vi "OP_Print_TPS_cluster_20171030.vi"() -> ()   [LabVIEW 2013]
uses:
  <vilib>/addons/database/Connection.llb/DB Tools Open Connec (Path).vi
  <vilib>/addons/database/Connection.llb/Conn Execute.vi
  <vilib>/addons/database/Recordset.llb/Rec Fetch Recordset Data (R).vi
  <vilib>/addons/database/Recordset.llb/Rec Destroy - Connection.vi
  <userlib>/caLab/Private/Get_PV-1D.vi
  <userlib>/caLab/Private/Get_PV.vi
  <vilib>/addons/database/_DB Variant To Data/Database Variant To Data.xnode
  <vilib>/addons/database/NI_Database_API.lvlib
panel:
  out "EVENTs":i32
  out "check loop":i32
  in  "Check period":i32=10 min=0 max=10
  out "Diff list":string[][](array[string])
  out "Program Start Time":dbl=3592021508.642459
  out "dT":u32=325
  out "x > y?":bool
  out "PV list":string[](array[string])=["LI-ES-CPS-01:SETMODE", "LI-ES-CPS-01:PULSEMODE", "LI-ES-BPS-01:SETU:GRID", "LI-ES-BPS-01:SETU:SBM", "LI-ES-BPS-01:SETU:MBM", "LI-RF-CAB-07:SET:MODE", "LI-RF-HVP-11:SET:U", "LI-RF-CAB-09:SET:MODE", "LI-RF-HVP-21:SET:U", "LI-RF-CAB-11:SET:MODE", "LI-RF-HVP-31:SET:U", "LI-RF-WGA-01:SET:POS", "LI-RF-WGA-02:SET:POS", "LI-RF-WGA-03:SET:POS", "LI-RF-SFT-01:SET:POS", "LI-RF-SFT-02:SET:POS", "LI-RF-SFT-03:SET:POS", "LI-RF-CTR-01:ES:SET:DEG", "LI-RF-CTR-01:SP:SET:DEG", "LI-RF-CTR-01:K123:SET:DEG", "LI-RF-CTR-01:K1:SET:DEG", "LI-RF-CTR-01:K3:SET:DEG", "LI-RF-AMP-01:SET:PWR", "LI-RF-AMP-02:SET:PWR", "LI-MA-SPS-01:SET:I", "LI-MA-SPS-02:SET:I", "LI-MA-SPS-03:SET:I", "LI-MA-SPS-04:SET:I", "LI-MA-SPS-05:SET:I", "LI-MA-SPS-06:SET:I", "LI-MA-SPS-07:SET:I", "LI-MA-SPS-08:SET:I", "LI-MA-SPS-09:SET:I", "LI-MA-SPS-10:SET:I", "LI-MA-SPS-11:SET:I", "LI-MA-SPS-12:SET:I", "LI-MA-SPS-13:SET:I", "LI-MA-SPS-14:SET:I", "LI-MA-SPS-15:SET:I", "LI-MA-SPS-16:SET:I", "LI-MA-STP-01:SET:I", "LI-MA-STP-02:SET:I", "LI-MA-STP-03:SET:I", "LI-MA-STP-04:SET:I", "LI-MA-STP-05:SET:I", "LI-MA-STP-06:SET:I", "LI-MA-STP-07:SET:I", "LI-MA-STP-08:SET:I", "LI-MA-STP-09:SET:I", "LI-MA-STP-10:SET:I", "LI-MA-STP-11:SET:I", "LI-MA-STP-12:SET:I", "LI-MA-STP-13:SET:I", "LI-MA-STP-14:SET:I", "LI-MA-STP-15:SET:I", "LI-MA-STP-16:SET:I", "LI-MA-QPS-01:SET:I", "LI-MA-QPS-02:SET:I", "LI-MA-QPS-03:SET:I", "LI-MA-QPS-04:SET:I", "LI-MA-QPS-05:SET:I", "LI-MA-QPS-06:SET:I", "CPCITM-TI-EVRTG:Pulse7DelaySet", "CPCITM-TI-EVRTG:Pulse7WidthSet", "CPCITM-TI-EVRTG:GTX7CtrlGTXPHSet", "CPCITM-TI-EVRTG:GTX7DlySet", "CPCITM-TI-EVRTG:Pulse6DelaySet", "CPCITM-TI-EVRTG:Pulse6WidthSet", "CPCITM-TI-EVRTG:GTX6CtrlGTXPHSet", "CPCITM-TI-EVRTG:GTX6DlySet", "CPCILI-TI-EVR:Pulse2DelaySet", "CPCILI-TI-EVR:Pulse2WidthSet", "CPCILI-TI-EVR:Pulse3DelaySet", "CPCILI-TI-EVR:Pulse3WidthSet", "CPCILI-TI-EVR:Pulse4DelaySet", "CPCILI-TI-EVR:Pulse4WidthSet", "CPCILI-TI-EVR:Pulse5DelaySet", "CPCILI-TI-EVR:Pulse5WidthSet", "CPCILI-TI-EVR:Pulse6DelaySet", "CPCILI-TI-EVR:Pulse6WidthSet", "CPCILI-TI-EVR:Pulse7DelaySet", "CPCILI-TI-EVR:Pulse7WidthSet", "CPCILI-TI-EVR:Pulse8DelaySet", "CPCILI-TI-EVR:Pulse8WidthSet", "CPCILI-TI-EVR:Pulse9DelaySet", "CPCILI-TI-EVR:Pulse9WidthSet", "CPCITM-TI-EVRTG:GTX6DlySet", "CPCITM-TI-EVRTG:GTX7DlySet", "LTB-PS-HC-1:setI", "LTB-PS-HC-2:setI", "LTB-PS-HC-3:setI", "LTB-PS-HC-4:setI", "LTB-PS-HC-5:setI", "LTB-PS-VC-1:setI", "LTB-PS-VC-2:setI", "LTB-PS-VC-3:setI", "LTB-PS-VC-4:setI", "LTB-PS-VC-5:setI", "LTB-PS-VC-6:setI", "LTB-PS-VC-7:setI", "LTB-PS-Q1A:setI", "LTB-PS-Q1B:setI", "LTB-PS-Q1C:setI", "LTB-PS-Q2A:setI", "LTB-PS-Q2B:setI", "LTB-PS-Q2C:setI", "LTB-PS-Q3A:setI", "LTB-PS-Q3B:setI", "LTB-PS-Q4A:setI", "LTB-PS-Q4B:setI", "LTB-PS-QQ:setI", "LTB-PS-BEND-1:setI", "LTB-PS-VC-2a:setI", "LTB-PS-HC-3a:setI", "LTB-PS-HC-3b:setI", "LTB-PS-HC-4a:setI", "LTB-PS-HC-5a:setI", "LI-DI-SLIT-motor:axis2Position1", "LI-DI-SLIT-motor:axis1Position1", "BR-PS-HC-101:setI", "BR-PS-HC-102:setI", "BR-PS-HC-103:setI", "BR-PS-HC-104:setI", "BR-PS-HC-105:setI", "BR-PS-HC-106:setI", "BR-PS-HC-107:setI", "BR-PS-HC-108:setI", "BR-PS-HC-109:setI", "BR-PS-HC-110:setI", "BR-PS-HC-201:setI", "BR-PS-HC-202:setI", "BR-PS-HC-203:setI", "BR-PS-HC-204:setI", "BR-PS-HC-205:setI", "BR-PS-HC-206:setI", "BR-PS-HC-207:setI", "BR-PS-HC-208:setI", "BR-PS-HC-209:setI", "BR-PS-HC-210:setI", "BR-PS-HC-301:setI", "BR-PS-HC-302:setI", "BR-PS-HC-303:setI", "BR-PS-HC-304:setI", "BR-PS-HC-305:setI", "BR-PS-HC-306:setI", "BR-PS-HC-307:setI", "BR-PS-HC-308:setI", "BR-PS-HC-309:setI", "BR-PS-HC-310:setI", "BR-PS-HC-401:setI", "BR-PS-HC-402:setI", "BR-PS-HC-403:setI", "BR-PS-HC-404:setI", "BR-PS-HC-405:setI", "BR-PS-HC-406:setI", "BR-PS-HC-407:setI", "BR-PS-HC-408:setI", "BR-PS-HC-409:setI", "BR-PS-HC-410:setI", "BR-PS-HC-501:setI", "BR-PS-HC-502:setI", "BR-PS-HC-503:setI", "BR-PS-HC-504:setI", "BR-PS-HC-505:setI", "BR-PS-HC-506:setI", "BR-PS-HC-507:setI", "BR-PS-HC-508:setI", "BR-PS-HC-509:setI", "BR-PS-HC-510:setI", "BR-PS-HC-601:setI", "BR-PS-HC-602:setI", "BR-PS-HC-603:setI", "BR-PS-HC-603a:setI", "BR-PS-HC-604:setI", "BR-PS-HC-605:setI", "BR-PS-HC-606:setI", "BR-PS-HC-606a:setI", "BR-PS-HC-607:setI", "BR-PS-HC-608:setI", "BR-PS-HC-609:setI", "BR-PS-HC-610:setI", "BR-PS-VC-101:setI", "BR-PS-VC-102:setI", "BR-PS-VC-103:setI", "BR-PS-VC-104:setI", "BR-PS-VC-105:setI", "BR-PS-VC-106:setI", "BR-PS-VC-201:setI", "BR-PS-VC-202:setI", "BR-PS-VC-203:setI", "BR-PS-VC-204:setI", "BR-PS-VC-205:setI", "BR-PS-VC-206:setI", "BR-PS-VC-301:setI", "BR-PS-VC-302:setI", "BR-PS-VC-303:setI", "BR-PS-VC-304:setI", "BR-PS-VC-305:setI", "BR-PS-VC-306:setI", "BR-PS-VC-401:setI", "BR-PS-VC-402:setI", "BR-PS-VC-403:setI", "BR-PS-VC-404:setI", "BR-PS-VC-405:setI", "BR-PS-VC-406:setI", "BR-PS-VC-501:setI", "BR-PS-VC-502:setI", "BR-PS-VC-503:setI", "BR-PS-VC-504:setI", "BR-PS-VC-505:setI", "BR-PS-VC-506:setI", "BR-PS-VC-601:setI", "BR-PS-VC-602:setI", "BR-PS-VC-602a:setI", "BR-PS-VC-603:setI", "BR-PS-VC-604:setI", "BR-PS-VC-604a:setI", "BR-PS-VC-605:setI", "BR-PS-VC-606:setI", "BR-PS-VC-100a:setI", "BR-PS-SD:setI", "BR-PS-SF:setI", "cpsc_027:AO:SLOW_SET:CH:1", "cpsc_037:AO:SLOW_SET:CH:3", "BR-RF-LLRF:setStationPhase", "TI-INJ-PROC:setTinj", "BR-PS-INJ-SE:setHV", "CPCIPM-TI-EVR:Pulse1DelaySet", "BR-PS-INJ-KI:setHV", "CPCIPM-TI-EVR:Pulse2DelaySet", "BR-PS-QF:setWfDC", "BR-PS-QM:setWfDC", "BR-PS-Q1:setWfDC", "BR-PS-Q2:setWfDC", "BR-PS-BEND:setWfDC", "BTS-PS-HC-1:setI", "BTS-PS-HC-2:setI", "BTS-PS-HC-3:setI", "BTS-PS-HC-4:setI", "BTS-PS-HC-5:setI", "BTS-PS-VC-2:setI", "BTS-PS-VC-3:setI", "BTS-PS-VC-4:setI", "BTS-PS-VC-5:setI", "BTS-PS-VC-6:setI", "BTS-PS-Q1A:setI", "BTS-PS-Q1B:setI", "BTS-PS-Q1C:setI", "BTS-PS-Q2A:setI", "BTS-PS-Q2B:setI", "BTS-PS-Q2C:setI", "BTS-PS-Q3A:setI", "BTS-PS-BEND-1:setI", "BTS-PS-BEND-2:setI", "BR-PS-EXT-K1:setHV", "BR-PS-EXT-K2:setHV", "SR-PS-INJ-SE1:setHV", "SR-PS-INJ-SE2:setHV", "SR-PS-INJ-K1:setHV", "SR-PS-INJ-K2:setHV", "SR-PS-INJ-K3:setHV", "SR-PS-INJ-K4:setHV", "CPCIPM-TI-EVR:Pulse4DelaySet", "CPCIPM-TI-EVR:Pulse5DelaySet", "CPCIPM-TI-EVR:Pulse3DelaySet", "CPCIPM-TI-EVR:Pulse6DelaySet", "CPCIPM-TI-EVR:Pulse7DelaySet", "T560:setADelay", "T560:setBDelay", "T560:setCDelay", "T560:setDDelay", "CPCIPM-TI-EVR:Pulse4DelaySet", "CPCIPM-TI-EVR:Pulse5DelaySet", "BR-PS-EXT-SE1:setHV", "BR-PS-EXT-SE2:setHV", "CPCIPM-TI-EVR:Pulse3DelaySet", "CPCIPM-TI-EVR:Pulse11DelaySet", "SR-PS-BEND:setI", "SR-PS-HC-011:setI", "SR-PS-HC-012:setI", "SR-PS-HC-013:setI", "SR-PS-HC-014:setI", "SR-PS-HC-015:setI", "SR-PS-HC-016:setI", "SR-PS-HC-017:setI", "SR-PS-HC-021:setI", "SR-PS-HC-022:setI", "SR-PS-HC-023:setI", "SR-PS-HC-024:setI", "SR-PS-HC-025:setI", "SR-PS-HC-026:setI", "SR-PS-HC-027:setI", "SR-PS-HC-031:setI", "SR-PS-HC-032:setI", "SR-PS-HC-033:setI", "SR-PS-HC-034:setI", "SR-PS-HC-035:setI", "SR-PS-HC-036:setI", "SR-PS-HC-037:setI", "SR-PS-HC-041:setI", "SR-PS-HC-042:setI", "SR-PS-HC-043:setI", "SR-PS-HC-044:setI", "SR-PS-HC-045:setI", "SR-PS-HC-046:setI", "SR-PS-HC-047:setI", "SR-PS-HC-051:setI", "SR-PS-HC-052:setI", "SR-PS-HC-053:setI", "SR-PS-HC-054:setI", "SR-PS-HC-055:setI", "SR-PS-HC-056:setI", "SR-PS-HC-057:setI", "SR-PS-HC-061:setI", "SR-PS-HC-062:setI", "SR-PS-HC-063:setI", "SR-PS-HC-064:setI", "SR-PS-HC-065:setI", "SR-PS-HC-066:setI", "SR-PS-HC-067:setI", "SR-PS-HC-071:setI", "SR-PS-HC-072:setI", "SR-PS-HC-073:setI", "SR-PS-HC-074:setI", "SR-PS-HC-075:setI", "SR-PS-HC-076:setI", "SR-PS-HC-077:setI", "SR-PS-HC-081:setI", "SR-PS-HC-082:setI", "SR-PS-HC-083:setI", "SR-PS-HC-084:setI", "SR-PS-HC-085:setI", "SR-PS-HC-086:setI", "SR-PS-HC-087:setI", "SR-PS-HC-091:setI", "SR-PS-HC-092:setI", "SR-PS-HC-093:setI", "SR-PS-HC-094:setI", "SR-PS-HC-095:setI", "SR-PS-HC-096:setI", "SR-PS-HC-097:setI", "SR-PS-HC-101:setI", "SR-PS-HC-102:setI", "SR-PS-HC-103:setI", "SR-PS-HC-104:setI", "SR-PS-HC-105:setI", "SR-PS-HC-106:setI", "SR-PS-HC-107:setI", "SR-PS-HC-111:setI", "SR-PS-HC-112:setI", "SR-PS-HC-113:setI", "SR-PS-HC-114:setI", "SR-PS-HC-115:setI", "SR-PS-HC-116:setI", "SR-PS-HC-117:setI", "SR-PS-HC-121:setI", "SR-PS-HC-122:setI", "SR-PS-HC-123:setI", "SR-PS-HC-124:setI", "SR-PS-HC-125:setI", "SR-PS-HC-126:setI", "SR-PS-HC-127:setI", "SR-PS-HC-131:setI", "SR-PS-HC-132:setI", "SR-PS-HC-133:setI", "SR-PS-HC-134:setI", "SR-PS-HC-135:setI", "SR-PS-HC-136:setI", "SR-PS-HC-137:setI", "SR-PS-HC-141:setI", "SR-PS-HC-142:setI", "SR-PS-HC-143:setI", "SR-PS-HC-144:setI", "SR-PS-HC-145:setI", "SR-PS-HC-146:setI", "SR-PS-HC-147:setI", "SR-PS-HC-151:setI", "SR-PS-HC-152:setI", "SR-PS-HC-153:setI", "SR-PS-HC-154:setI", "SR-PS-HC-155:setI", "SR-PS-HC-156:setI", "SR-PS-HC-157:setI", "SR-PS-HC-161:setI", "SR-PS-HC-162:setI", "SR-PS-HC-163:setI", "SR-PS-HC-164:setI", "SR-PS-HC-165:setI", "SR-PS-HC-166:setI", "SR-PS-HC-167:setI", "SR-PS-HC-171:setI", "SR-PS-HC-172:setI", "SR-PS-HC-173:setI", "SR-PS-HC-174:setI", "SR-PS-HC-175:setI", "SR-PS-HC-176:setI", "SR-PS-HC-177:setI", "SR-PS-HC-181:setI", "SR-PS-HC-182:setI", "SR-PS-HC-183:setI", "SR-PS-HC-184:setI", "SR-PS-HC-185:setI", "SR-PS-HC-186:setI", "SR-PS-HC-187:setI", "SR-PS-HC-191:setI", "SR-PS-HC-192:setI", "SR-PS-HC-193:setI", "SR-PS-HC-194:setI", "SR-PS-HC-195:setI", "SR-PS-HC-196:setI", "SR-PS-HC-197:setI", "SR-PS-HC-201:setI", "SR-PS-HC-202:setI", "SR-PS-HC-203:setI", "SR-PS-HC-204:setI", "SR-PS-HC-205:setI", "SR-PS-HC-206:setI", "SR-PS-HC-207:setI", "SR-PS-HC-211:setI", "SR-PS-HC-212:setI", "SR-PS-HC-213:setI", "SR-PS-HC-214:setI", "SR-PS-HC-215:setI", "SR-PS-HC-216:setI", "SR-PS-HC-217:setI", "SR-PS-HC-221:setI", "SR-PS-HC-222:setI", "SR-PS-HC-223:setI", "SR-PS-HC-224:setI", "SR-PS-HC-225:setI", "SR-PS-HC-226:setI", "SR-PS-HC-227:setI", "SR-PS-HC-231:setI", "SR-PS-HC-232:setI", "SR-PS-HC-233:setI", "SR-PS-HC-234:setI", "SR-PS-HC-235:setI", "SR-PS-HC-236:setI", "SR-PS-HC-237:setI", "SR-PS-HC-241:setI", "SR-PS-HC-242:setI", "SR-PS-HC-243:setI", "SR-PS-HC-244:setI", "SR-PS-HC-245:setI", "SR-PS-HC-246:setI", "SR-PS-HC-247:setI", "SR-PS-VC-011:setI", "SR-PS-VC-012:setI", "SR-PS-VC-013:setI", "SR-PS-VC-014:setI", "SR-PS-VC-015:setI", "SR-PS-VC-016:setI", "SR-PS-VC-017:setI", "SR-PS-VC-021:setI", "SR-PS-VC-022:setI", "SR-PS-VC-023:setI", "SR-PS-VC-024:setI", "SR-PS-VC-025:setI", "SR-PS-VC-026:setI", "SR-PS-VC-027:setI", "SR-PS-VC-031:setI", "SR-PS-VC-032:setI", "SR-PS-VC-033:setI", "SR-PS-VC-034:setI", "SR-PS-VC-035:setI", "SR-PS-VC-036:setI", "SR-PS-VC-037:setI", "SR-PS-VC-041:setI", "SR-PS-VC-042:setI", "SR-PS-VC-043:setI", "SR-PS-VC-044:setI", "SR-PS-VC-045:setI", "SR-PS-VC-046:setI", "SR-PS-VC-047:setI", "SR-PS-VC-051:setI", "SR-PS-VC-052:setI", "SR-PS-VC-053:setI", "SR-PS-VC-054:setI", "SR-PS-VC-055:setI", "SR-PS-VC-056:setI", "SR-PS-VC-057:setI", "SR-PS-VC-061:setI", "SR-PS-VC-062:setI", "SR-PS-VC-063:setI", "SR-PS-VC-064:setI", "SR-PS-VC-065:setI", "SR-PS-VC-066:setI", "SR-PS-VC-067:setI", "SR-PS-VC-071:setI", "SR-PS-VC-072:setI", "SR-PS-VC-073:setI", "SR-PS-VC-074:setI", "SR-PS-VC-075:setI", "SR-PS-VC-076:setI", "SR-PS-VC-077:setI", "SR-PS-VC-081:setI", "SR-PS-VC-082:setI", "SR-PS-VC-083:setI", "SR-PS-VC-084:setI", "SR-PS-VC-085:setI", "SR-PS-VC-086:setI", "SR-PS-VC-087:setI", "SR-PS-VC-091:setI", "SR-PS-VC-092:setI", "SR-PS-VC-093:setI", "SR-PS-VC-094:setI", "SR-PS-VC-095:setI", "SR-PS-VC-096:setI", "SR-PS-VC-097:setI", "SR-PS-VC-101:setI", "SR-PS-VC-102:setI", "SR-PS-VC-103:setI", "SR-PS-VC-104:setI", "SR-PS-VC-105:setI", "SR-PS-VC-106:setI", "SR-PS-VC-107:setI", "SR-PS-VC-111:setI", "SR-PS-VC-112:setI", "SR-PS-VC-113:setI", "SR-PS-VC-114:setI", "SR-PS-VC-115:setI", "SR-PS-VC-116:setI", "SR-PS-VC-117:setI", "SR-PS-VC-121:setI", "SR-PS-VC-122:setI", "SR-PS-VC-123:setI", "SR-PS-VC-124:setI", "SR-PS-VC-125:setI", "SR-PS-VC-126:setI", "SR-PS-VC-127:setI", "SR-PS-VC-131:setI", "SR-PS-VC-132:setI", "SR-PS-VC-133:setI", "SR-PS-VC-134:setI", "SR-PS-VC-135:setI", "SR-PS-VC-136:setI", "SR-PS-VC-137:setI", "SR-PS-VC-141:setI", "SR-PS-VC-142:setI", "SR-PS-VC-143:setI", "SR-PS-VC-144:setI", "SR-PS-VC-145:setI", "SR-PS-VC-146:setI", "SR-PS-VC-147:setI", "SR-PS-VC-151:setI", "SR-PS-VC-152:setI", "SR-PS-VC-153:setI", "SR-PS-VC-154:setI", "SR-PS-VC-155:setI", "SR-PS-VC-156:setI", "SR-PS-VC-157:setI", "SR-PS-VC-161:setI", "SR-PS-VC-162:setI", "SR-PS-VC-163:setI", "SR-PS-VC-164:setI", "SR-PS-VC-165:setI", "SR-PS-VC-166:setI", "SR-PS-VC-167:setI", "SR-PS-VC-171:setI", "SR-PS-VC-172:setI", "SR-PS-VC-173:setI", "SR-PS-VC-174:setI", "SR-PS-VC-175:setI", "SR-PS-VC-176:setI", "SR-PS-VC-177:setI", "SR-PS-VC-181:setI", "SR-PS-VC-182:setI", "SR-PS-VC-183:setI", "SR-PS-VC-184:setI", "SR-PS-VC-185:setI", "SR-PS-VC-186:setI", "SR-PS-VC-187:setI", "SR-PS-VC-191:setI", "SR-PS-VC-192:setI", "SR-PS-VC-193:setI", "SR-PS-VC-194:setI", "SR-PS-VC-195:setI", "SR-PS-VC-196:setI", "SR-PS-VC-197:setI", "SR-PS-VC-201:setI", "SR-PS-VC-202:setI", "SR-PS-VC-203:setI", "SR-PS-VC-204:setI", "SR-PS-VC-205:setI", "SR-PS-VC-206:setI", "SR-PS-VC-207:setI", "SR-PS-VC-211:setI", "SR-PS-VC-212:setI", "SR-PS-VC-213:setI", "SR-PS-VC-214:setI", "SR-PS-VC-215:setI", "SR-PS-VC-216:setI", "SR-PS-VC-217:setI", "SR-PS-VC-221:setI", "SR-PS-VC-222:setI", "SR-PS-VC-223:setI", "SR-PS-VC-224:setI", "SR-PS-VC-225:setI", "SR-PS-VC-226:setI", "SR-PS-VC-227:setI", "SR-PS-VC-231:setI", "SR-PS-VC-232:setI", "SR-PS-VC-233:setI", "SR-PS-VC-234:setI", "SR-PS-VC-235:setI", "SR-PS-VC-236:setI", "SR-PS-VC-237:setI", "SR-PS-VC-241:setI", "SR-PS-VC-242:setI", "SR-PS-VC-243:setI", "SR-PS-VC-244:setI", "SR-PS-VC-245:setI", "SR-PS-VC-246:setI", "SR-PS-VC-247:setI", "SR-PS-QL1-0101:setI", "SR-PS-QL2-0102:setI", "SR-PS-QL3-0103:setI", "SR-PS-QS4-0104:setI", "SR-PS-QS5-0105:setI", "SR-PS-QS5-0106:setI", "SR-PS-QS4-0107:setI", "SR-PS-QS3-0108:setI", "SR-PS-QS2-0109:setI", "SR-PS-QS1-0110:setI", "SR-PS-QS1-0201:setI", "SR-PS-QS2-0202:setI", "SR-PS-QS3-0203:setI", "SR-PS-QS4-0204:setI", "SR-PS-QS5-0205:setI", "SR-PS-QS5-0206:setI", "SR-PS-QS4-0207:setI", "SR-PS-QS3-0208:setI", "SR-PS-QS2-0209:setI", "SR-PS-QS1-0210:setI", "SR-PS-QS1-0301:setI", "SR-PS-QS2-0302:setI", "SR-PS-QS3-0303:setI", "SR-PS-QS4-0304:setI", "SR-PS-QS5-0305:setI", "SR-PS-QS5-0306:setI", "SR-PS-QS4-0307:setI", "SR-PS-QS3-0308:setI", "SR-PS-QS2-0309:setI", "SR-PS-QS1-0310:setI", "SR-PS-QS1-0401:setI", "SR-PS-QS2-0402:setI", "SR-PS-QS3-0403:setI", "SR-PS-QS4-0404:setI", "SR-PS-QS5-0405:setI", "SR-PS-QS5-0406:setI", "SR-PS-QS4-0407:setI", "SR-PS-QL3-0408:setI", "SR-PS-QL2-0409:setI", "SR-PS-QL1-0410:setI", "SR-PS-QL1-0501:setI", "SR-PS-QL2-0502:setI", "SR-PS-QL3-0503:setI", "SR-PS-QS4-0504:setI", "SR-PS-QS5-0505:setI", "SR-PS-QS5-0506:setI", "SR-PS-QS4-0507:setI", "SR-PS-QS3-0508:setI", "SR-PS-QS2-0509:setI", "SR-PS-QS1-0510:setI", "SR-PS-QS1-0601:setI", "SR-PS-QS2-0602:setI", "SR-PS-QS3-0603:setI", "SR-PS-QS4-0604:setI", "SR-PS-QS5-0605:setI", "SR-PS-QS5-0606:setI", "SR-PS-QS4-0607:setI", "SR-PS-QS3-0608:setI", "SR-PS-QS2-0609:setI", "SR-PS-QS1-0610:setI", "SR-PS-QS1-0701:setI", "SR-PS-QS2-0702:setI", "SR-PS-QS3-0703:setI", "SR-PS-QS4-0704:setI", "SR-PS-QS5-0705:setI", "SR-PS-QS5-0706:setI", "SR-PS-QS4-0707:setI", "SR-PS-QS3-0708:setI", "SR-PS-QS2-0709:setI", "SR-PS-QS1-0710:setI", "SR-PS-QS1-0801:setI", "SR-PS-QS2-0802:setI", "SR-PS-QS3-0803:setI", "SR-PS-QS4-0804:setI", "SR-PS-QS5-0805:setI", "SR-PS-QS5-0806:setI", "SR-PS-QS4-0807:setI", "SR-PS-QL3-0808:setI", "SR-PS-QL2-0809:setI", "SR-PS-QL1-0810:setI", "SR-PS-QL1-0901:setI", "SR-PS-QL2-0902:setI", "SR-PS-QL3-0903:setI", "SR-PS-QS4-0904:setI", "SR-PS-QS5-0905:setI", "SR-PS-QS5-0906:setI", "SR-PS-QS4-0907:setI", "SR-PS-QS3-0908:setI", "SR-PS-QS2-0909:setI", "SR-PS-QS1-0910:setI", "SR-PS-QS1-1001:setI", "SR-PS-QS2-1002:setI", "SR-PS-QS3-1003:setI", "SR-PS-QS4-1004:setI", "SR-PS-QS5-1005:setI", "SR-PS-QS5-1006:setI", "SR-PS-QS4-1007:setI", "SR-PS-QS3-1008:setI", "SR-PS-QS2-1009:setI", "SR-PS-QS1-1010:setI", "SR-PS-QS1-1101:setI", "SR-PS-QS2-1102:setI", "SR-PS-QS3-1103:setI", "SR-PS-QS4-1104:setI", "SR-PS-QS5-1105:setI", "SR-PS-QS5-1106:setI", "SR-PS-QS4-1107:setI", "SR-PS-QS3-1108:setI", "SR-PS-QS2-1109:setI", "SR-PS-QS1-1110:setI", "SR-PS-QS1-1201:setI", "SR-PS-QS2-1202:setI", "SR-PS-QS3-1203:setI", "SR-PS-QS4-1204:setI", "SR-PS-QS5-1205:setI", "SR-PS-QS5-1206:setI", "SR-PS-QS4-1207:setI", "SR-PS-QL3-1208:setI", "SR-PS-QL2-1209:setI", "SR-PS-QL1-1210:setI", "SR-PS-QL1-1301:setI", "SR-PS-QL2-1302:setI", "SR-PS-QL3-1303:setI", "SR-PS-QS4-1304:setI", "SR-PS-QS5-1305:setI", "SR-PS-QS5-1306:setI", "SR-PS-QS4-1307:setI", "SR-PS-QS3-1308:setI", "SR-PS-QS2-1309:setI", "SR-PS-QS1-1310:setI", "SR-PS-QS1-1401:setI", "SR-PS-QS2-1402:setI", "SR-PS-QS3-1403:setI", "SR-PS-QS4-1404:setI", "SR-PS-QS5-1405:setI", "SR-PS-QS5-1406:setI", "SR-PS-QS4-1407:setI", "SR-PS-QS3-1408:setI", "SR-PS-QS2-1409:setI", "SR-PS-QS1-1410:setI", "SR-PS-QS1-1501:setI", "SR-PS-QS2-1502:setI", "SR-PS-QS3-1503:setI", "SR-PS-QS4-1504:setI", "SR-PS-QS5-1505:setI", "SR-PS-QS5-1506:setI", "SR-PS-QS4-1507:setI", "SR-PS-QS3-1508:setI", "SR-PS-QS2-1509:setI", "SR-PS-QS1-1510:setI", "SR-PS-QS1-1601:setI", "SR-PS-QS2-1602:setI", "SR-PS-QS3-1603:setI", "SR-PS-QS4-1604:setI", "SR-PS-QS5-1605:setI", "SR-PS-QS5-1606:setI", "SR-PS-QS4-1607:setI", "SR-PS-QL3-1608:setI", "SR-PS-QL2-1609:setI", "SR-PS-QL1-1610:setI", "SR-PS-QL1-1701:setI", "SR-PS-QL2-1702:setI", "SR-PS-QL3-1703:setI", "SR-PS-QS4-1704:setI", "SR-PS-QS5-1705:setI", "SR-PS-QS5-1706:setI", "SR-PS-QS4-1707:setI", "SR-PS-QS3-1708:setI", "SR-PS-QS2-1709:setI", "SR-PS-QS1-1710:setI", "SR-PS-QS1-1801:setI", "SR-PS-QS2-1802:setI", "SR-PS-QS3-1803:setI", "SR-PS-QS4-1804:setI", "SR-PS-QS5-1805:setI", "SR-PS-QS5-1806:setI", "SR-PS-QS4-1807:setI", "SR-PS-QS3-1808:setI", "SR-PS-QS2-1809:setI", "SR-PS-QS1-1810:setI", "SR-PS-QS1-1901:setI", "SR-PS-QS2-1902:setI", "SR-PS-QS3-1903:setI", "SR-PS-QS4-1904:setI", "SR-PS-QS5-1905:setI", "SR-PS-QS5-1906:setI", "SR-PS-QS4-1907:setI", "SR-PS-QS3-1908:setI", "SR-PS-QS2-1909:setI", "SR-PS-QS1-1910:setI", "SR-PS-QS1-2001:setI", "SR-PS-QS2-2002:setI", "SR-PS-QS3-2003:setI", "SR-PS-QS4-2004:setI", "SR-PS-QS5-2005:setI", "SR-PS-QS5-2006:setI", "SR-PS-QS4-2007:setI", "SR-PS-QL3-2008:setI", "SR-PS-QL2-2009:setI", "SR-PS-QL1-2010:setI", "SR-PS-QL1-2101:setI", "SR-PS-QL2-2102:setI", "SR-PS-QL3-2103:setI", "SR-PS-QS4-2104:setI", "SR-PS-QS5-2105:setI", "SR-PS-QS5-2106:setI", "SR-PS-QS4-2107:setI", "SR-PS-QS3-2108:setI", "SR-PS-QS2-2109:setI", "SR-PS-QS1-2110:setI", "SR-PS-QS1-2201:setI", "SR-PS-QS2-2202:setI", "SR-PS-QS3-2203:setI", "SR-PS-QS4-2204:setI", "SR-PS-QS5-2205:setI", "SR-PS-QS5-2206:setI", "SR-PS-QS4-2207:setI", "SR-PS-QS3-2208:setI", "SR-PS-QS2-2209:setI", "SR-PS-QS1-2210:setI", "SR-PS-QS1-2301:setI", "SR-PS-QS2-2302:setI", "SR-PS-QS3-2303:setI", "SR-PS-QS4-2304:setI", "SR-PS-QS5-2305:setI", "SR-PS-QS5-2306:setI", "SR-PS-QS4-2307:setI", "SR-PS-QS3-2308:setI", "SR-PS-QS2-2309:setI", "SR-PS-QS1-2310:setI", "SR-PS-QS1-2401:setI", "SR-PS-QS2-2402:setI", "SR-PS-QS3-2403:setI", "SR-PS-QS4-2404:setI", "SR-PS-QS5-2405:setI", "SR-PS-QS5-2406:setI", "SR-PS-QS4-2407:setI", "SR-PS-QL3-2408:setI", "SR-PS-QL2-2409:setI", "SR-PS-QL1-2410:setI", "SR-PS-S1-011:setI", "SR-PS-S2-012:setI", "SR-PS-SD-013:setI", "SR-PS-SF-014:setI", "SR-PS-SD-015:setI", "SR-PS-S4-016:setI", "SR-PS-S3-017:setI", "SR-PS-S5-021:setI", "SR-PS-S6-022:setI", "SR-PS-SD-023:setI", "SR-PS-SF-024:setI", "SR-PS-SD-025:setI", "SR-PS-S6-026:setI", "SR-PS-S5-027:setI", "SR-PS-S5-031:setI", "SR-PS-S6-032:setI", "SR-PS-SD-033:setI", "SR-PS-SF-034:setI", "SR-PS-SD-035:setI", "SR-PS-S6-036:setI", "SR-PS-S5-037:setI", "SR-PS-S3-041:setI", "SR-PS-S4-042:setI", "SR-PS-SD-043:setI", "SR-PS-SF-044:setI", "SR-PS-SD-045:setI", "SR-PS-S2-046:setI", "SR-PS-S1-047:setI", "SR-PS-S1-051:setI", "SR-PS-S2-052:setI", "SR-PS-SD-053:setI", "SR-PS-SF-054:setI", "SR-PS-SD-055:setI", "SR-PS-S4-056:setI", "SR-PS-S3-057:setI", "SR-PS-S5-061:setI", "SR-PS-S6-062:setI", "SR-PS-SD-063:setI", "SR-PS-SF-064:setI", "SR-PS-SD-065:setI", "SR-PS-S6-066:setI", "SR-PS-S5-067:setI", "SR-PS-S5-071:setI", "SR-PS-S6-072:setI", "SR-PS-SD-073:setI", "SR-PS-SF-074:setI", "SR-PS-SD-075:setI", "SR-PS-S6-076:setI", "SR-PS-S5-077:setI", "SR-PS-S3-081:setI", "SR-PS-S4-082:setI", "SR-PS-SD-083:setI", "SR-PS-SF-084:setI", "SR-PS-SD-085:setI", "SR-PS-S2-086:setI", "SR-PS-S1-087:setI", "SR-PS-S1-091:setI", "SR-PS-S2-092:setI", "SR-PS-SD-093:setI", "SR-PS-SF-094:setI", "SR-PS-SD-095:setI", "SR-PS-S4-096:setI", "SR-PS-S3-097:setI", "SR-PS-S5-101:setI", "SR-PS-S6-102:setI", "SR-PS-SD-103:setI", "SR-PS-SF-104:setI", "SR-PS-SD-105:setI", "SR-PS-S6-106:setI", "SR-PS-S5-107:setI", "SR-PS-S5-111:setI", "SR-PS-S6-112:setI", "SR-PS-SD-113:setI", "SR-PS-SF-114:setI", "SR-PS-SD-115:setI", "SR-PS-S6-116:setI", "SR-PS-S5-117:setI", "SR-PS-S3-121:setI", "SR-PS-S4-122:setI", "SR-PS-SD-123:setI", "SR-PS-SF-124:setI", "SR-PS-SD-125:setI", "SR-PS-S2-126:setI", "SR-PS-S1-127:setI", "SR-PS-S1-131:setI", "SR-PS-S2-132:setI", "SR-PS-SD-133:setI", "SR-PS-SF-134:setI", "SR-PS-SD-135:setI", "SR-PS-S4-136:setI", "SR-PS-S3-137:setI", "SR-PS-S5-141:setI", "SR-PS-S6-142:setI", "SR-PS-SD-143:setI", "SR-PS-SF-144:setI", "SR-PS-SD-145:setI", "SR-PS-S6-146:setI", "SR-PS-S5-147:setI", "SR-PS-S5-151:setI", "SR-PS-S6-152:setI", "SR-PS-SD-153:setI", "SR-PS-SF-154:setI", "SR-PS-SD-155:setI", "SR-PS-S6-156:setI", "SR-PS-S5-157:setI", "SR-PS-S3-161:setI", "SR-PS-S4-162:setI", "SR-PS-SD-163:setI", "SR-PS-SF-164:setI", "SR-PS-SD-165:setI", "SR-PS-S2-166:setI", "SR-PS-S1-167:setI", "SR-PS-S1-171:setI", "SR-PS-S2-172:setI", "SR-PS-SD-173:setI", "SR-PS-SF-174:setI", "SR-PS-SD-175:setI", "SR-PS-S4-176:setI", "SR-PS-S3-177:setI", "SR-PS-S5-181:setI", "SR-PS-S6-182:setI", "SR-PS-SD-183:setI", "SR-PS-SF-184:setI", "SR-PS-SD-185:setI", "SR-PS-S6-186:setI", "SR-PS-S5-187:setI", "SR-PS-S5-191:setI", "SR-PS-S6-192:setI", "SR-PS-SD-193:setI", "SR-PS-SF-194:setI", "SR-PS-SD-195:setI", "SR-PS-S6-196:setI", "SR-PS-S5-197:setI", "SR-PS-S3-201:setI", "SR-PS-S4-202:setI", "SR-PS-SD-203:setI", "SR-PS-SF-204:setI", "SR-PS-SD-205:setI", "SR-PS-S2-206:setI", "SR-PS-S1-207:setI", "SR-PS-S1-211:setI", "SR-PS-S2-212:setI", "SR-PS-SD-213:setI", "SR-PS-SF-214:setI", "SR-PS-SD-215:setI", "SR-PS-S4-216:setI", "SR-PS-S3-217:setI", "SR-PS-S5-221:setI", "SR-PS-S6-222:setI", "SR-PS-SD-223:setI", "SR-PS-SF-224:setI", "SR-PS-SD-225:setI", "SR-PS-S6-226:setI", "SR-PS-S5-227:setI", "SR-PS-S5-231:setI", "SR-PS-S6-232:setI", "SR-PS-SD-233:setI", "SR-PS-SF-234:setI", "SR-PS-SD-235:setI", "SR-PS-S6-236:setI", "SR-PS-S5-237:setI", "SR-PS-S3-241:setI", "SR-PS-S4-242:setI", "SR-PS-SD-243:setI", "SR-PS-SF-244:setI", "SR-PS-SD-245:setI", "SR-PS-S2-246:setI", "SR-PS-S1-247:setI", "SR-PS-SKEW-011:setI", "SR-PS-SKEW-012:setI", "SR-PS-SKEW-013:setI", "SR-PS-SKEW-014:setI", "SR-PS-SKEW-015:setI", "SR-PS-SKEW-016:setI", "SR-PS-SKEW-017:setI", "SR-PS-SKEW-021:setI", "SR-PS-SKEW-022:setI", "SR-PS-SKEW-023:setI", "SR-PS-SKEW-024:setI", "SR-PS-SKEW-025:setI", "SR-PS-SKEW-026:setI", "SR-PS-SKEW-027:setI", "SR-PS-SKEW-031:setI", "SR-PS-SKEW-032:setI", "SR-PS-SKEW-033:setI", "SR-PS-SKEW-034:setI", "SR-PS-SKEW-035:setI", "SR-PS-SKEW-036:setI", "SR-PS-SKEW-037:setI", "SR-PS-SKEW-041:setI", "SR-PS-SKEW-042:setI", "SR-PS-SKEW-043:setI", "SR-PS-SKEW-044:setI", "SR-PS-SKEW-045:setI", "SR-PS-SKEW-046:setI", "SR-PS-SKEW-047:setI", "SR-PS-SKEW-051:setI", "SR-PS-SKEW-052:setI", "SR-PS-SKEW-053:setI", "SR-PS-SKEW-054:setI", "SR-PS-SKEW-055:setI", "SR-PS-SKEW-056:setI", "SR-PS-SKEW-057:setI", "SR-PS-SKEW-061:setI", "SR-PS-SKEW-062:setI", "SR-PS-SKEW-063:setI", "SR-PS-SKEW-064:setI", "SR-PS-SKEW-065:setI", "SR-PS-SKEW-066:setI", "SR-PS-SKEW-067:setI", "SR-PS-SKEW-071:setI", "SR-PS-SKEW-072:setI", "SR-PS-SKEW-073:setI", "SR-PS-SKEW-074:setI", "SR-PS-SKEW-075:setI", "SR-PS-SKEW-076:setI", "SR-PS-SKEW-077:setI", "SR-PS-SKEW-081:setI", "SR-PS-SKEW-082:setI", "SR-PS-SKEW-083:setI", "SR-PS-SKEW-084:setI", "SR-PS-SKEW-085:setI", "SR-PS-SKEW-086:setI", "SR-PS-SKEW-087:setI", "SR-PS-SKEW-091:setI", "SR-PS-SKEW-092:setI", "SR-PS-SKEW-093:setI", "SR-PS-SKEW-094:setI", "SR-PS-SKEW-095:setI", "SR-PS-SKEW-096:setI", "SR-PS-SKEW-097:setI", "SR-PS-SKEW-101:setI", "SR-PS-SKEW-102:setI", "SR-PS-SKEW-103:setI", "SR-PS-SKEW-104:setI", "SR-PS-SKEW-105:setI", "SR-PS-SKEW-106:setI", "SR-PS-SKEW-107:setI", "SR-PS-SKEW-111:setI", "SR-PS-SKEW-112:setI", "SR-PS-SKEW-113:setI", "SR-PS-SKEW-114:setI", "SR-PS-SKEW-115:setI", "SR-PS-SKEW-116:setI", "SR-PS-SKEW-117:setI", "SR-PS-SKEW-121:setI", "SR-PS-SKEW-122:setI", "SR-PS-SKEW-123:setI", "SR-PS-SKEW-124:setI", "SR-PS-SKEW-125:setI", "SR-PS-SKEW-126:setI", "SR-PS-SKEW-127:setI", "SR-PS-SKEW-131:setI", "SR-PS-SKEW-132:setI", "SR-PS-SKEW-133:setI", "SR-PS-SKEW-134:setI", "SR-PS-SKEW-135:setI", "SR-PS-SKEW-136:setI", "SR-PS-SKEW-137:setI", "SR-PS-SKEW-141:setI", "SR-PS-SKEW-142:setI", "SR-PS-SKEW-143:setI", "SR-PS-SKEW-144:setI", "SR-PS-SKEW-145:setI", "SR-PS-SKEW-146:setI", "SR-PS-SKEW-147:setI", "SR-PS-SKEW-151:setI", "SR-PS-SKEW-152:setI", "SR-PS-SKEW-153:setI", "SR-PS-SKEW-154:setI", "SR-PS-SKEW-155:setI", "SR-PS-SKEW-156:setI", "SR-PS-SKEW-157:setI", "SR-PS-SKEW-161:setI", "SR-PS-SKEW-162:setI", "SR-PS-SKEW-163:setI", "SR-PS-SKEW-164:setI", "SR-PS-SKEW-165:setI", "SR-PS-SKEW-166:setI", "SR-PS-SKEW-167:setI", "SR-PS-SKEW-171:setI", "SR-PS-SKEW-172:setI", "SR-PS-SKEW-173:setI", "SR-PS-SKEW-174:setI", "SR-PS-SKEW-175:setI", "SR-PS-SKEW-176:setI", "SR-PS-SKEW-177:setI", "SR-PS-SKEW-181:setI", "SR-PS-SKEW-182:setI", "SR-PS-SKEW-183:setI", "SR-PS-SKEW-184:setI", "SR-PS-SKEW-185:setI", "SR-PS-SKEW-186:setI", "SR-PS-SKEW-187:setI", "SR-PS-SKEW-191:setI", "SR-PS-SKEW-192:setI", "SR-PS-SKEW-193:setI", "SR-PS-SKEW-194:setI", "SR-PS-SKEW-195:setI", "SR-PS-SKEW-196:setI", "SR-PS-SKEW-197:setI", "SR-PS-SKEW-201:setI", "SR-PS-SKEW-202:setI", "SR-PS-SKEW-203:setI", "SR-PS-SKEW-204:setI", "SR-PS-SKEW-205:setI", "SR-PS-SKEW-206:setI", "SR-PS-SKEW-207:setI", "SR-PS-SKEW-211:setI", "SR-PS-SKEW-212:setI", "SR-PS-SKEW-213:setI", "SR-PS-SKEW-214:setI", "SR-PS-SKEW-215:setI", "SR-PS-SKEW-216:setI", "SR-PS-SKEW-217:setI", "SR-PS-SKEW-221:setI", "SR-PS-SKEW-222:setI", "SR-PS-SKEW-223:setI", "SR-PS-SKEW-224:setI", "SR-PS-SKEW-225:setI", "SR-PS-SKEW-226:setI", "SR-PS-SKEW-227:setI", "SR-PS-SKEW-231:setI", "SR-PS-SKEW-232:setI", "SR-PS-SKEW-233:setI", "SR-PS-SKEW-234:setI", "SR-PS-SKEW-235:setI", "SR-PS-SKEW-236:setI", "SR-PS-SKEW-237:setI", "SR-PS-SKEW-241:setI", "SR-PS-SKEW-242:setI", "SR-PS-SKEW-243:setI", "SR-PS-SKEW-244:setI", "SR-PS-SKEW-245:setI", "SR-PS-SKEW-246:setI", "SR-PS-SKEW-247:setI", "SR-RF2-LLRF:setGapVoltage", "SR-RF2-LLRF:setStationPhase", "SR-RF3-LLRF:setGapVoltage", "SR-RF3-LLRF:setStationPhase", "SR-PS-DMB09-Q1:setI", "SR-PS-DMB09-Q2:setI", "SR-PS-DMB09-Q3:setI", "SR-PS-DMB25-Q1:setI", "SR-PS-DMB25-Q2:setI", "SR-PS-DMB25-Q3:setI", "SR-PS-DMB41-Q1:setI", "SR-PS-DMB41-Q2:setI", "SR-PS-DMB41-Q3:setI", "SR-PS-DMB09-HC1:setI", "SR-PS-DMB09-HC2:setI", "SR-PS-DMB09-VC1:setI", "SR-PS-DMB09-VC2:setI", "SR-PS-DMB25-HC1:setI", "SR-PS-DMB25-HC2:setI", "SR-PS-DMB25-VC1:setI", "SR-PS-DMB25-VC2:setI", "SR-PS-DMB41-HC1:setI", "SR-PS-DMB41-HC2:setI", "SR-PS-DMB41-VC1:setI", "SR-PS-DMB41-VC2:setI", "SR-ID-IU22-05:setGap", "SR-ID-IU22A-09:setGap", "SR-ID-IU22B-09:setGap", "SR-ID-IUT22-21:setGap", "SR-ID-IU22-23:setGap", "SR-ID-IU22A-25:setGap", "SR-ID-IU22B-25:setGap", "SR-ID-EPU48A-41:setGap", "SR-ID-EPU48A-41:setPhase", "SR-ID-EPU48B-41:setGap", "SR-ID-EPU48B-41:setPhase", "SR-ID-EPU46-45:setGap", "SR-ID-EPU46-45:setPhase", "SR-ID-IUT22-21:setGapTaper", "SR-ID-EPU48PS-41:setGap", "SR-ID-IU22-05:gapMotorOff", "SR-ID-IU22A-09:gapMotorOff", "SR-ID-IU22B-09:gapMotorOff", "SR-ID-IUT22-21:gapMotorOff", "SR-ID-IU22-23:gapMotorOff", "SR-ID-IU22A-25:gapMotorOff", "SR-ID-IU22B-25:gapMotorOff", "SR-ID-EPU48A-41:gapMotorOff", "SR-ID-EPU48B-41:gapMotorOff", "SR-ID-EPU46-45:gapMotorOff", "SR-ID-EPU48A-41:phaseMotorOff", "SR-ID-EPU48B-41:phaseMotorOff", "SR-ID-EPU46-45:phaseMotorOff", "SR-DI-FOFB-H:setStatus", "SR-DI-FOFB-V:setStatus", "IGPF:TPSX:FBCTRL", "IGPF:TPSY:FBCTRL", "TPS-SR-022:bpm3:ilk:enabled", "SR-DI-ANGLE-ILK:StatusX", "SR-DI-ANGLE-ILK:StatusY", "SR-DI-RF-FB:setStatus", "SR-ID-EPU48-TFF:status", "SR-ID-EPU48-CFF:status", "SR-ID-EPU46-TFF:status", "SR-ID-EPU46-CFF:status", "TI-INJ-PROC:TopupHiLowStart"]
  out "error out 5":errorcluster
  out "error out 4":errorcluster
  out "result":string="Beam Trip Events \nTatal Counts: 0"
  in  "last ? Hrs":dbl=12.0 min=1.0 max=24.0 step=1.0
  in  "Trip Evt B":bool
  in  "Show Check list Button":bool=TRUE
  in  "View Diff Button":bool
  in  "Save Lattice Button":bool
  in  "Refresh B":bool
  out "x = y?":bool
  out "NOW time":string="15:45:10"
  out "NOW date":string="2017/10/28"
  in  "Save Button":bool
  out "error out 3":errorcluster
  in  "stop":bool
  out "time kickeron":string="15:43:52"
  out "date kickeron":string="2017/10/28"
  out "Cluster":T1={"SR Fill Pattern"=array[864 elements], "Beam Current(mA"=320.769453, "Beam Lifetime(min)"=354.3939151043138, "Beamsize X(um)"=63.15189373514937, "Beamsize Y(um)"=38.03691397287648, "Tune X(from BPM)"=0.1487279843444227, "Tune Y(from BPM)"=0.2309197651663405, "Mode"="Top-Up", "NuX(from BBF) "=0.15142063757609414, "NuY(from BBF)"=0.22496346361412184, "IU22-23gap(R)"=7.0, "IU22-05gap(R)"=7.372, "IU22-05M"=TRUE, "IU22A-09gap(R)"=8.05, "IU22A-09M"=TRUE, "IU22B-09gap(R)"=40.001, "IU22B-09M"=FALSE, "IUT22-21gap(R)"=7.0, "IUT22-21M"=TRUE, "IU22-23M"=TRUE, "IU22A-25gap(R)"=7.0, "IU22A-25M"=TRUE, "IU22B-25gap(R)"=40.0, "IU22B-25M"=FALSE, "EPU48A-41gap(R)"=65.00055, "EPU48A-41gM"=FALSE, "EPU48B-41gap(R)"=27.450000000000003, "EPU48B-41gM"=TRUE, "EPU46-45gap(R)"=44.99850000000001, "EPU46-45gM"=FALSE, "EPU48A-41phase(R)"=0.00055, "EPU48B-41phase(R)"=0.0, "EPU46-45phase(R)"=5e-05, "Grid volt.(V)(S)"=33.0, "Gun mode"="MBM", "Mod.3 HV(kV)(S)"=35.37999999999996, "SR"="SR_DMB_2017_1024_0300LOCO.data", "BR"="Booster_2017_1023_0900.data", "Linac"="Linac_2017_0413_1015.data", "LTB"="LTB_JT_2017_0828_1050.data", "BTS"="BTS_2017_1023_0900.data", "RF2 remote"=TRUE, "RF2 OP mode"=TRUE, "RF2 phase.(S)"=-42.0, "RF Freq.(s)"=499655365.67399085, "RF2 gap volt.(S)"=1600.0, "RF3 remote"=TRUE, "RF3 OP mode"=TRUE, "RF3 phase.(S)"=1.1999999999999995, "RF3 gap volt.(S)"=1600.0, "BBF V"=TRUE, "BBF H"=TRUE, "BR ext. kicker1(kV)"=17.666, "BR ext. kicker2(kV)"=17.666, "BR ext. sep.1(V)"=322.14, "BR ext. sep.2(V)"=441.1, "BR inj. sep.(V)"=104.95, "BR inj. kicker(kV)"=13.449999999999969, "SR kicker4(kV)"=7.945, "SR kicker3(kV)"=8.02, "SR kicker2(kV)"=8.142, "SR kicker1(kV)"=8.1, "SR inj. sep.2(V)"=397.2, "SR inj. sep.1(V)"=398.04, "Bucket Start"=100.0, "Bucket Last"=450.0, "Bucket Step"=10.0, "Orbit ILK(P)"=TRUE, "IU22-05 Hutch Enable"=TRUE, "IU22A-09M Hutch Enable"=TRUE, "IUT22-21M Hutch Enable"=TRUE, "IU22-23M Hutch Enable"=TRUE, "IU22A-25M Hutch Enable"=TRUE, "EPU48A-41M Hutch Enable"=TRUE, "EPU46-45M Hutch Enable"=FALSE, "EPU46-45 FE Enable"=TRUE, "EPU48A-41 FE Enable"=TRUE, "IU22A-25 FE Enable"=TRUE, "IU22-23 FE Enable"=TRUE, "IUT22-21 FE Enable"=TRUE, "IU22A-09 FE Enable"=TRUE, "IU22-05 FE Enable"=TRUE, "EPU48A-41pM"=FALSE, "EPU48B-41pM"=TRUE, "EPU46-45pM"=FALSE, "Gun volt.(V)(S)"=23.5, "Width count"=75.0, "2ns step"=2.0, "10ps delay"=150.0, "phase shifter"=130.0015, "Taper"=1.0899999999999999, "05XBPMX 1"=14.279, "09XBPMX 1"=-34.837, "21XBPMX 1"=-36.466, "23XBPMX 1"=-38.547000000000004, "25XBPMX 1"=-40.08, "41XBPMX 1"=-513.551, "45XBPMX 1"=-12.86, "05XBPMY 1"=51.999, "09XBPMY 1"=30.004, "21XBPMY 1"=-4.771, "23XBPMY 1"=19.080000000000002, "25XBPMY 1"=-4.366, "41XBPMY 1"=309.241, "45XBPMY 1"=1.842, "FOFB H"="On", "FOFB V"="On", "time string"="15:45:09", "date"="2017/10/28", "date (last kicker ON)"="2017/10/28", "time string (last kicker ON)"="15:43:52", "Radio Buttons 2"=enum."absolute", "09XBPMX 2"="23.77", "09XBPMY 2"="-18.01", "05XBPMY 2"="-459.85", "05XBPMX 2"="-403.56", "21XBPMY 2"="-134.87", "21XBPMX 2"="-31.92", "23XBPMY 2"="233.82", "23XBPMX 2"="11.09", "25XBPMY 2"="5171.53", "25XBPMX 2"="2152.43", "41XBPMY 2"=" closed", "41XBPMX 2"=" PAB ", "45XBPMX 2"=" Hutch ", "45XBPMY 2"=" closed", "05 mode"="Follow", "09A mode"="Follow", "09B mode"="Follow", "21 mode"="Follow", "23 mode"="Follow", "25A mode"="Follow", "25B mode"="Follow", "41A mode"="Follow", "41B mode"="Follow", "46 mode"="Follow", "BeamCurrent History"={"BPM NO.  1_172"=array[4319 elements], array[4319 elements]}, "SR Beam Current in            hours"=12.0, "RF FB"="On", "BPMX Graph 2"={"Array of X axis  平均分配至各段"=[1.0, 1.1666666666666667, 1.3333333333333333, 1.5, 1.6666666666666665, 1.8333333333333333, 2.0, 2.142857142857143, 2.2857142857142856, 2.4285714285714284, 2.571428571428571, 2.7142857142857144, 2.857142857142857, 3.0, 3.142857142857143, 3.2857142857142856, 3.4285714285714284, 3.571428571428571, 3.7142857142857144, 3.857142857142857, 4.0, 4.125, 4.25, 4.375, 4.5, 4.625, 4.75, 4.875, 5.0, 5.125, 5.25, 5.375, 5.5, 5.625, 5.75, 5.875, 6.0, 6.142857142857143, 6.285714285714286, 6.428571428571429, 6.571428571428571, 6.714285714285714, 6.857142857142857, 7.0, 7.142857142857143, 7.285714285714286, 7.428571428571429, 7.571428571428571, 7.714285714285714, 7.857142857142857, 8.0, 8.142857142857142, 8.285714285714286, 8.428571428571429, 8.571428571428571, 8.714285714285714, 8.857142857142858, 9.0, 9.142857142857142, 9.285714285714286, 9.428571428571429, 9.571428571428571, 9.714285714285714, 9.857142857142858, 10.0, 10.142857142857142, 10.285714285714286, 10.428571428571429, 10.571428571428571, 10.714285714285714, 10.857142857142858, 11.0, 11.142857142857142, 11.285714285714286, 11.428571428571429, 11.571428571428571, 11.714285714285714, 11.857142857142858, 12.0, 12.125, 12.25, 12.375, 12.5, 12.625, 12.75, 12.875, 13.0, 13.125, 13.25, 13.375, 13.5, 13.625, 13.75, 13.875, 14.0, 14.142857142857142, 14.285714285714286, 14.428571428571429, 14.571428571428571, 14.714285714285714, 14.857142857142858, 15.0, 15.142857142857142, 15.285714285714286, 15.428571428571429, 15.571428571428571, 15.714285714285714, 15.857142857142858, 16.0, 16.142857142857142, 16.285714285714285, 16.428571428571427, 16.571428571428573, 16.714285714285715, 16.857142857142858, 17.0, 17.142857142857142, 17.285714285714285, 17.428571428571427, 17.571428571428573, 17.714285714285715, 17.857142857142858, 18.0, 18.142857142857142, 18.285714285714285, 18.428571428571427, 18.571428571428573, 18.714285714285715, 18.857142857142858, 19.0, 19.142857142857142, 19.285714285714285, 19.428571428571427, 19.571428571428573, 19.714285714285715, 19.857142857142858, 20.0, 20.125, 20.25, 20.375, 20.5, 20.625, 20.75, 20.875, 21.0, 21.125, 21.25, 21.375, 21.5, 21.625, 21.75, 21.875, 22.0, 22.142857142857142, 22.285714285714285, 22.428571428571427, 22.571428571428573, 22.714285714285715, 22.857142857142858, 23.0, 23.142857142857142, 23.285714285714285, 23.428571428571427, 23.571428571428573, 23.714285714285715, 23.857142857142858, 24.0, 24.166666666666668, 24.333333333333332, 24.5, 24.666666666666668, 24.833333333333332], [-104.35000000000001, -27.61, -81.269, 31.074, 6.062, -136.0, 99.494, -88.141, -46.889, -165.06900000000002, 6.021, -84.98, 1.75, -8.811, 8.532, -133.949, -96.848, 24.799, 5.059, -100.301, 144.643, -9.353, 21.271, -55.053000000000004, 53.308, 191.175, 158.868, 222.566, -123.501, -26.869, 534.8770000000001, 573.141, -225.076, -6.779, 120.711, -75.419, 85.256, 50.948, -59.4, -203.09900000000002, -20.847, 130.465, -112.508, 76.115, 15.039, -35.207, -105.659, -16.897000000000002, 68.91, -141.159, 107.378, 144.351, -55.053000000000004, -193.076, 129.21, 58.157000000000004, -162.566, 153.643, 28.149, 9.358, -84.211, 85.112, 22.422, -31.252, 89.379, -47.49, 54.793, -68.275, 110.611, -118.584, -371.90500000000003, -20.115000000000002, -329.103, -249.097, -146.817, 118.556, -25.749, -98.32600000000001, 55.269, -122.093, 50.967, -55.89, 88.019, -0.462, -608.1560000000001, -139.752, -304.999, -215.022, 93.23400000000001, 44.699, -65.235, 37.049, -3.491, -169.852, 216.458, 50.398, -92.285, -132.13400000000001, -12.869, 66.74, -188.53300000000002, 148.653, -5.112, -71.334, -177.681, 41.168, -12.532, -184.913, 194.919, 52.414, -75.628, -80.415, -36.814, 105.73100000000001, -104.36800000000001, 110.101, 49.669000000000004, -67.327, -157.372, 29.624000000000002, 22.156, -105.663, 47.799, 11.591000000000001, -75.285, -79.821, 34.331, -24.937, -158.703, 177.15, 200.872, -165.849, -60.67, 20.183, -15.311, -111.206, 107.58800000000001, 26.489, 69.547, -41.230000000000004, 81.986, 54.43, 253.076, 378.43600000000004, -117.003, -304.999, 131.013, 2.21, -158.435, 94.489, 63.017, -82.94500000000001, 99.147, 65.752, -37.261, -102.577, 41.791000000000004, 66.599, -163.73, 160.137, -7.15, -51.275, -140.353, 33.772, 54.203, -147.597, 128.696, 58.22, -47.144, -184.493, 56.980000000000004, 67.437, -54.227000000000004, -0.031]}, "BPMY Graph 2"={"Array of X axis  平均分配至各段"=[1.0, 1.1666666666666667, 1.3333333333333333, 1.5, 1.6666666666666665, 1.8333333333333333, 2.0, 2.142857142857143, 2.2857142857142856, 2.4285714285714284, 2.571428571428571, 2.7142857142857144, 2.857142857142857, 3.0, 3.142857142857143, 3.2857142857142856, 3.4285714285714284, 3.571428571428571, 3.7142857142857144, 3.857142857142857, 4.0, 4.125, 4.25, 4.375, 4.5, 4.625, 4.75, 4.875, 5.0, 5.125, 5.25, 5.375, 5.5, 5.625, 5.75, 5.875, 6.0, 6.142857142857143, 6.285714285714286, 6.428571428571429, 6.571428571428571, 6.714285714285714, 6.857142857142857, 7.0, 7.142857142857143, 7.285714285714286, 7.428571428571429, 7.571428571428571, 7.714285714285714, 7.857142857142857, 8.0, 8.142857142857142, 8.285714285714286, 8.428571428571429, 8.571428571428571, 8.714285714285714, 8.857142857142858, 9.0, 9.142857142857142, 9.285714285714286, 9.428571428571429, 9.571428571428571, 9.714285714285714, 9.857142857142858, 10.0, 10.142857142857142, 10.285714285714286, 10.428571428571429, 10.571428571428571, 10.714285714285714, 10.857142857142858, 11.0, 11.142857142857142, 11.285714285714286, 11.428571428571429, 11.571428571428571, 11.714285714285714, 11.857142857142858, 12.0, 12.125, 12.25, 12.375, 12.5, 12.625, 12.75, 12.875, 13.0, 13.125, 13.25, 13.375, 13.5, 13.625, 13.75, 13.875, 14.0, 14.142857142857142, 14.285714285714286, 14.428571428571429, 14.571428571428571, 14.714285714285714, 14.857142857142858, 15.0, 15.142857142857142, 15.285714285714286, 15.428571428571429, 15.571428571428571, 15.714285714285714, 15.857142857142858, 16.0, 16.142857142857142, 16.285714285714285, 16.428571428571427, 16.571428571428573, 16.714285714285715, 16.857142857142858, 17.0, 17.142857142857142, 17.285714285714285, 17.428571428571427, 17.571428571428573, 17.714285714285715, 17.857142857142858, 18.0, 18.142857142857142, 18.285714285714285, 18.428571428571427, 18.571428571428573, 18.714285714285715, 18.857142857142858, 19.0, 19.142857142857142, 19.285714285714285, 19.428571428571427, 19.571428571428573, 19.714285714285715, 19.857142857142858, 20.0, 20.125, 20.25, 20.375, 20.5, 20.625, 20.75, 20.875, 21.0, 21.125, 21.25, 21.375, 21.5, 21.625, 21.75, 21.875, 22.0, 22.142857142857142, 22.285714285714285, 22.428571428571427, 22.571428571428573, 22.714285714285715, 22.857142857142858, 23.0, 23.142857142857142, 23.285714285714285, 23.428571428571427, 23.571428571428573, 23.714285714285715, 23.857142857142858, 24.0, 24.166666666666668, 24.333333333333332, 24.5, 24.666666666666668, 24.833333333333332], [-143.858, -13.775, -13.785, 122.665, -66.475, 31.541, 2.118, -24.67, 28.275000000000002, 0.139, -36.578, -28.396, 48.925000000000004, 9.287, -3.412, 70.053, -21.479, 14.89, -7.234, 5.521, -3.164, 19.558, -37.538000000000004, 37.11, -77.159, -13.755, 77.63, 28.249000000000002, -209.114, -44.569, 92.851, 173.641, -70.156, -22.722, 17.795, -6.59, 25.654, -41.882, 53.713, 9.237, -26.164, 18.357, 63.695, -8.542, 5.183, -5.99, 9.508000000000001, -5.462, -29.446, 36.574, -52.552, 51.439, -48.502, 0.73, -23.836000000000002, -3.648, -9.628, -5.485, -68.679, 95.486, -62.041000000000004, 54.633, -58.791000000000004, 68.305, -49.682, 29.838, -8.459, 3.213, -5.561, -80.617, 58.144, 15.346, -158.743, -40.726, 5.259, 3.258, 41.128, -54.377, 5.01, 18.84, 11.403, -20.73, 21.792, -17.296, 27.29, 0.783, -6.804, -137.476, 116.70700000000001, -6.929, 17.846, -3.586, 11.754, 6.341, 0.292, -0.911, -8.236, -5.312, 14.939, -29.945, 30.573, -9.991, -49.344, 82.117, -27.45, 22.291, -6.636, -9.389, 10.034, -14.218, 14.215, -7.3, 12.409, -44.302, 50.197, -36.089, -9.120000000000001, 45.881, 14.836, -27.324, 10.765, -10.139, -33.252, 2.737, -9.99, -6.019, -53.329, -28.159, 2.676, -36.9, -2.372, 8.92, 13.599, -25.723, -16.436, 7.722, -0.088, -29.122, 32.814, -20.521, 30.155, -45.734, 36.611000000000004, 74.528, 68.482, -22.548000000000002, -31.398, 134.603, -45.587, -0.981, -40.156, 24.441, 20.477, -31.424, 19.5, -11.789, 16.394000000000002, -38.567, 9.523, 0.09, -0.058, -4.8500000000000005, 11.71, 25.637, -10.51, -18.101, -12.389000000000001, 95.417, -138.726, 30.355, 96.245, -48.666000000000004, 40.851, -0.71]}} {"SR Beam Current in            hours" min=1.0 max=24.0 step=1.0 format="%#_2f"; "45XBPMY 1" format="%#.2f"; "41XBPMY 1" format="%#.2f"; "25XBPMY 1" format="%#.2f"; "23XBPMY 1" format="%#.2f"; "21XBPMY 1" format="%#.2f"; "09XBPMY 1" format="%#.2f"; "05XBPMY 1" format="%#.2f"; "45XBPMX 1" format="%#.2f"; "41XBPMX 1" format="%#.2f"; "25XBPMX 1" format="%#.2f"; "23XBPMX 1" format="%#.2f"; "21XBPMX 1" format="%#.2f"; "09XBPMX 1" format="%#.2f"; "05XBPMX 1" format="%#.2f"; "Taper" format="%#.4f"; "phase shifter" format="%#.3f"; "10ps delay" format="%#.1f"; "2ns step" format="%#.1f"; "Width count" format="%#.1f"; "Gun volt.(V)(S)" format="%#.1f"; "Bucket Step" format="%#.2f"; "Bucket Last" format="%#.2f"; "Bucket Start" format="%#.2f"; "BR ext. kicker1(kV)" format="%#.2f"; "BR ext. kicker2(kV)" format="%#.2f"; "BR ext. sep.1(V)" format="%#.2f"; "BR ext. sep.2(V)" format="%#.2f"; "BR inj. sep.(V)" format="%#.3f"; "BR inj. kicker(kV)" format="%#.3f"; "SR kicker4(kV)" format="%#.2f"; "SR kicker3(kV)" format="%#.2f"; "SR kicker2(kV)" format="%#.2f"; "SR kicker1(kV)" format="%#.2f"; "SR inj. sep.2(V)" format="%#.2f"; "SR inj. sep.1(V)" format="%#.2f"; "RF3 gap volt.(S)" format="%#.0f"; "RF3 phase.(S)" format="%#.1f"; "RF2 gap volt.(S)" format="%#.0f"; "RF Freq.(s)" format="%#.1f"; "RF2 phase.(S)" format="%#.1f"; "Mod.3 HV(kV)(S)" format="%#.3f"; "Grid volt.(V)(S)" format="%#.1f"; "EPU46-45phase(R)" format="%#.4f"; "EPU48B-41phase(R)" format="%#.4f"; "EPU48A-41phase(R)" format="%#.4f"; "EPU46-45gap(R)" format="%#.4f"; "EPU48B-41gap(R)" format="%#.4f"; "EPU48A-41gap(R)" format="%#.4f"; "IU22B-25gap(R)" format="%#.4f"; "IU22A-25gap(R)" format="%#.4f"; "IUT22-21gap(R)" format="%#.4f"; "IU22B-09gap(R)" format="%#.4f"; "IU22A-09gap(R)" format="%#.4f"; "IU22-05gap(R)" format="%#.4f"; "IU22-23gap(R)" format="%#.4f"; "NuY(from BBF)" format="%#.4f"; "NuX(from BBF)" format="%#.4f"; "Tune Y(from BPM)" format="%#.4f"; "Tune X(from BPM)" format="%#.4f"; "Beamsize Y(um)" format="%#.2f"; "Beamsize X(um)" format="%#.2f"; "Beam Lifetime(min)" format="%#.3f"; "Beam Current(mA" format="%#.3f"}
  out "Value Array (number) 7":dbl[](array[numeric])=[12.934000000000001, 52.266, -35.292, 28.567, -37.62, -4.79, -40.34, 19.011, -41.612, -4.549, -513.989, 308.821, -13.981, 1.604, -404.43600000000004, -459.711, 23.794, -18.499, -32.093, -134.864, 10.407, 233.79500000000002, 2139.3830000000003, 5158.407, -27.067, 11.554, 134.031, -84.025]
  out "Value Array (number) 6":dbl[](array[numeric])=[7.372, 8.05, 40.001, 7.0, 7.0, 7.0, 40.0, 65.0006, 0.00065, 27.450000000000003, 0.0, 44.99850000000001, 5e-05, -1.0899999999999999, 130.0015]
  out "Value Array (number) 5":dbl[](array[numeric])=[499654641.19275105, 1.0, 0.0, 1335.005102558433, 1400.0, -56.1, 1.0, 0.0, 1362.1066276040413, 1400.0, 160.0]
  out "Value Array (number) 3":dbl[](array[numeric])=[0.0, 33.0, 23.5, 350.0, 35.37999999999996, 22485.0, 22485.0, 62.0, 75.0, 2.0, 2.0, 200.0, 150.0]
  out "Orbit ILK(A)":bool
  out "Orbit INT. Ang Active":bool
  out "Orbit INT.Ang. On":bool
  out "Orbit INT. Pos Active":bool
  out "Orbit INT.Pos. On":bool
  out "SBM volt.(S)":dbl=350.0 format="%#.1f"
  out "MBM volt.(S)":dbl=23.5 format="%#.1f"
  in  "Copy Button":bool
  in  "Print Button":bool
  in  "Help Button":bool
  in  "Open Button":bool
  out "BR Fill Pattern":dbl[](graph)
  # "TPS OP Handover Information"
  # "Additional Functions"
  # "Others"
  # "Time："
  # "Valve  Status"
  # "follow"
  # "SM Status"
  # "歷史電流圖\ntrip次數?\n輻射劑量?\n平均氣壓\n目前最高累計劑量\n最近一次觸發時BR電流及WCM數值"
  # "TFF"
  # "CFF"
  # "hrs"
  # "TPS Operational Handover Information v1.4.3"
  # "SR Status"
  # "Feedback"
  # "Pulse Mag"
  # "LINAC"
  # "x8(ns)"
  # "x2(ns)"
  # "x0.01(ns)"
  # "RF Status"
  # "Hz"
  # "(kV)"
  # "(kV)"
  # "Changeliang@LOP.NSRRC"
  # "SR Fill Pattern"
  # "Lattice Files in using"
  # "ID &Beamline (R)"
  # "mode"
  # "Gap\nmm"
  # "Motor"
  # "Phase"
  # "FE/Hutch"
  # "phase\nshifter"
  # "XBPM1X\num"
  # "XBPM1Y\num"
  # "XBPM2X\num"
  # "XBPM2Y\num"
  # "Note"
  # "05"
  # "09"
  # "Taper(enc)"
  # "21"
  # "23"
  # "25"
  # "41"
  # "45"
  # "SR Orbit"
  # "BPMX"
  # "BPMY"
  # "SR Beam Current History"
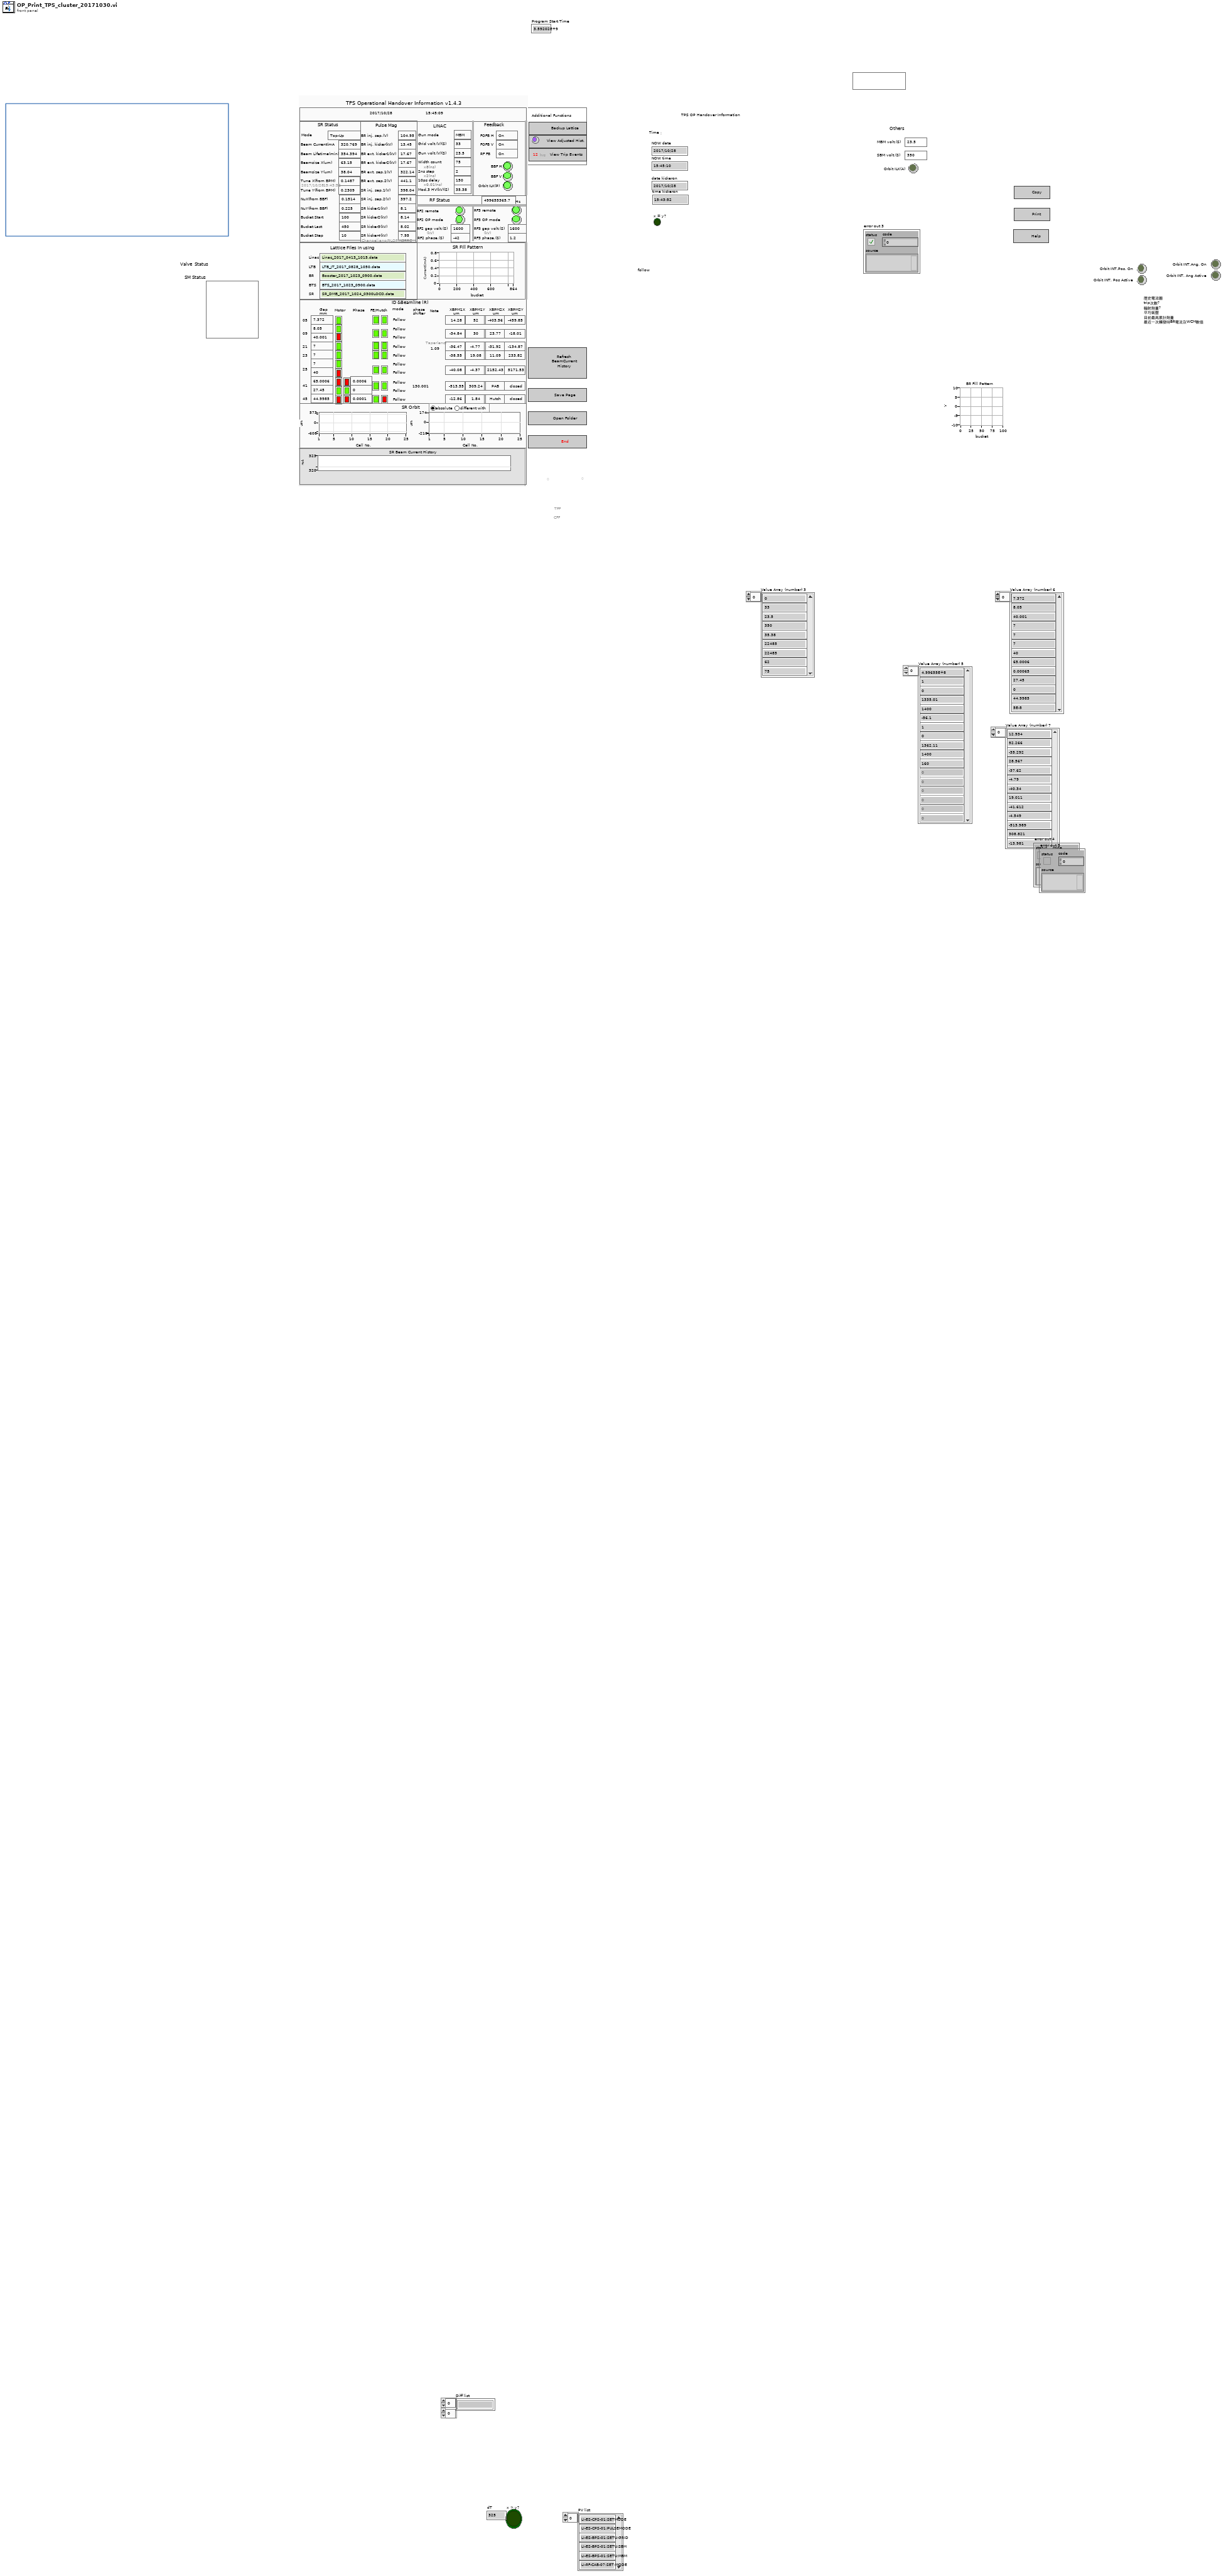
[diagram p1: front panel]
types:
  T1 = cluster{"SR Fill Pattern":dbl[], "Beam Current(mA":dbl, "Beam Lifetime(min)":dbl, "Beamsize X(um)":dbl, "Beamsize Y(um)":dbl, "Tune X(from BPM)":dbl, "Tune Y(from BPM)":dbl, "Mode":string, "NuX(from BBF) ":dbl, "NuY(from BBF)":dbl, "IU22-23gap(R)":dbl, "IU22-05gap(R)":dbl, "IU22-05M":bool, "IU22A-09gap(R)":dbl, "IU22A-09M":bool, "IU22B-09gap(R)":dbl, "IU22B-09M":bool, "IUT22-21gap(R)":dbl, "IUT22-21M":bool, "IU22-23M":bool, "IU22A-25gap(R)":dbl, "IU22A-25M":bool, "IU22B-25gap(R)":dbl, "IU22B-25M":bool, "EPU48A-41gap(R)":dbl, "EPU48A-41gM":bool, "EPU48B-41gap(R)":dbl, "EPU48B-41gM":bool, "EPU46-45gap(R)":dbl, "EPU46-45gM":bool, "EPU48A-41phase(R)":dbl, "EPU48B-41phase(R)":dbl, "EPU46-45phase(R)":dbl, "Grid volt.(V)(S)":dbl, "Gun mode":string, "Mod.3 HV(kV)(S)":dbl, "SR":string, "BR":string, "Linac":string, "LTB":string, "BTS":string, "RF2 remote":bool, "RF2 OP mode":bool, "RF2 phase.(S)":dbl, "RF Freq.(s)":dbl, "RF2 gap volt.(S)":dbl, "RF3 remote":bool, "RF3 OP mode":bool, "RF3 phase.(S)":dbl, "RF3 gap volt.(S)":dbl, "BBF V":bool, "BBF H":bool, "BR ext. kicker1(kV)":dbl, "BR ext. kicker2(kV)":dbl, "BR ext. sep.1(V)":dbl, "BR ext. sep.2(V)":dbl, "BR inj. sep.(V)":dbl, "BR inj. kicker(kV)":dbl, "SR kicker4(kV)":dbl, "SR kicker3(kV)":dbl, "SR kicker2(kV)":dbl, "SR kicker1(kV)":dbl, "SR inj. sep.2(V)":dbl, "SR inj. sep.1(V)":dbl, "Bucket Start":dbl, "Bucket Last":dbl, "Bucket Step":dbl, "Orbit ILK(P)":bool, "IU22-05 Hutch Enable":bool, "IU22A-09M Hutch Enable":bool, "IUT22-21M Hutch Enable":bool, "IU22-23M Hutch Enable":bool, "IU22A-25M Hutch Enable":bool, "EPU48A-41M Hutch Enable":bool, "EPU46-45M Hutch Enable":bool, "EPU46-45 FE Enable":bool, "EPU48A-41 FE Enable":bool, "IU22A-25 FE Enable":bool, "IU22-23 FE Enable":bool, "IUT22-21 FE Enable":bool, "IU22A-09 FE Enable":bool, "IU22-05 FE Enable":bool, "EPU48A-41pM":bool, "EPU48B-41pM":bool, "EPU46-45pM":bool, "Gun volt.(V)(S)":dbl, "Width count":dbl, "2ns step":dbl, "10ps delay":dbl, "phase shifter":dbl, "Taper":dbl, "05XBPMX 1":dbl, "09XBPMX 1":dbl, "21XBPMX 1":dbl, "23XBPMX 1":dbl, "25XBPMX 1":dbl, "41XBPMX 1":dbl, "45XBPMX 1":dbl, "05XBPMY 1":dbl, "09XBPMY 1":dbl, "21XBPMY 1":dbl, "23XBPMY 1":dbl, "25XBPMY 1":dbl, "41XBPMY 1":dbl, "45XBPMY 1":dbl, "FOFB H":string, "FOFB V":string, "time string":string, "date":string, "date (last kicker ON)":string, "time string (last kicker ON)":string, "Radio Buttons 2":enum32{"absolute", "different with"}, "09XBPMX 2":string, "09XBPMY 2":string, "05XBPMY 2":string, "05XBPMX 2":string, "21XBPMY 2":string, "21XBPMX 2":string, "23XBPMY 2":string, "23XBPMX 2":string, "25XBPMY 2":string, "25XBPMX 2":string, "41XBPMY 2":string, "41XBPMX 2":string, "45XBPMX 2":string, "45XBPMY 2":string, "05 mode":string, "09A mode":string, "09B mode":string, "21 mode":string, "23 mode":string, "25A mode":string, "25B mode":string, "41A mode":string, "41B mode":string, "46 mode":string, "BeamCurrent History":cluster{"BPM NO.  1_172":dbl[], dbl[]}, "SR Beam Current in            hours":dbl, "RF FB":string, "BPMX Graph 2":cluster{"Array of X axis  平均分配至各段":dbl[], dbl[]}, "BPMY Graph 2":cluster{"Array of X axis  平均分配至各段":dbl[], dbl[]}}
  T2 = typedef "NI_Database_API.lvlib/Conn ObjectReference.ctl" = refnum<k1>
  T3 = typedef "NI_Database_API.lvlib/Rec ObjectReference.ctl" = refnum<k1>
  T4 = typedef "imagedata.ctl" = cluster{"image type":i32, "image depth":i32, "image":u8[], "mask":u8[], "colors":u32[], "Rectangle":cluster{"left":i16, "top":i16, "right":i16, "bottom":i16}}
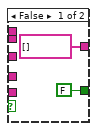
[diagram p2: hidden frame]
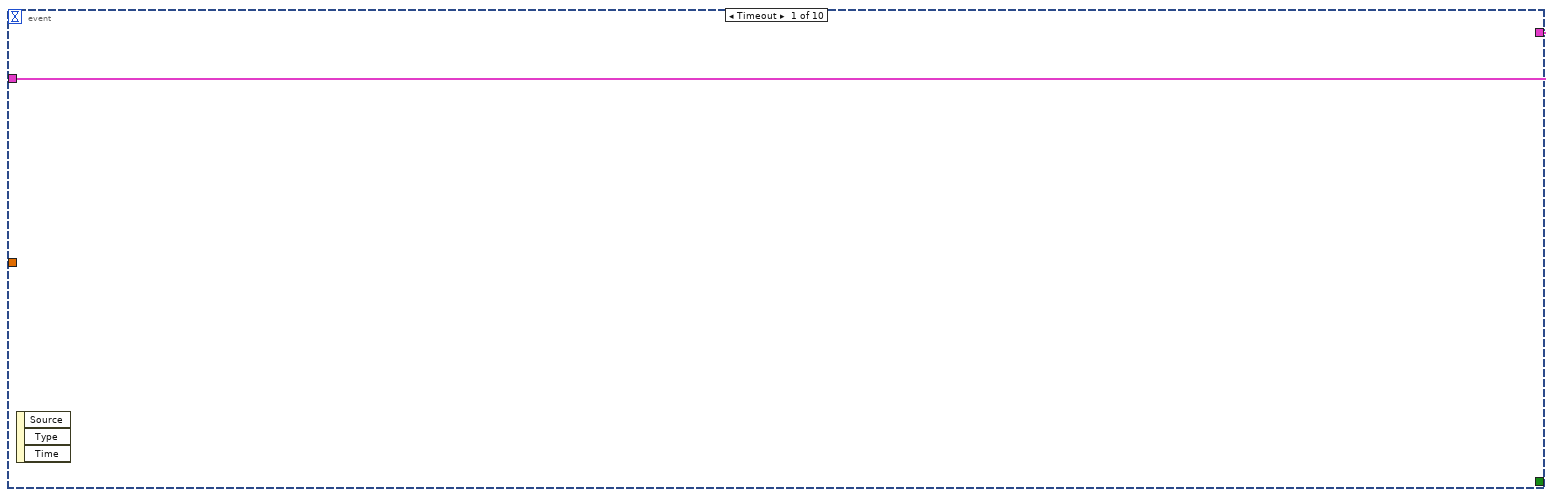
[diagram p4: hidden frame]
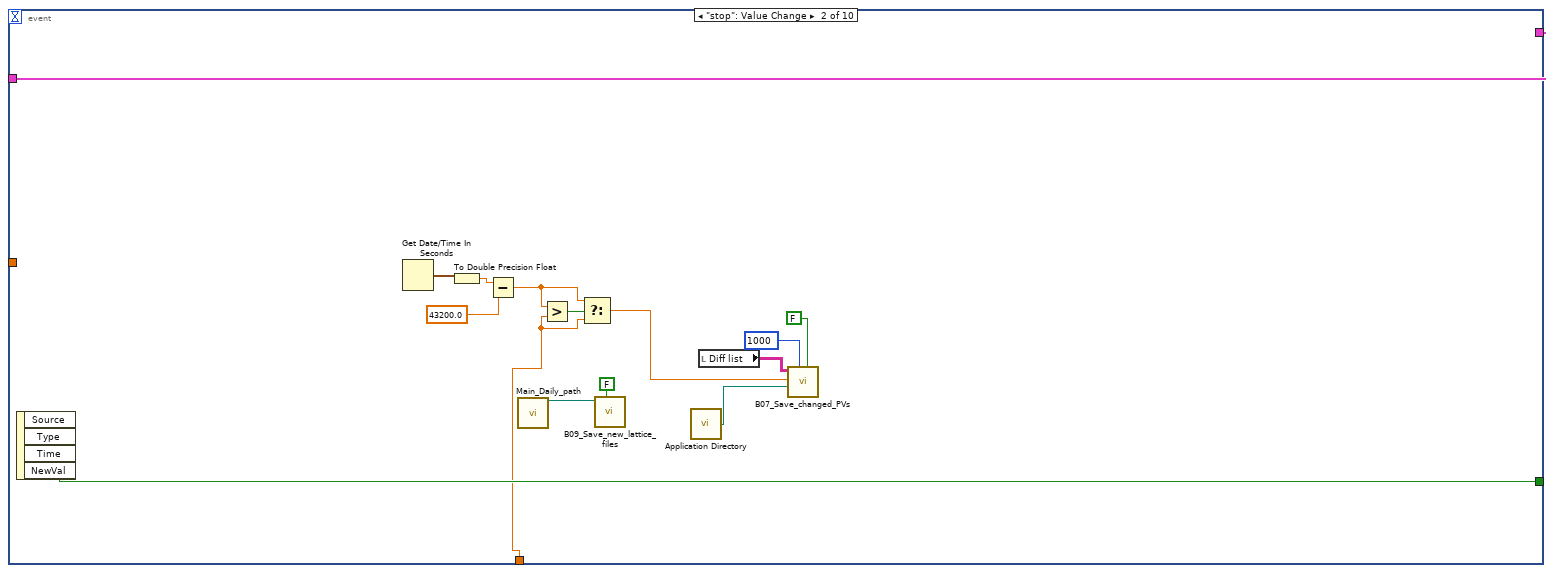
[diagram p5: hidden frame]
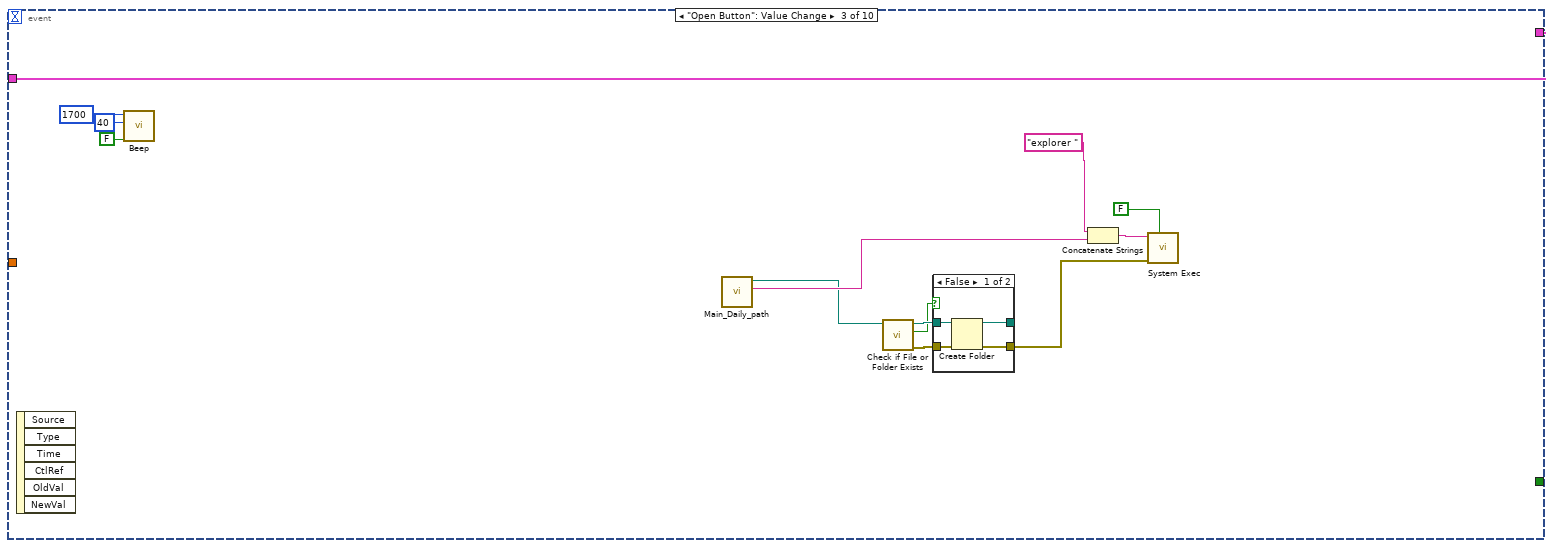
[diagram p6: hidden frame]
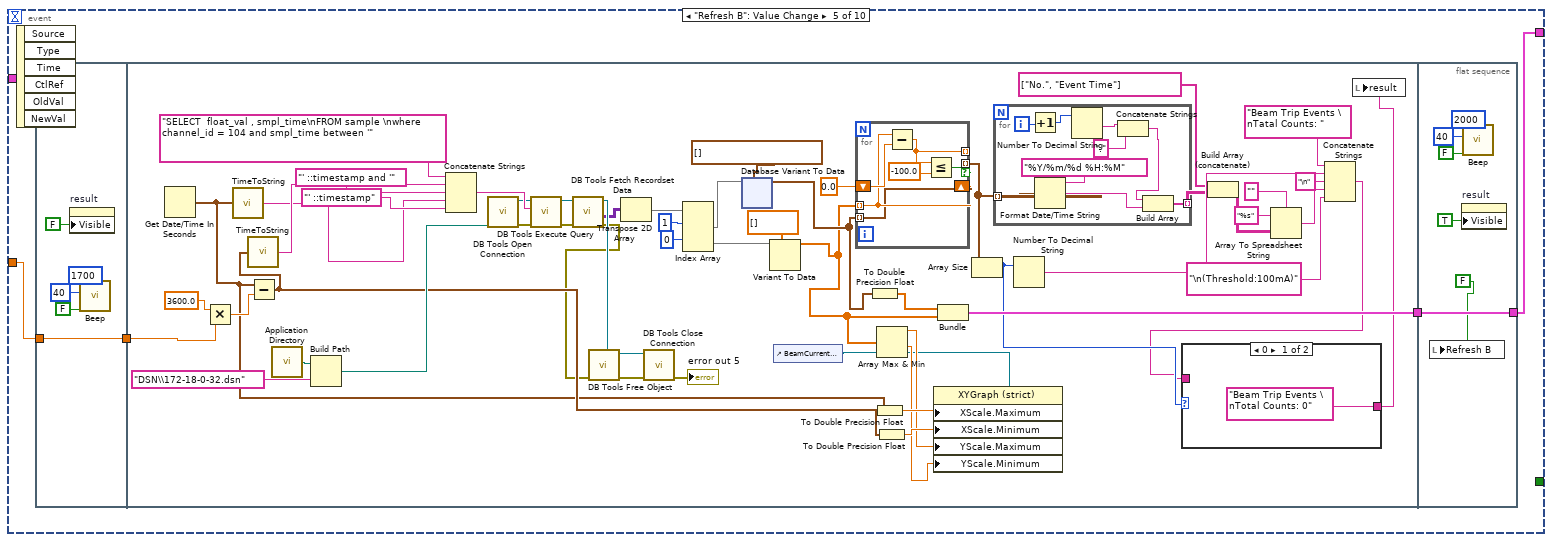
[diagram p9: hidden frame]
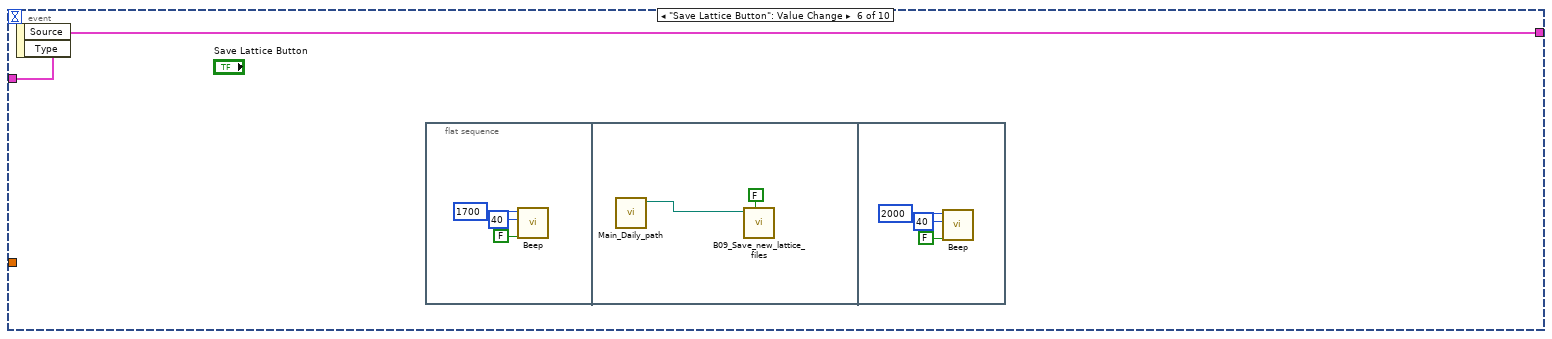
[diagram p11: hidden frame]
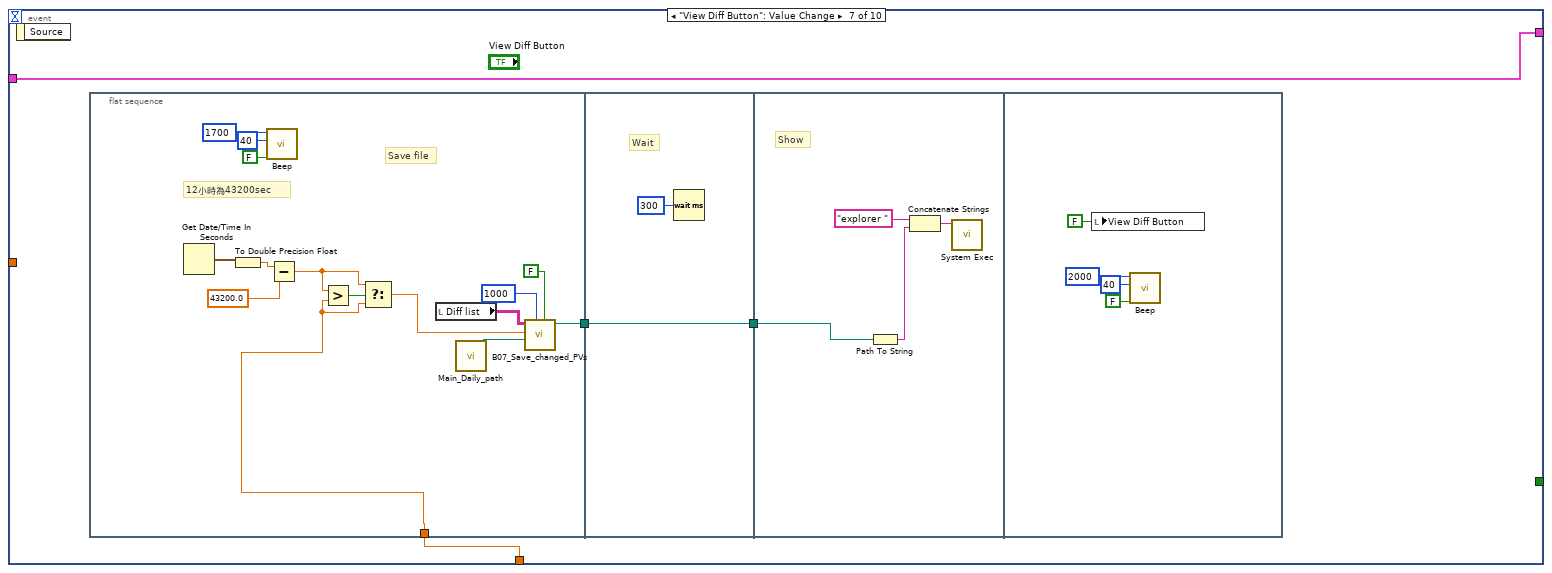
[diagram p12: hidden frame]
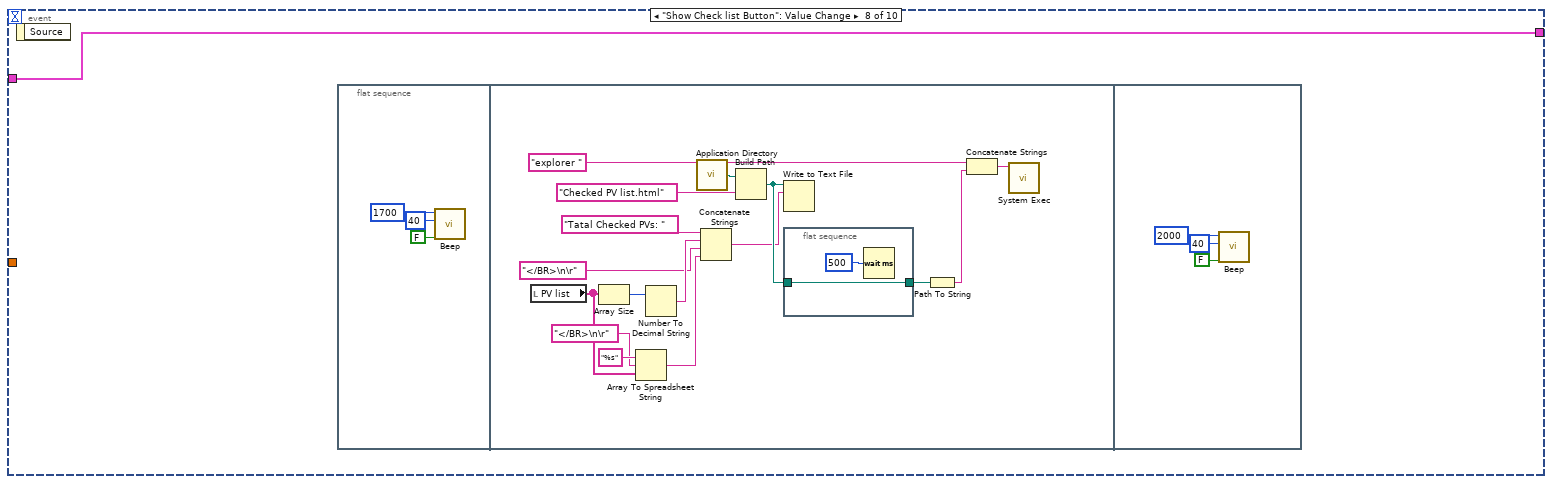
[diagram p13: hidden frame]
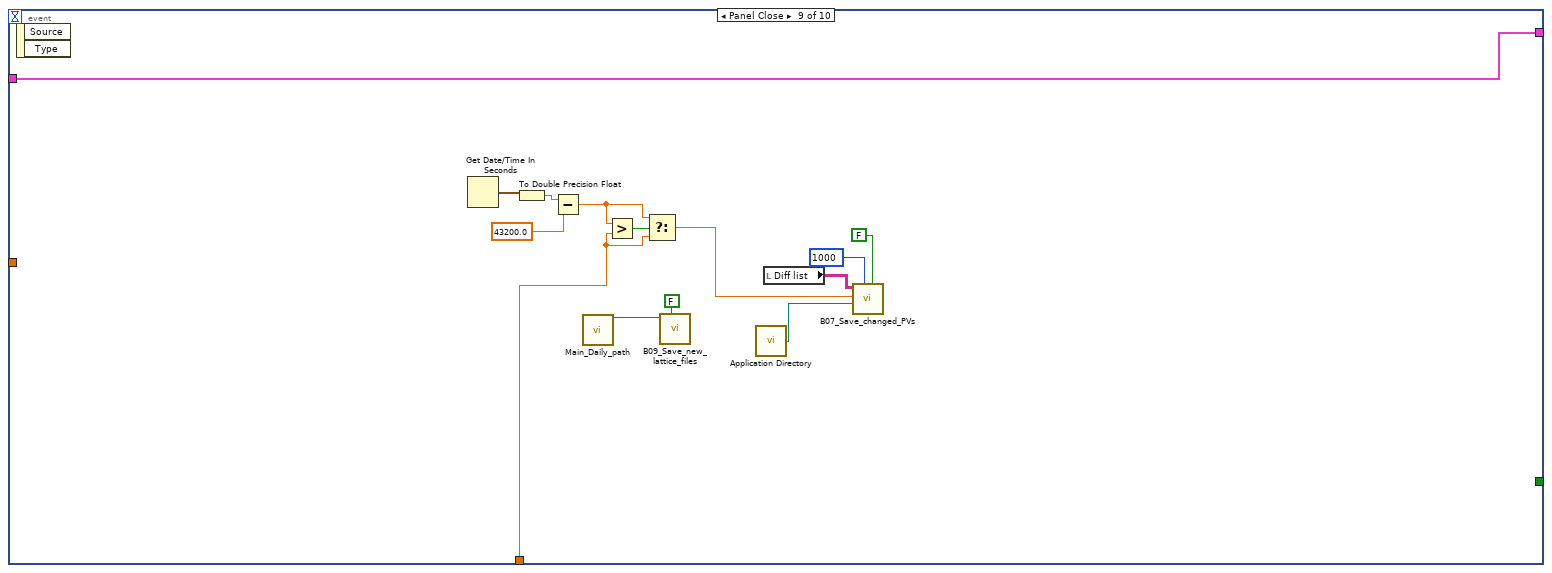
[diagram p14: hidden frame]
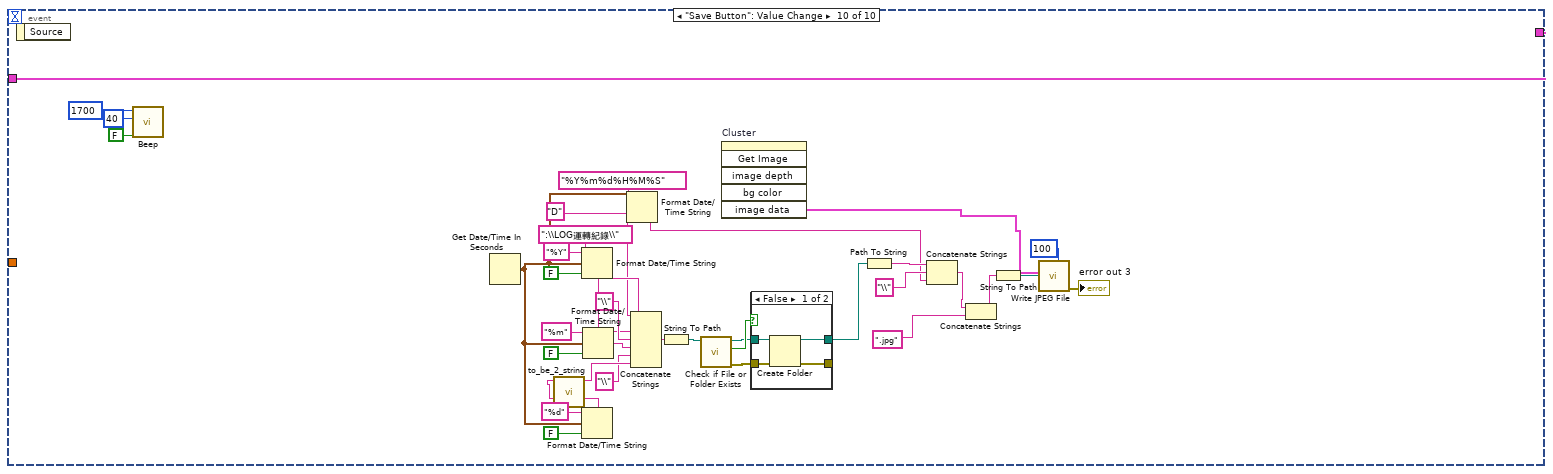
[diagram p15: hidden frame]
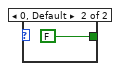
[diagram p17: hidden frame]
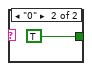
[diagram p18: hidden frame]
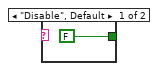
[diagram p19: hidden frame]
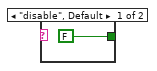
[diagram p20: hidden frame]
diagram:
  (unwired) "CPCITM-TI-EVRTG:GTX6CtrlGTXPHSet" ("regular expression")
  (unwired) "CPCITM-TI-EVRTG:GTX7CtrlGTXPHSet" ("regular expression")
  w1 = string[] ["LI-ES-CPS-01:SETMODE", "LI-ES-CPS-01:PULSEMODE", "LI-ES-BPS-01:SETU:GRID", "LI-ES-BPS-01:SETU:SBM", "LI-ES-BPS-01:SETU:MBM", "LI-RF-CAB-07:SET:MODE", "LI-RF-HVP-11:SET:U", "LI-RF-CAB-09:SET:MODE", "LI-RF-HVP-21:SET:U", "LI-RF-CAB-11:SET:MODE", "LI-RF-HVP-31:SET:U", "LI-RF-WGA-01:SET:POS", "LI-RF-WGA-02:SET:POS", "LI-RF-WGA-03:SET:POS", "LI-RF-SFT-01:SET:POS", "LI-RF-SFT-02:SET:POS", "LI-RF-SFT-03:SET:POS", "LI-RF-CTR-01:ES:SET:DEG", "LI-RF-CTR-01:SP:SET:DEG", "LI-RF-CTR-01:K123:SET:DEG", "LI-RF-CTR-01:K1:SET:DEG", "LI-RF-CTR-01:K3:SET:DEG", "LI-RF-AMP-01:SET:PWR", "LI-RF-AMP-02:SET:PWR", "LI-MA-SPS-01:SET:I", "LI-MA-SPS-02:SET:I", "LI-MA-SPS-03:SET:I", "LI-MA-SPS-04:SET:I", "LI-MA-SPS-05:SET:I", "LI-MA-SPS-06:SET:I", "LI-MA-SPS-07:SET:I", "LI-MA-SPS-08:SET:I", "LI-MA-SPS-09:SET:I", "LI-MA-SPS-10:SET:I", "LI-MA-SPS-11:SET:I", "LI-MA-SPS-12:SET:I", "LI-MA-SPS-13:SET:I", "LI-MA-SPS-14:SET:I", "LI-MA-SPS-15:SET:I", "LI-MA-SPS-16:SET:I", "LI-MA-STP-01:SET:I", "LI-MA-STP-02:SET:I", "LI-MA-STP-03:SET:I", "LI-MA-STP-04:SET:I", "LI-MA-STP-05:SET:I", "LI-MA-STP-06:SET:I", "LI-MA-STP-07:SET:I", "LI-MA-STP-08:SET:I", "LI-MA-STP-09:SET:I", "LI-MA-STP-10:SET:I", "LI-MA-STP-11:SET:I", "LI-MA-STP-12:SET:I", "LI-MA-STP-13:SET:I", "LI-MA-STP-14:SET:I", "LI-MA-STP-15:SET:I", "LI-MA-STP-16:SET:I", "LI-MA-QPS-01:SET:I", "LI-MA-QPS-02:SET:I", "LI-MA-QPS-03:SET:I", "LI-MA-QPS-04:SET:I", "LI-MA-QPS-05:SET:I", "LI-MA-QPS-06:SET:I", "CPCITM-TI-EVRTG:Pulse7DelaySet", "CPCITM-TI-EVRTG:Pulse7WidthSet", "CPCITM-TI-EVRTG:GTX7DlySet", "CPCITM-TI-EVRTG:Pulse6DelaySet", "CPCITM-TI-EVRTG:Pulse6WidthSet", "CPCITM-TI-EVRTG:GTX6DlySet", "CPCILI-TI-EVR:Pulse2DelaySet", "CPCILI-TI-EVR:Pulse2WidthSet", "CPCILI-TI-EVR:Pulse3DelaySet", "CPCILI-TI-EVR:Pulse3WidthSet", "CPCILI-TI-EVR:Pulse4DelaySet", "CPCILI-TI-EVR:Pulse4WidthSet", "CPCILI-TI-EVR:Pulse5DelaySet", "CPCILI-TI-EVR:Pulse5WidthSet", "CPCILI-TI-EVR:Pulse6DelaySet", "CPCILI-TI-EVR:Pulse6WidthSet", "CPCILI-TI-EVR:Pulse7DelaySet", "CPCILI-TI-EVR:Pulse7WidthSet", "CPCILI-TI-EVR:Pulse8DelaySet", "CPCILI-TI-EVR:Pulse8WidthSet", "CPCILI-TI-EVR:Pulse9DelaySet", "CPCILI-TI-EVR:Pulse9WidthSet", "CPCITM-TI-EVRTG:GTX6DlySet", "CPCITM-TI-EVRTG:GTX7DlySet"]  # PV nanes(LINAC) without 2 PHset
  w3 = string[] ["SR-ID-IU22-05:setGap", "SR-ID-IU22A-09:setGap", "SR-ID-IU22B-09:setGap", "SR-ID-IUT22-21:setGap", "SR-ID-IU22-23:setGap", "SR-ID-IU22A-25:setGap", "SR-ID-IU22B-25:setGap", "SR-ID-EPU48A-41:setGap", "SR-ID-EPU48A-41:setPhase", "SR-ID-EPU48B-41:setGap", "SR-ID-EPU48B-41:setPhase", "SR-ID-EPU46-45:setGap", "SR-ID-EPU46-45:setPhase", "SR-ID-IUT22-21:setGapTaper", "SR-ID-EPU48PS-41:setGap"]  # PV nanes(ID gap_phase_Taper_)
  w14 = string[] ["TI-INJ-PROC:TopupHiLowStart"]  # PV nanes(Others)
  w13 = string[] ["SR-PS-BEND:setI", "SR-PS-HC-011:setI", "SR-PS-HC-012:setI", "SR-PS-HC-013:setI", "SR-PS-HC-014:setI", "SR-PS-HC-015:setI", "SR-PS-HC-016:setI", "SR-PS-HC-017:setI", "SR-PS-HC-021:setI", "SR-PS-HC-022:setI", "SR-PS-HC-023:setI", "SR-PS-HC-024:setI", "SR-PS-HC-025:setI", "SR-PS-HC-026:setI", "SR-PS-HC-027:setI", "SR-PS-HC-031:setI", "SR-PS-HC-032:setI", "SR-PS-HC-033:setI", "SR-PS-HC-034:setI", "SR-PS-HC-035:setI", "SR-PS-HC-036:setI", "SR-PS-HC-037:setI", "SR-PS-HC-041:setI", "SR-PS-HC-042:setI", "SR-PS-HC-043:setI", "SR-PS-HC-044:setI", "SR-PS-HC-045:setI", "SR-PS-HC-046:setI", "SR-PS-HC-047:setI", "SR-PS-HC-051:setI", "SR-PS-HC-052:setI", "SR-PS-HC-053:setI", "SR-PS-HC-054:setI", "SR-PS-HC-055:setI", "SR-PS-HC-056:setI", "SR-PS-HC-057:setI", "SR-PS-HC-061:setI", "SR-PS-HC-062:setI", "SR-PS-HC-063:setI", "SR-PS-HC-064:setI", "SR-PS-HC-065:setI", "SR-PS-HC-066:setI", "SR-PS-HC-067:setI", "SR-PS-HC-071:setI", "SR-PS-HC-072:setI", "SR-PS-HC-073:setI", "SR-PS-HC-074:setI", "SR-PS-HC-075:setI", "SR-PS-HC-076:setI", "SR-PS-HC-077:setI", "SR-PS-HC-081:setI", "SR-PS-HC-082:setI", "SR-PS-HC-083:setI", "SR-PS-HC-084:setI", "SR-PS-HC-085:setI", "SR-PS-HC-086:setI", "SR-PS-HC-087:setI", "SR-PS-HC-091:setI", "SR-PS-HC-092:setI", "SR-PS-HC-093:setI", "SR-PS-HC-094:setI", "SR-PS-HC-095:setI", "SR-PS-HC-096:setI", "SR-PS-HC-097:setI", "SR-PS-HC-101:setI", "SR-PS-HC-102:setI", "SR-PS-HC-103:setI", "SR-PS-HC-104:setI", "SR-PS-HC-105:setI", "SR-PS-HC-106:setI", "SR-PS-HC-107:setI", "SR-PS-HC-111:setI", "SR-PS-HC-112:setI", "SR-PS-HC-113:setI", "SR-PS-HC-114:setI", "SR-PS-HC-115:setI", "SR-PS-HC-116:setI", "SR-PS-HC-117:setI", "SR-PS-HC-121:setI", "SR-PS-HC-122:setI", "SR-PS-HC-123:setI", "SR-PS-HC-124:setI", "SR-PS-HC-125:setI", "SR-PS-HC-126:setI", "SR-PS-HC-127:setI", "SR-PS-HC-131:setI", "SR-PS-HC-132:setI", "SR-PS-HC-133:setI", "SR-PS-HC-134:setI", "SR-PS-HC-135:setI", "SR-PS-HC-136:setI", "SR-PS-HC-137:setI", "SR-PS-HC-141:setI", "SR-PS-HC-142:setI", "SR-PS-HC-143:setI", "SR-PS-HC-144:setI", "SR-PS-HC-145:setI", "SR-PS-HC-146:setI", "SR-PS-HC-147:setI", "SR-PS-HC-151:setI", "SR-PS-HC-152:setI", "SR-PS-HC-153:setI", "SR-PS-HC-154:setI", "SR-PS-HC-155:setI", "SR-PS-HC-156:setI", "SR-PS-HC-157:setI", "SR-PS-HC-161:setI", "SR-PS-HC-162:setI", "SR-PS-HC-163:setI", "SR-PS-HC-164:setI", "SR-PS-HC-165:setI", "SR-PS-HC-166:setI", "SR-PS-HC-167:setI", "SR-PS-HC-171:setI", "SR-PS-HC-172:setI", "SR-PS-HC-173:setI", "SR-PS-HC-174:setI", "SR-PS-HC-175:setI", "SR-PS-HC-176:setI", "SR-PS-HC-177:setI", "SR-PS-HC-181:setI", "SR-PS-HC-182:setI", "SR-PS-HC-183:setI", "SR-PS-HC-184:setI", "SR-PS-HC-185:setI", "SR-PS-HC-186:setI", "SR-PS-HC-187:setI", "SR-PS-HC-191:setI", "SR-PS-HC-192:setI", "SR-PS-HC-193:setI", "SR-PS-HC-194:setI", "SR-PS-HC-195:setI", "SR-PS-HC-196:setI", "SR-PS-HC-197:setI", "SR-PS-HC-201:setI", "SR-PS-HC-202:setI", "SR-PS-HC-203:setI", "SR-PS-HC-204:setI", "SR-PS-HC-205:setI", "SR-PS-HC-206:setI", "SR-PS-HC-207:setI", "SR-PS-HC-211:setI", "SR-PS-HC-212:setI", "SR-PS-HC-213:setI", "SR-PS-HC-214:setI", "SR-PS-HC-215:setI", "SR-PS-HC-216:setI", "SR-PS-HC-217:setI", "SR-PS-HC-221:setI", "SR-PS-HC-222:setI", "SR-PS-HC-223:setI", "SR-PS-HC-224:setI", "SR-PS-HC-225:setI", "SR-PS-HC-226:setI", "SR-PS-HC-227:setI", "SR-PS-HC-231:setI", "SR-PS-HC-232:setI", "SR-PS-HC-233:setI", "SR-PS-HC-234:setI", "SR-PS-HC-235:setI", "SR-PS-HC-236:setI", "SR-PS-HC-237:setI", "SR-PS-HC-241:setI", "SR-PS-HC-242:setI", "SR-PS-HC-243:setI", "SR-PS-HC-244:setI", "SR-PS-HC-245:setI", "SR-PS-HC-246:setI", "SR-PS-HC-247:setI", "SR-PS-VC-011:setI", "SR-PS-VC-012:setI", "SR-PS-VC-013:setI", "SR-PS-VC-014:setI", "SR-PS-VC-015:setI", "SR-PS-VC-016:setI", "SR-PS-VC-017:setI", "SR-PS-VC-021:setI", "SR-PS-VC-022:setI", "SR-PS-VC-023:setI", "SR-PS-VC-024:setI", "SR-PS-VC-025:setI", "SR-PS-VC-026:setI", "SR-PS-VC-027:setI", "SR-PS-VC-031:setI", "SR-PS-VC-032:setI", "SR-PS-VC-033:setI", "SR-PS-VC-034:setI", "SR-PS-VC-035:setI", "SR-PS-VC-036:setI", "SR-PS-VC-037:setI", "SR-PS-VC-041:setI", "SR-PS-VC-042:setI", "SR-PS-VC-043:setI", "SR-PS-VC-044:setI", "SR-PS-VC-045:setI", "SR-PS-VC-046:setI", "SR-PS-VC-047:setI", "SR-PS-VC-051:setI", "SR-PS-VC-052:setI", "SR-PS-VC-053:setI", "SR-PS-VC-054:setI", "SR-PS-VC-055:setI", "SR-PS-VC-056:setI", "SR-PS-VC-057:setI", "SR-PS-VC-061:setI", "SR-PS-VC-062:setI", "SR-PS-VC-063:setI", "SR-PS-VC-064:setI", "SR-PS-VC-065:setI", "SR-PS-VC-066:setI", "SR-PS-VC-067:setI", "SR-PS-VC-071:setI", "SR-PS-VC-072:setI", "SR-PS-VC-073:setI", "SR-PS-VC-074:setI", "SR-PS-VC-075:setI", "SR-PS-VC-076:setI", "SR-PS-VC-077:setI", "SR-PS-VC-081:setI", "SR-PS-VC-082:setI", "SR-PS-VC-083:setI", "SR-PS-VC-084:setI", "SR-PS-VC-085:setI", "SR-PS-VC-086:setI", "SR-PS-VC-087:setI", "SR-PS-VC-091:setI", "SR-PS-VC-092:setI", "SR-PS-VC-093:setI", "SR-PS-VC-094:setI", "SR-PS-VC-095:setI", "SR-PS-VC-096:setI", "SR-PS-VC-097:setI", "SR-PS-VC-101:setI", "SR-PS-VC-102:setI", "SR-PS-VC-103:setI", "SR-PS-VC-104:setI", "SR-PS-VC-105:setI", "SR-PS-VC-106:setI", "SR-PS-VC-107:setI", "SR-PS-VC-111:setI", "SR-PS-VC-112:setI", "SR-PS-VC-113:setI", "SR-PS-VC-114:setI", "SR-PS-VC-115:setI", "SR-PS-VC-116:setI", "SR-PS-VC-117:setI", "SR-PS-VC-121:setI", "SR-PS-VC-122:setI", "SR-PS-VC-123:setI", "SR-PS-VC-124:setI", "SR-PS-VC-125:setI", "SR-PS-VC-126:setI", "SR-PS-VC-127:setI", "SR-PS-VC-131:setI", "SR-PS-VC-132:setI", "SR-PS-VC-133:setI", "SR-PS-VC-134:setI", "SR-PS-VC-135:setI", "SR-PS-VC-136:setI", "SR-PS-VC-137:setI", "SR-PS-VC-141:setI", "SR-PS-VC-142:setI", "SR-PS-VC-143:setI", "SR-PS-VC-144:setI", "SR-PS-VC-145:setI", "SR-PS-VC-146:setI", "SR-PS-VC-147:setI", "SR-PS-VC-151:setI", "SR-PS-VC-152:setI", "SR-PS-VC-153:setI", "SR-PS-VC-154:setI", "SR-PS-VC-155:setI", "SR-PS-VC-156:setI", "SR-PS-VC-157:setI", "SR-PS-VC-161:setI", "SR-PS-VC-162:setI", "SR-PS-VC-163:setI", "SR-PS-VC-164:setI", "SR-PS-VC-165:setI", "SR-PS-VC-166:setI", "SR-PS-VC-167:setI", "SR-PS-VC-171:setI", "SR-PS-VC-172:setI", "SR-PS-VC-173:setI", "SR-PS-VC-174:setI", "SR-PS-VC-175:setI", "SR-PS-VC-176:setI", "SR-PS-VC-177:setI", "SR-PS-VC-181:setI", "SR-PS-VC-182:setI", "SR-PS-VC-183:setI", "SR-PS-VC-184:setI", "SR-PS-VC-185:setI", "SR-PS-VC-186:setI", "SR-PS-VC-187:setI", "SR-PS-VC-191:setI", "SR-PS-VC-192:setI", "SR-PS-VC-193:setI", "SR-PS-VC-194:setI", "SR-PS-VC-195:setI", "SR-PS-VC-196:setI", "SR-PS-VC-197:setI", "SR-PS-VC-201:setI", "SR-PS-VC-202:setI", "SR-PS-VC-203:setI", "SR-PS-VC-204:setI", "SR-PS-VC-205:setI", "SR-PS-VC-206:setI", "SR-PS-VC-207:setI", "SR-PS-VC-211:setI", "SR-PS-VC-212:setI", "SR-PS-VC-213:setI", "SR-PS-VC-214:setI", "SR-PS-VC-215:setI", "SR-PS-VC-216:setI", "SR-PS-VC-217:setI", "SR-PS-VC-221:setI", "SR-PS-VC-222:setI", "SR-PS-VC-223:setI", "SR-PS-VC-224:setI", "SR-PS-VC-225:setI", "SR-PS-VC-226:setI", "SR-PS-VC-227:setI", "SR-PS-VC-231:setI", "SR-PS-VC-232:setI", "SR-PS-VC-233:setI", "SR-PS-VC-234:setI", "SR-PS-VC-235:setI", "SR-PS-VC-236:setI", "SR-PS-VC-237:setI", "SR-PS-VC-241:setI", "SR-PS-VC-242:setI", "SR-PS-VC-243:setI", "SR-PS-VC-244:setI", "SR-PS-VC-245:setI", "SR-PS-VC-246:setI", "SR-PS-VC-247:setI", "SR-PS-QL1-0101:setI", "SR-PS-QL2-0102:setI", "SR-PS-QL3-0103:setI", "SR-PS-QS4-0104:setI", "SR-PS-QS5-0105:setI", "SR-PS-QS5-0106:setI", "SR-PS-QS4-0107:setI", "SR-PS-QS3-0108:setI", "SR-PS-QS2-0109:setI", "SR-PS-QS1-0110:setI", "SR-PS-QS1-0201:setI", "SR-PS-QS2-0202:setI", "SR-PS-QS3-0203:setI", "SR-PS-QS4-0204:setI", "SR-PS-QS5-0205:setI", "SR-PS-QS5-0206:setI", "SR-PS-QS4-0207:setI", "SR-PS-QS3-0208:setI", "SR-PS-QS2-0209:setI", "SR-PS-QS1-0210:setI", "SR-PS-QS1-0301:setI", "SR-PS-QS2-0302:setI", "SR-PS-QS3-0303:setI", "SR-PS-QS4-0304:setI", "SR-PS-QS5-0305:setI", "SR-PS-QS5-0306:setI", "SR-PS-QS4-0307:setI", "SR-PS-QS3-0308:setI", "SR-PS-QS2-0309:setI", "SR-PS-QS1-0310:setI", "SR-PS-QS1-0401:setI", "SR-PS-QS2-0402:setI", "SR-PS-QS3-0403:setI", "SR-PS-QS4-0404:setI", "SR-PS-QS5-0405:setI", "SR-PS-QS5-0406:setI", "SR-PS-QS4-0407:setI", "SR-PS-QL3-0408:setI", "SR-PS-QL2-0409:setI", "SR-PS-QL1-0410:setI", "SR-PS-QL1-0501:setI", "SR-PS-QL2-0502:setI", "SR-PS-QL3-0503:setI", "SR-PS-QS4-0504:setI", "SR-PS-QS5-0505:setI", "SR-PS-QS5-0506:setI", "SR-PS-QS4-0507:setI", "SR-PS-QS3-0508:setI", "SR-PS-QS2-0509:setI", "SR-PS-QS1-0510:setI", "SR-PS-QS1-0601:setI", "SR-PS-QS2-0602:setI", "SR-PS-QS3-0603:setI", "SR-PS-QS4-0604:setI", "SR-PS-QS5-0605:setI", "SR-PS-QS5-0606:setI", "SR-PS-QS4-0607:setI", "SR-PS-QS3-0608:setI", "SR-PS-QS2-0609:setI", "SR-PS-QS1-0610:setI", "SR-PS-QS1-0701:setI", "SR-PS-QS2-0702:setI", "SR-PS-QS3-0703:setI", "SR-PS-QS4-0704:setI", "SR-PS-QS5-0705:setI", "SR-PS-QS5-0706:setI", "SR-PS-QS4-0707:setI", "SR-PS-QS3-0708:setI", "SR-PS-QS2-0709:setI", "SR-PS-QS1-0710:setI", "SR-PS-QS1-0801:setI", "SR-PS-QS2-0802:setI", "SR-PS-QS3-0803:setI", "SR-PS-QS4-0804:setI", "SR-PS-QS5-0805:setI", "SR-PS-QS5-0806:setI", "SR-PS-QS4-0807:setI", "SR-PS-QL3-0808:setI", "SR-PS-QL2-0809:setI", "SR-PS-QL1-0810:setI", "SR-PS-QL1-0901:setI", "SR-PS-QL2-0902:setI", "SR-PS-QL3-0903:setI", "SR-PS-QS4-0904:setI", "SR-PS-QS5-0905:setI", "SR-PS-QS5-0906:setI", "SR-PS-QS4-0907:setI", "SR-PS-QS3-0908:setI", "SR-PS-QS2-0909:setI", "SR-PS-QS1-0910:setI", "SR-PS-QS1-1001:setI", "SR-PS-QS2-1002:setI", "SR-PS-QS3-1003:setI", "SR-PS-QS4-1004:setI", "SR-PS-QS5-1005:setI", "SR-PS-QS5-1006:setI", "SR-PS-QS4-1007:setI", "SR-PS-QS3-1008:setI", "SR-PS-QS2-1009:setI", "SR-PS-QS1-1010:setI", "SR-PS-QS1-1101:setI", "SR-PS-QS2-1102:setI", "SR-PS-QS3-1103:setI", "SR-PS-QS4-1104:setI", "SR-PS-QS5-1105:setI", "SR-PS-QS5-1106:setI", "SR-PS-QS4-1107:setI", "SR-PS-QS3-1108:setI", "SR-PS-QS2-1109:setI", "SR-PS-QS1-1110:setI", "SR-PS-QS1-1201:setI", "SR-PS-QS2-1202:setI", "SR-PS-QS3-1203:setI", "SR-PS-QS4-1204:setI", "SR-PS-QS5-1205:setI", "SR-PS-QS5-1206:setI", "SR-PS-QS4-1207:setI", "SR-PS-QL3-1208:setI", "SR-PS-QL2-1209:setI", "SR-PS-QL1-1210:setI", "SR-PS-QL1-1301:setI", "SR-PS-QL2-1302:setI", "SR-PS-QL3-1303:setI", "SR-PS-QS4-1304:setI", "SR-PS-QS5-1305:setI", "SR-PS-QS5-1306:setI", "SR-PS-QS4-1307:setI", "SR-PS-QS3-1308:setI", "SR-PS-QS2-1309:setI", "SR-PS-QS1-1310:setI", "SR-PS-QS1-1401:setI", "SR-PS-QS2-1402:setI", "SR-PS-QS3-1403:setI", "SR-PS-QS4-1404:setI", "SR-PS-QS5-1405:setI", "SR-PS-QS5-1406:setI", "SR-PS-QS4-1407:setI", "SR-PS-QS3-1408:setI", "SR-PS-QS2-1409:setI", "SR-PS-QS1-1410:setI", "SR-PS-QS1-1501:setI", "SR-PS-QS2-1502:setI", "SR-PS-QS3-1503:setI", "SR-PS-QS4-1504:setI", "SR-PS-QS5-1505:setI", "SR-PS-QS5-1506:setI", "SR-PS-QS4-1507:setI", "SR-PS-QS3-1508:setI", "SR-PS-QS2-1509:setI", "SR-PS-QS1-1510:setI", "SR-PS-QS1-1601:setI", "SR-PS-QS2-1602:setI", "SR-PS-QS3-1603:setI", "SR-PS-QS4-1604:setI", "SR-PS-QS5-1605:setI", "SR-PS-QS5-1606:setI", "SR-PS-QS4-1607:setI", "SR-PS-QL3-1608:setI", "SR-PS-QL2-1609:setI", "SR-PS-QL1-1610:setI", "SR-PS-QL1-1701:setI", "SR-PS-QL2-1702:setI", "SR-PS-QL3-1703:setI", "SR-PS-QS4-1704:setI", "SR-PS-QS5-1705:setI", "SR-PS-QS5-1706:setI", "SR-PS-QS4-1707:setI", "SR-PS-QS3-1708:setI", "SR-PS-QS2-1709:setI", "SR-PS-QS1-1710:setI", "SR-PS-QS1-1801:setI", "SR-PS-QS2-1802:setI", "SR-PS-QS3-1803:setI", "SR-PS-QS4-1804:setI", "SR-PS-QS5-1805:setI", "SR-PS-QS5-1806:setI", "SR-PS-QS4-1807:setI", "SR-PS-QS3-1808:setI", "SR-PS-QS2-1809:setI", "SR-PS-QS1-1810:setI", "SR-PS-QS1-1901:setI", "SR-PS-QS2-1902:setI", "SR-PS-QS3-1903:setI", "SR-PS-QS4-1904:setI", "SR-PS-QS5-1905:setI", "SR-PS-QS5-1906:setI", "SR-PS-QS4-1907:setI", "SR-PS-QS3-1908:setI", "SR-PS-QS2-1909:setI", "SR-PS-QS1-1910:setI", "SR-PS-QS1-2001:setI", "SR-PS-QS2-2002:setI", "SR-PS-QS3-2003:setI", "SR-PS-QS4-2004:setI", "SR-PS-QS5-2005:setI", "SR-PS-QS5-2006:setI", "SR-PS-QS4-2007:setI", "SR-PS-QL3-2008:setI", "SR-PS-QL2-2009:setI", "SR-PS-QL1-2010:setI", "SR-PS-QL1-2101:setI", "SR-PS-QL2-2102:setI", "SR-PS-QL3-2103:setI", "SR-PS-QS4-2104:setI", "SR-PS-QS5-2105:setI", "SR-PS-QS5-2106:setI", "SR-PS-QS4-2107:setI", "SR-PS-QS3-2108:setI", "SR-PS-QS2-2109:setI", "SR-PS-QS1-2110:setI", "SR-PS-QS1-2201:setI", "SR-PS-QS2-2202:setI", "SR-PS-QS3-2203:setI", "SR-PS-QS4-2204:setI", "SR-PS-QS5-2205:setI", "SR-PS-QS5-2206:setI", "SR-PS-QS4-2207:setI", "SR-PS-QS3-2208:setI", "SR-PS-QS2-2209:setI", "SR-PS-QS1-2210:setI", "SR-PS-QS1-2301:setI", "SR-PS-QS2-2302:setI", "SR-PS-QS3-2303:setI", "SR-PS-QS4-2304:setI", "SR-PS-QS5-2305:setI", "SR-PS-QS5-2306:setI", "SR-PS-QS4-2307:setI", "SR-PS-QS3-2308:setI", "SR-PS-QS2-2309:setI", "SR-PS-QS1-2310:setI", "SR-PS-QS1-2401:setI", "SR-PS-QS2-2402:setI", "SR-PS-QS3-2403:setI", "SR-PS-QS4-2404:setI", "SR-PS-QS5-2405:setI", "SR-PS-QS5-2406:setI", "SR-PS-QS4-2407:setI", "SR-PS-QL3-2408:setI", "SR-PS-QL2-2409:setI", "SR-PS-QL1-2410:setI", "SR-PS-S1-011:setI", "SR-PS-S2-012:setI", "SR-PS-SD-013:setI", "SR-PS-SF-014:setI", "SR-PS-SD-015:setI", "SR-PS-S4-016:setI", "SR-PS-S3-017:setI", "SR-PS-S5-021:setI", "SR-PS-S6-022:setI", "SR-PS-SD-023:setI", "SR-PS-SF-024:setI", "SR-PS-SD-025:setI", "SR-PS-S6-026:setI", "SR-PS-S5-027:setI", "SR-PS-S5-031:setI", "SR-PS-S6-032:setI", "SR-PS-SD-033:setI", "SR-PS-SF-034:setI", "SR-PS-SD-035:setI", "SR-PS-S6-036:setI", "SR-PS-S5-037:setI", "SR-PS-S3-041:setI", "SR-PS-S4-042:setI", "SR-PS-SD-043:setI", "SR-PS-SF-044:setI", "SR-PS-SD-045:setI", "SR-PS-S2-046:setI", "SR-PS-S1-047:setI", "SR-PS-S1-051:setI", "SR-PS-S2-052:setI", "SR-PS-SD-053:setI", "SR-PS-SF-054:setI", "SR-PS-SD-055:setI", "SR-PS-S4-056:setI", "SR-PS-S3-057:setI", "SR-PS-S5-061:setI", "SR-PS-S6-062:setI", "SR-PS-SD-063:setI", "SR-PS-SF-064:setI", "SR-PS-SD-065:setI", "SR-PS-S6-066:setI", "SR-PS-S5-067:setI", "SR-PS-S5-071:setI", "SR-PS-S6-072:setI", "SR-PS-SD-073:setI", "SR-PS-SF-074:setI", "SR-PS-SD-075:setI", "SR-PS-S6-076:setI", "SR-PS-S5-077:setI", "SR-PS-S3-081:setI", "SR-PS-S4-082:setI", "SR-PS-SD-083:setI", "SR-PS-SF-084:setI", "SR-PS-SD-085:setI", "SR-PS-S2-086:setI", "SR-PS-S1-087:setI", "SR-PS-S1-091:setI", "SR-PS-S2-092:setI", "SR-PS-SD-093:setI", "SR-PS-SF-094:setI", "SR-PS-SD-095:setI", "SR-PS-S4-096:setI", "SR-PS-S3-097:setI", "SR-PS-S5-101:setI", "SR-PS-S6-102:setI", "SR-PS-SD-103:setI", "SR-PS-SF-104:setI", "SR-PS-SD-105:setI", "SR-PS-S6-106:setI", "SR-PS-S5-107:setI", "SR-PS-S5-111:setI", "SR-PS-S6-112:setI", "SR-PS-SD-113:setI", "SR-PS-SF-114:setI", "SR-PS-SD-115:setI", "SR-PS-S6-116:setI", "SR-PS-S5-117:setI", "SR-PS-S3-121:setI", "SR-PS-S4-122:setI", "SR-PS-SD-123:setI", "SR-PS-SF-124:setI", "SR-PS-SD-125:setI", "SR-PS-S2-126:setI", "SR-PS-S1-127:setI", "SR-PS-S1-131:setI", "SR-PS-S2-132:setI", "SR-PS-SD-133:setI", "SR-PS-SF-134:setI", "SR-PS-SD-135:setI", "SR-PS-S4-136:setI", "SR-PS-S3-137:setI", "SR-PS-S5-141:setI", "SR-PS-S6-142:setI", "SR-PS-SD-143:setI", "SR-PS-SF-144:setI", "SR-PS-SD-145:setI", "SR-PS-S6-146:setI", "SR-PS-S5-147:setI", "SR-PS-S5-151:setI", "SR-PS-S6-152:setI", "SR-PS-SD-153:setI", "SR-PS-SF-154:setI", "SR-PS-SD-155:setI", "SR-PS-S6-156:setI", "SR-PS-S5-157:setI", "SR-PS-S3-161:setI", "SR-PS-S4-162:setI", "SR-PS-SD-163:setI", "SR-PS-SF-164:setI", "SR-PS-SD-165:setI", "SR-PS-S2-166:setI", "SR-PS-S1-167:setI", "SR-PS-S1-171:setI", "SR-PS-S2-172:setI", "SR-PS-SD-173:setI", "SR-PS-SF-174:setI", "SR-PS-SD-175:setI", "SR-PS-S4-176:setI", "SR-PS-S3-177:setI", "SR-PS-S5-181:setI", "SR-PS-S6-182:setI", "SR-PS-SD-183:setI", "SR-PS-SF-184:setI", "SR-PS-SD-185:setI", "SR-PS-S6-186:setI", "SR-PS-S5-187:setI", "SR-PS-S5-191:setI", "SR-PS-S6-192:setI", "SR-PS-SD-193:setI", "SR-PS-SF-194:setI", "SR-PS-SD-195:setI", "SR-PS-S6-196:setI", "SR-PS-S5-197:setI", "SR-PS-S3-201:setI", "SR-PS-S4-202:setI", "SR-PS-SD-203:setI", "SR-PS-SF-204:setI", "SR-PS-SD-205:setI", "SR-PS-S2-206:setI", "SR-PS-S1-207:setI", "SR-PS-S1-211:setI", "SR-PS-S2-212:setI", "SR-PS-SD-213:setI", "SR-PS-SF-214:setI", "SR-PS-SD-215:setI", "SR-PS-S4-216:setI", "SR-PS-S3-217:setI", "SR-PS-S5-221:setI", "SR-PS-S6-222:setI", "SR-PS-SD-223:setI", "SR-PS-SF-224:setI", "SR-PS-SD-225:setI", "SR-PS-S6-226:setI", "SR-PS-S5-227:setI", "SR-PS-S5-231:setI", "SR-PS-S6-232:setI", "SR-PS-SD-233:setI", "SR-PS-SF-234:setI", "SR-PS-SD-235:setI", "SR-PS-S6-236:setI", "SR-PS-S5-237:setI", "SR-PS-S3-241:setI", "SR-PS-S4-242:setI", "SR-PS-SD-243:setI", "SR-PS-SF-244:setI", "SR-PS-SD-245:setI", "SR-PS-S2-246:setI", "SR-PS-S1-247:setI", "SR-PS-SKEW-011:setI", "SR-PS-SKEW-012:setI", "SR-PS-SKEW-013:setI", "SR-PS-SKEW-014:setI", "SR-PS-SKEW-015:setI", "SR-PS-SKEW-016:setI", "SR-PS-SKEW-017:setI", "SR-PS-SKEW-021:setI", "SR-PS-SKEW-022:setI", "SR-PS-SKEW-023:setI", "SR-PS-SKEW-024:setI", "SR-PS-SKEW-025:setI", "SR-PS-SKEW-026:setI", "SR-PS-SKEW-027:setI", "SR-PS-SKEW-031:setI", "SR-PS-SKEW-032:setI", "SR-PS-SKEW-033:setI", "SR-PS-SKEW-034:setI", "SR-PS-SKEW-035:setI", "SR-PS-SKEW-036:setI", "SR-PS-SKEW-037:setI", "SR-PS-SKEW-041:setI", "SR-PS-SKEW-042:setI", "SR-PS-SKEW-043:setI", "SR-PS-SKEW-044:setI", "SR-PS-SKEW-045:setI", "SR-PS-SKEW-046:setI", "SR-PS-SKEW-047:setI", "SR-PS-SKEW-051:setI", "SR-PS-SKEW-052:setI", "SR-PS-SKEW-053:setI", "SR-PS-SKEW-054:setI", "SR-PS-SKEW-055:setI", "SR-PS-SKEW-056:setI", "SR-PS-SKEW-057:setI", "SR-PS-SKEW-061:setI", "SR-PS-SKEW-062:setI", "SR-PS-SKEW-063:setI", "SR-PS-SKEW-064:setI", "SR-PS-SKEW-065:setI", "SR-PS-SKEW-066:setI", "SR-PS-SKEW-067:setI", "SR-PS-SKEW-071:setI", "SR-PS-SKEW-072:setI", "SR-PS-SKEW-073:setI", "SR-PS-SKEW-074:setI", "SR-PS-SKEW-075:setI", "SR-PS-SKEW-076:setI", "SR-PS-SKEW-077:setI", "SR-PS-SKEW-081:setI", "SR-PS-SKEW-082:setI", "SR-PS-SKEW-083:setI", "SR-PS-SKEW-084:setI", "SR-PS-SKEW-085:setI", "SR-PS-SKEW-086:setI", "SR-PS-SKEW-087:setI", "SR-PS-SKEW-091:setI", "SR-PS-SKEW-092:setI", "SR-PS-SKEW-093:setI", "SR-PS-SKEW-094:setI", "SR-PS-SKEW-095:setI", "SR-PS-SKEW-096:setI", "SR-PS-SKEW-097:setI", "SR-PS-SKEW-101:setI", "SR-PS-SKEW-102:setI", "SR-PS-SKEW-103:setI", "SR-PS-SKEW-104:setI", "SR-PS-SKEW-105:setI", "SR-PS-SKEW-106:setI", "SR-PS-SKEW-107:setI", "SR-PS-SKEW-111:setI", "SR-PS-SKEW-112:setI", "SR-PS-SKEW-113:setI", "SR-PS-SKEW-114:setI", "SR-PS-SKEW-115:setI", "SR-PS-SKEW-116:setI", "SR-PS-SKEW-117:setI", "SR-PS-SKEW-121:setI", "SR-PS-SKEW-122:setI", "SR-PS-SKEW-123:setI", "SR-PS-SKEW-124:setI", "SR-PS-SKEW-125:setI", "SR-PS-SKEW-126:setI", "SR-PS-SKEW-127:setI", "SR-PS-SKEW-131:setI", "SR-PS-SKEW-132:setI", "SR-PS-SKEW-133:setI", "SR-PS-SKEW-134:setI", "SR-PS-SKEW-135:setI", "SR-PS-SKEW-136:setI", "SR-PS-SKEW-137:setI", "SR-PS-SKEW-141:setI", "SR-PS-SKEW-142:setI", "SR-PS-SKEW-143:setI", "SR-PS-SKEW-144:setI", "SR-PS-SKEW-145:setI", "SR-PS-SKEW-146:setI", "SR-PS-SKEW-147:setI", "SR-PS-SKEW-151:setI", "SR-PS-SKEW-152:setI", "SR-PS-SKEW-153:setI", "SR-PS-SKEW-154:setI", "SR-PS-SKEW-155:setI", "SR-PS-SKEW-156:setI", "SR-PS-SKEW-157:setI", "SR-PS-SKEW-161:setI", "SR-PS-SKEW-162:setI", "SR-PS-SKEW-163:setI", "SR-PS-SKEW-164:setI", "SR-PS-SKEW-165:setI", "SR-PS-SKEW-166:setI", "SR-PS-SKEW-167:setI", "SR-PS-SKEW-171:setI", "SR-PS-SKEW-172:setI", "SR-PS-SKEW-173:setI", "SR-PS-SKEW-174:setI", "SR-PS-SKEW-175:setI", "SR-PS-SKEW-176:setI", "SR-PS-SKEW-177:setI", "SR-PS-SKEW-181:setI", "SR-PS-SKEW-182:setI", "SR-PS-SKEW-183:setI", "SR-PS-SKEW-184:setI", "SR-PS-SKEW-185:setI", "SR-PS-SKEW-186:setI", "SR-PS-SKEW-187:setI", "SR-PS-SKEW-191:setI", "SR-PS-SKEW-192:setI", "SR-PS-SKEW-193:setI", "SR-PS-SKEW-194:setI", "SR-PS-SKEW-195:setI", "SR-PS-SKEW-196:setI", "SR-PS-SKEW-197:setI", "SR-PS-SKEW-201:setI", "SR-PS-SKEW-202:setI", "SR-PS-SKEW-203:setI", "SR-PS-SKEW-204:setI", "SR-PS-SKEW-205:setI", "SR-PS-SKEW-206:setI", "SR-PS-SKEW-207:setI", "SR-PS-SKEW-211:setI", "SR-PS-SKEW-212:setI", "SR-PS-SKEW-213:setI", "SR-PS-SKEW-214:setI", "SR-PS-SKEW-215:setI", "SR-PS-SKEW-216:setI", "SR-PS-SKEW-217:setI", "SR-PS-SKEW-221:setI", "SR-PS-SKEW-222:setI", "SR-PS-SKEW-223:setI", "SR-PS-SKEW-224:setI", "SR-PS-SKEW-225:setI", "SR-PS-SKEW-226:setI", "SR-PS-SKEW-227:setI", "SR-PS-SKEW-231:setI", "SR-PS-SKEW-232:setI", "SR-PS-SKEW-233:setI", "SR-PS-SKEW-234:setI", "SR-PS-SKEW-235:setI", "SR-PS-SKEW-236:setI", "SR-PS-SKEW-237:setI", "SR-PS-SKEW-241:setI", "SR-PS-SKEW-242:setI", "SR-PS-SKEW-243:setI", "SR-PS-SKEW-244:setI", "SR-PS-SKEW-245:setI", "SR-PS-SKEW-246:setI", "SR-PS-SKEW-247:setI", "SR-RF2-LLRF:setGapVoltage", "SR-RF2-LLRF:setStationPhase", "SR-RF3-LLRF:setGapVoltage", "SR-RF3-LLRF:setStationPhase", "SR-PS-DMB09-Q1:setI", "SR-PS-DMB09-Q2:setI", "SR-PS-DMB09-Q3:setI", "SR-PS-DMB25-Q1:setI", "SR-PS-DMB25-Q2:setI", "SR-PS-DMB25-Q3:setI", "SR-PS-DMB41-Q1:setI", "SR-PS-DMB41-Q2:setI", "SR-PS-DMB41-Q3:setI", "SR-PS-DMB09-HC1:setI", "SR-PS-DMB09-HC2:setI", "SR-PS-DMB09-VC1:setI", "SR-PS-DMB09-VC2:setI", "SR-PS-DMB25-HC1:setI", "SR-PS-DMB25-HC2:setI", "SR-PS-DMB25-VC1:setI", "SR-PS-DMB25-VC2:setI", "SR-PS-DMB41-HC1:setI", "SR-PS-DMB41-HC2:setI", "SR-PS-DMB41-VC1:setI", "SR-PS-DMB41-VC2:setI"]  # PV nanes(SR)
  w10 = string[] ["LTB-PS-HC-1:setI", "LTB-PS-HC-2:setI", "LTB-PS-HC-3:setI", "LTB-PS-HC-4:setI", "LTB-PS-HC-5:setI", "LTB-PS-VC-1:setI", "LTB-PS-VC-2:setI", "LTB-PS-VC-3:setI", "LTB-PS-VC-4:setI", "LTB-PS-VC-5:setI", "LTB-PS-VC-6:setI", "LTB-PS-VC-7:setI", "LTB-PS-Q1A:setI", "LTB-PS-Q1B:setI", "LTB-PS-Q1C:setI", "LTB-PS-Q2A:setI", "LTB-PS-Q2B:setI", "LTB-PS-Q2C:setI", "LTB-PS-Q3A:setI", "LTB-PS-Q3B:setI", "LTB-PS-Q4A:setI", "LTB-PS-Q4B:setI", "LTB-PS-QQ:setI", "LTB-PS-BEND-1:setI", "LTB-PS-VC-2a:setI", "LTB-PS-HC-3a:setI", "LTB-PS-HC-3b:setI", "LTB-PS-HC-4a:setI", "LTB-PS-HC-5a:setI", "LI-DI-SLIT-motor:axis2Position1", "LI-DI-SLIT-motor:axis1Position1"]  # PV nanes(LTB)
  w12 = string[] ["BTS-PS-HC-1:setI", "BTS-PS-HC-2:setI", "BTS-PS-HC-3:setI", "BTS-PS-HC-4:setI", "BTS-PS-HC-5:setI", "BTS-PS-VC-2:setI", "BTS-PS-VC-3:setI", "BTS-PS-VC-4:setI", "BTS-PS-VC-5:setI", "BTS-PS-VC-6:setI", "BTS-PS-Q1A:setI", "BTS-PS-Q1B:setI", "BTS-PS-Q1C:setI", "BTS-PS-Q2A:setI", "BTS-PS-Q2B:setI", "BTS-PS-Q2C:setI", "BTS-PS-Q3A:setI", "BTS-PS-BEND-1:setI", "BTS-PS-BEND-2:setI", "BR-PS-EXT-K1:setHV", "BR-PS-EXT-K2:setHV", "SR-PS-INJ-SE1:setHV", "SR-PS-INJ-SE2:setHV", "SR-PS-INJ-K1:setHV", "SR-PS-INJ-K2:setHV", "SR-PS-INJ-K3:setHV", "SR-PS-INJ-K4:setHV", "CPCIPM-TI-EVR:Pulse4DelaySet", "CPCIPM-TI-EVR:Pulse5DelaySet", "CPCIPM-TI-EVR:Pulse3DelaySet", "CPCIPM-TI-EVR:Pulse6DelaySet", "CPCIPM-TI-EVR:Pulse7DelaySet", "T560:setADelay", "T560:setBDelay", "T560:setCDelay", "T560:setDDelay", "CPCIPM-TI-EVR:Pulse4DelaySet", "CPCIPM-TI-EVR:Pulse5DelaySet", "BR-PS-EXT-SE1:setHV", "BR-PS-EXT-SE2:setHV", "CPCIPM-TI-EVR:Pulse3DelaySet", "CPCIPM-TI-EVR:Pulse11DelaySet"]  # PV nanes(BTS)
  w11 = string[] ["BR-PS-HC-101:setI", "BR-PS-HC-102:setI", "BR-PS-HC-103:setI", "BR-PS-HC-104:setI", "BR-PS-HC-105:setI", "BR-PS-HC-106:setI", "BR-PS-HC-107:setI", "BR-PS-HC-108:setI", "BR-PS-HC-109:setI", "BR-PS-HC-110:setI", "BR-PS-HC-201:setI", "BR-PS-HC-202:setI", "BR-PS-HC-203:setI", "BR-PS-HC-204:setI", "BR-PS-HC-205:setI", "BR-PS-HC-206:setI", "BR-PS-HC-207:setI", "BR-PS-HC-208:setI", "BR-PS-HC-209:setI", "BR-PS-HC-210:setI", "BR-PS-HC-301:setI", "BR-PS-HC-302:setI", "BR-PS-HC-303:setI", "BR-PS-HC-304:setI", "BR-PS-HC-305:setI", "BR-PS-HC-306:setI", "BR-PS-HC-307:setI", "BR-PS-HC-308:setI", "BR-PS-HC-309:setI", "BR-PS-HC-310:setI", "BR-PS-HC-401:setI", "BR-PS-HC-402:setI", "BR-PS-HC-403:setI", "BR-PS-HC-404:setI", "BR-PS-HC-405:setI", "BR-PS-HC-406:setI", "BR-PS-HC-407:setI", "BR-PS-HC-408:setI", "BR-PS-HC-409:setI", "BR-PS-HC-410:setI", "BR-PS-HC-501:setI", "BR-PS-HC-502:setI", "BR-PS-HC-503:setI", "BR-PS-HC-504:setI", "BR-PS-HC-505:setI", "BR-PS-HC-506:setI", "BR-PS-HC-507:setI", "BR-PS-HC-508:setI", "BR-PS-HC-509:setI", "BR-PS-HC-510:setI", "BR-PS-HC-601:setI", "BR-PS-HC-602:setI", "BR-PS-HC-603:setI", "BR-PS-HC-603a:setI", "BR-PS-HC-604:setI", "BR-PS-HC-605:setI", "BR-PS-HC-606:setI", "BR-PS-HC-606a:setI", "BR-PS-HC-607:setI", "BR-PS-HC-608:setI", "BR-PS-HC-609:setI", "BR-PS-HC-610:setI", "BR-PS-VC-101:setI", "BR-PS-VC-102:setI", "BR-PS-VC-103:setI", "BR-PS-VC-104:setI", "BR-PS-VC-105:setI", "BR-PS-VC-106:setI", "BR-PS-VC-201:setI", "BR-PS-VC-202:setI", "BR-PS-VC-203:setI", "BR-PS-VC-204:setI", "BR-PS-VC-205:setI", "BR-PS-VC-206:setI", "BR-PS-VC-301:setI", "BR-PS-VC-302:setI", "BR-PS-VC-303:setI", "BR-PS-VC-304:setI", "BR-PS-VC-305:setI", "BR-PS-VC-306:setI", "BR-PS-VC-401:setI", "BR-PS-VC-402:setI", "BR-PS-VC-403:setI", "BR-PS-VC-404:setI", "BR-PS-VC-405:setI", "BR-PS-VC-406:setI", "BR-PS-VC-501:setI", "BR-PS-VC-502:setI", "BR-PS-VC-503:setI", "BR-PS-VC-504:setI", "BR-PS-VC-505:setI", "BR-PS-VC-506:setI", "BR-PS-VC-601:setI", "BR-PS-VC-602:setI", "BR-PS-VC-602a:setI", "BR-PS-VC-603:setI", "BR-PS-VC-604:setI", "BR-PS-VC-604a:setI", "BR-PS-VC-605:setI", "BR-PS-VC-606:setI", "BR-PS-VC-100a:setI", "BR-PS-SD:setI", "BR-PS-SF:setI", "cpsc_027:AO:SLOW_SET:CH:1", "cpsc_037:AO:SLOW_SET:CH:3", "BR-RF-LLRF:setStationPhase", "TI-INJ-PROC:setTinj", "BR-PS-INJ-SE:setHV", "CPCIPM-TI-EVR:Pulse1DelaySet", "BR-PS-INJ-KI:setHV", "CPCIPM-TI-EVR:Pulse2DelaySet", "BR-PS-QF:setWfDC", "BR-PS-QM:setWfDC", "BR-PS-Q1:setWfDC", "BR-PS-Q2:setWfDC", "BR-PS-BEND:setWfDC"]  # PV nanes (BR_without_Wf)
  w16 = FALSE ("Trip Evt B")
  (unwired) string[] ["FE-DI-XBPM-051:SA:SA_X_MONITOR", "FE-DI-XBPM-051:SA:SA_Y_MONITOR", "FE-DI-XBPM-091:SA:SA_X_MONITOR", "FE-DI-XBPM-091:SA:SA_Y_MONITOR", "FE-DI-XBPM-211:SA:SA_X_MONITOR", "FE-DI-XBPM-211:SA:SA_Y_MONITOR", "FE-DI-XBPM-231:SA:SA_X_MONITOR", "FE-DI-XBPM-231:SA:SA_Y_MONITOR", "FE-DI-XBPM-251:SA:SA_X_MONITOR", "FE-DI-XBPM-251:SA:SA_Y_MONITOR", "FE-DI-XBPM-411:SA:SA_X_MONITOR", "FE-DI-XBPM-411:SA:SA_Y_MONITOR", "FE-DI-XBPM-451:SA:SA_X_MONITOR", "FE-DI-XBPM-451:SA:SA_Y_MONITOR"]
  (unwired) string[] ["LI-VA-VAL-01:STA:POS", "LI-VA-VAL-02:STA:POS", "LI-VA-VAL-03:STA:POS", "LI-VA-VAL-04:STA:POS", "LI-VA-VAL-05:STA:POS"]
  (unwired) string[] ["SR-DI-SOFB-H:getStatus", "SR-DI-SOFB-V:getStatus", "IGPF:TPSX:FBCTRL", "IGPF:TPSY:FBCTRL", "SR-DI-FOFB-H:getStatus", "SR-DI-FOFB-V:getStatus"]
  # "這兩個變動太頻繁，不紀錄"
  # "PV nanes(ID gap_phase_Taper_)"
  # "PV nanes(Feedback_ILK)"
  # "V1.4.2 改成直接用最大最小值當作scale的最大最小值"
  # "1.4.1\n將BeamCurrent 圖形的Y軸上下限\n改成取最大值的1.01倍，再無條件進位取整數\n最小值的0.99倍，再無條件捨去取整數"
  # "FE-DI-XBPM-051:SA:SA_Y_MONITOR"
  # "FE-DI-XBPM-051:SA:SA_X_MONITOR"
  # "TPS-SR-052:bpm4:ilk:enabled"
  # "0 為OPEN"
  # "VALVE(EPICS)"
  n1 = local read "last ? Hrs"() -> (w26:dbl)
  n2 = Multiply(x=3600.0 ("y"), y=w26) -> (x*y=w50:dbl)
  n3 = Get Date/Time In Seconds() -> (seconds since 1Jan1904=w21:timestamp)
  n4 = Subtract(x=w21, y=w50) -> (x-y=w20:timestamp)
  n5 = call "TimeToString.vi"("Time Stamp Control"=w21) -> ("result string"=w52:string)
  n6 = call "TimeToString.vi"("Time Stamp Control"=w20) -> ("result string"=w51:string)
  n7 = call <vilib>:"Application Directory.vi"() -> ("Application Directory"=w53:path)
  n8 = Build Path(base path=w53, name or relative path="DSN\\172-18-0-32.dsn") -> (appended path=w55:path)
  n9 = call-poly <vilib>:"DB Tools Open Connection.vi"("connection information"=w55) -> ("error out"=w44:errorcluster, "connection reference"=w43:T2)  [unwired: 7 in]
  n10 = Concatenate Strings("SELECT  float_val , smpl_time\nFROM sample \nwhere  channel_id = 104 and smpl_time between '" ("result string"), w51, "' ::timestamp and '" ("result string"), w52, "' ::timestamp" ("result string")) -> (w28:string)
  n11 = call-poly <vilib>:"DB Tools Execute Query.vi"("error in (no error)"=w44, "SQL query"=w28, "connection reference"=w43) -> ("error out"=w41:errorcluster, "recordset reference"=w42:T3)  [unwired: 5 in]
  n12 = call-poly <vilib>:"DB Tools Fetch Recordset Data.vi"("error in (no error)"=w41, "recordset reference"=w42) -> ("error out"=w39:errorcluster, "recordset data"=w36:variant[][], "recordset reference out"=w40:T3)  [unwired: 3 in]
  n13 = call-poly <vilib>:"DB Tools Free Object.vi"("error in (no error)"=w39, "recordset reference"=w40) -> ("error out"=w37:errorcluster, "connection reference"=w38:T2)  [unwired: 8 in]
  n14 = Variant To Data(type=string[][] [], Variant=w36) -> (data=w34:string[][])  [unwired: 1 in, 1 out]
  n15 = call <vilib>:"DB Tools Close Connection.vi"("error in (no error)"=w37, "connection reference"=w38) -> ()  [unwired: 5 in, 1 out]
  n16 = Transpose 2D Array(2D array=w34) -> (transposed array=w32:string[][])
  n17 = Index Array(array=w32, index (row) #1=0 ("index (row)"), index (row) #2=1 ("index (row)")) -> (element #1=w46:string[], element #2=w48:string[])  [unwired: 2 in]
  n18 = Fract/Exp String To Number(string=w46) -> (number=w22:dbl[])  [unwired: 3 in, 1 out]
  n19 = Array Max & Min(array=w22) -> (max value=w18:dbl, min value=w17:dbl)  [unwired: 2 out]
  n20 = for {
    tunnel: w48 -> [w59] mode=indexing
    tunnel: [w58] -> w47 mode=indexing
    n21 = Scan From String "Scan From String"(format string="%<%Y/%m/%d %p %I:%M:%S>T", input string=w59, initial scan location=u32 0, default 1=timestamp(-73814400 s since 1904-01-01)) -> (output 1=w62:timestamp)  [unwired: 1 in, 3 out]
    n22 = To Double Precision Float(number=w62) -> (double precision float=w58:dbl)
  }
  n23 = To Double Precision Float(number=w21) -> (double precision float=w24:dbl)
  n24 = To Double Precision Float(number=w20) -> (double precision float=w23:dbl)
  n25 = control-ref of="BeamCurrent History"() -> (w25:refnum<vi>)
  n26 = property on="Property Node" class="XYGraph (strict)"(reference=w25, "XScale.Maximum"=w24, "XScale.Minimum"=w23, "YScale.Maximum"=w18, "YScale.Minimum"=w17) -> ()  [unwired: 1 in, 2 out]
  n27 = local write "Refresh B"(w16) -> ()
  n28 = local write "Trip Evt B"(w16) -> ()
  n29 = Bundle(w47, w22) -> (w27:cluster{dbl[], dbl[]})  [unwired: 1 in]
  n30 = property on="result" class="Str"("Visible"=FALSE) -> ()  [unwired: 2 in, 2 out]
  n31 = Build Array (concatenate)(w3, string[] ["SR-ID-IU22-05:gapMotorOff", "SR-ID-IU22A-09:gapMotorOff", "SR-ID-IU22B-09:gapMotorOff", "SR-ID-IUT22-21:gapMotorOff", "SR-ID-IU22-23:gapMotorOff", "SR-ID-IU22A-25:gapMotorOff", "SR-ID-IU22B-25:gapMotorOff", "SR-ID-EPU48A-41:gapMotorOff", "SR-ID-EPU48B-41:gapMotorOff", "SR-ID-EPU46-45:gapMotorOff", "SR-ID-EPU48A-41:phaseMotorOff", "SR-ID-EPU48B-41:phaseMotorOff", "SR-ID-EPU46-45:phaseMotorOff"]) -> (w2:string[])
  n32 = Build Array (concatenate)(w1, w10, w11, w12, w13, w2, string[] ["SR-DI-FOFB-H:setStatus", "SR-DI-FOFB-V:setStatus", "IGPF:TPSX:FBCTRL", "IGPF:TPSY:FBCTRL", "TPS-SR-022:bpm3:ilk:enabled", "SR-DI-ANGLE-ILK:StatusX", "SR-DI-ANGLE-ILK:StatusY", "SR-DI-RF-FB:setStatus", "SR-ID-EPU48-TFF:status", "SR-ID-EPU48-CFF:status", "SR-ID-EPU46-TFF:status", "SR-ID-EPU46-CFF:status"], w14) -> (w15:string[])
  "PV list" <- w15
  n33 = Get Date/Time In Seconds() -> (seconds since 1Jan1904=w7:timestamp)
  n34 = To Double Precision Float(number=w7) -> (double precision float=w5:dbl)
  "Program Start Time" <- w5
  n35 = while {
    shift-right: [w207] -> _
    shift-left: _ -> [w205]
    shift-right: [w206] -> _
    shift-left: _ -> [w204]
    shift-right: [w73] -> _
    shift-left: w27 -> [w72]
    tunnel: w5 -> [w68]
    stop <- "stop" stop-if-true
    w67 = dbl[] [1.0, 1.1666666666666667, 1.3333333333333333, 1.5, 1.6666666666666665, 1.8333333333333333, 2.0, 2.142857142857143, 2.2857142857142856, 2.4285714285714284, 2.571428571428571, 2.7142857142857144, 2.857142857142857, 3.0, 3.142857142857143, 3.2857142857142856, 3.4285714285714284, 3.571428571428571, 3.7142857142857144, 3.857142857142857, 4.0, 4.125, 4.25, 4.375, 4.5, 4.625, 4.75, 4.875, 5.0, 5.125, 5.25, 5.375, 5.5, 5.625, 5.75, 5.875, 6.0, 6.142857142857143, 6.285714285714286, 6.428571428571429, 6.571428571428571, 6.714285714285714, 6.857142857142857, 7.0, 7.142857142857143, 7.285714285714286, 7.428571428571429, 7.571428571428571, 7.714285714285714, 7.857142857142857, 8.0, 8.142857142857142, 8.285714285714286, 8.428571428571429, 8.571428571428571, 8.714285714285714, 8.857142857142858, 9.0, 9.142857142857142, 9.285714285714286, 9.428571428571429, 9.571428571428571, 9.714285714285714, 9.857142857142858, 10.0, 10.142857142857142, 10.285714285714286, 10.428571428571429, 10.571428571428571, 10.714285714285714, 10.857142857142858, 11.0, 11.142857142857142, 11.285714285714286, 11.428571428571429, 11.571428571428571, 11.714285714285714, 11.857142857142858, 12.0, 12.125, 12.25, 12.375, 12.5, 12.625, 12.75, 12.875, 13.0, 13.125, 13.25, 13.375, 13.5, 13.625, 13.75, 13.875, 14.0, 14.142857142857142, 14.285714285714286, 14.428571428571429, 14.571428571428571, 14.714285714285714, 14.857142857142858, 15.0, 15.142857142857142, 15.285714285714286, 15.428571428571429, 15.571428571428571, 15.714285714285714, 15.857142857142858, 16.0, 16.142857142857142, 16.285714285714285, 16.428571428571427, 16.571428571428573, 16.714285714285715, 16.857142857142858, 17.0, 17.142857142857142, 17.285714285714285, 17.428571428571427, 17.571428571428573, 17.714285714285715, 17.857142857142858, 18.0, 18.142857142857142, 18.285714285714285, 18.428571428571427, 18.571428571428573, 18.714285714285715, 18.857142857142858, 19.0, 19.142857142857142, 19.285714285714285, 19.428571428571427, 19.571428571428573, 19.714285714285715, 19.857142857142858, 20.0, 20.125, 20.25, 20.375, 20.5, 20.625, 20.75, 20.875, 21.0, 21.125, 21.25, 21.375, 21.5, 21.625, 21.75, 21.875, 22.0, 22.142857142857142, 22.285714285714285, 22.428571428571427, 22.571428571428573, 22.714285714285715, 22.857142857142858, 23.0, 23.142857142857142, 23.285714285714285, 23.428571428571427, 23.571428571428573, 23.714285714285715, 23.857142857142858, 24.0, 24.166666666666668, 24.333333333333332, 24.5, 24.666666666666668, 24.833333333333332]  # Array of X axis  平均分配至各段
    w98 = string[] ["SR-ID-IU22-05:setECMode", "SR-ID-IU22A-09:setECMode", "SR-ID-IU22B-09:setECMode", "SR-ID-IUT22-21:setECMode", "SR-ID-IU22-23:setECMode", "SR-ID-IU22A-25:setECMode", "SR-ID-IU22B-25:setECMode", "SR-ID-EPU48A-41:setECMode", "SR-ID-EPU48B-41:setECMode", "SR-ID-EPU46-45:setECMode"]  # ID_mode
    w184 = string[] ["FE-05-PAB:Open", "FE-05-MGV:Open", "FE-05-FCV:Open", "FE-09-PAB:Open", "FE-09-MGV:Open", "FE-09-FCV:Open", "FE-21-PAB:Open", "FE-21-MGV:Open", "FE-21-FCV:Open", "FE-23-PAB:Open", "FE-23-PAB:Open", "FE-23-FCV:Open", "FE-25-PAB:Open", "FE-25-MGV:Open", "FE-25-FCV:Open", "FE-41-PAB:Open", "FE-41-MGV:Open", "FE-41-FCV:Open", "FE-45-PAB:Open", "FE-45-MGV:Open", "FE-45-FCV:Open"]  # PAB_MGV_FCV enable
    (unwired) "LI-DI-WCM:getWfCh1"
    (unwired) "SR-DI-FP:CurrentBuffer"
    w323 = 0.001
    w321 = string[] ["SR-DI-BPM-011:Y", "SR-DI-BPM-012:Y", "SR-DI-BPM-013:Y", "SR-DI-BPM-014:Y", "SR-DI-BPM-015:Y", "SR-DI-BPM-016:Y", "SR-DI-BPM-017:Y", "SR-DI-BPM-021:Y", "SR-DI-BPM-022:Y", "SR-DI-BPM-023:Y", "SR-DI-BPM-024:Y", "SR-DI-BPM-025:Y", "SR-DI-BPM-026:Y", "SR-DI-BPM-027:Y", "SR-DI-BPM-031:Y", "SR-DI-BPM-032:Y", "SR-DI-BPM-033:Y", "SR-DI-BPM-034:Y", "SR-DI-BPM-035:Y", "SR-DI-BPM-036:Y", "SR-DI-BPM-037:Y", "SR-DI-BPM-041:Y", "SR-DI-BPM-042:Y", "SR-DI-BPM-043:Y", "SR-DI-BPM-044:Y", "SR-DI-BPM-045:Y", "SR-DI-BPM-046:Y", "SR-DI-BPM-047:Y", "SR-DI-BPM-048:Y", "SR-DI-BPM-050:Y", "SR-DI-BPM-051:Y", "SR-DI-BPM-052:Y", "SR-DI-BPM-053:Y", "SR-DI-BPM-054:Y", "SR-DI-BPM-055:Y", "SR-DI-BPM-056:Y", "SR-DI-BPM-057:Y", "SR-DI-BPM-061:Y", "SR-DI-BPM-062:Y", "SR-DI-BPM-063:Y", "SR-DI-BPM-064:Y", "SR-DI-BPM-065:Y", "SR-DI-BPM-066:Y", "SR-DI-BPM-067:Y", "SR-DI-BPM-071:Y", "SR-DI-BPM-072:Y", "SR-DI-BPM-073:Y", "SR-DI-BPM-074:Y", "SR-DI-BPM-075:Y", "SR-DI-BPM-076:Y", "SR-DI-BPM-077:Y", "SR-DI-BPM-081:Y", "SR-DI-BPM-082:Y", "SR-DI-BPM-083:Y", "SR-DI-BPM-084:Y", "SR-DI-BPM-085:Y", "SR-DI-BPM-086:Y", "SR-DI-BPM-087:Y", "SR-DI-BPM-091:Y", "SR-DI-BPM-092:Y", "SR-DI-BPM-093:Y", "SR-DI-BPM-094:Y", "SR-DI-BPM-095:Y", "SR-DI-BPM-096:Y", "SR-DI-BPM-097:Y", "SR-DI-BPM-101:Y", "SR-DI-BPM-102:Y", "SR-DI-BPM-103:Y", "SR-DI-BPM-104:Y", "SR-DI-BPM-105:Y", "SR-DI-BPM-106:Y", "SR-DI-BPM-107:Y", "SR-DI-BPM-111:Y", "SR-DI-BPM-112:Y", "SR-DI-BPM-113:Y", "SR-DI-BPM-114:Y", "SR-DI-BPM-115:Y", "SR-DI-BPM-116:Y", "SR-DI-BPM-117:Y", "SR-DI-BPM-121:Y", "SR-DI-BPM-122:Y", "SR-DI-BPM-123:Y", "SR-DI-BPM-124:Y", "SR-DI-BPM-125:Y", "SR-DI-BPM-126:Y", "SR-DI-BPM-127:Y", "SR-DI-BPM-128:Y", "SR-DI-BPM-130:Y", "SR-DI-BPM-131:Y", "SR-DI-BPM-132:Y", "SR-DI-BPM-133:Y", "SR-DI-BPM-134:Y", "SR-DI-BPM-135:Y", "SR-DI-BPM-136:Y", "SR-DI-BPM-137:Y", "SR-DI-BPM-141:Y", "SR-DI-BPM-142:Y", "SR-DI-BPM-143:Y", "SR-DI-BPM-144:Y", "SR-DI-BPM-145:Y", "SR-DI-BPM-146:Y", "SR-DI-BPM-147:Y", "SR-DI-BPM-151:Y", "SR-DI-BPM-152:Y", "SR-DI-BPM-153:Y", "SR-DI-BPM-154:Y", "SR-DI-BPM-155:Y", "SR-DI-BPM-156:Y", "SR-DI-BPM-157:Y", "SR-DI-BPM-161:Y", "SR-DI-BPM-162:Y", "SR-DI-BPM-163:Y", "SR-DI-BPM-164:Y", "SR-DI-BPM-165:Y", "SR-DI-BPM-166:Y", "SR-DI-BPM-167:Y", "SR-DI-BPM-171:Y", "SR-DI-BPM-172:Y", "SR-DI-BPM-173:Y", "SR-DI-BPM-174:Y", "SR-DI-BPM-175:Y", "SR-DI-BPM-176:Y", "SR-DI-BPM-177:Y", "SR-DI-BPM-181:Y", "SR-DI-BPM-182:Y", "SR-DI-BPM-183:Y", "SR-DI-BPM-184:Y", "SR-DI-BPM-185:Y", "SR-DI-BPM-186:Y", "SR-DI-BPM-187:Y", "SR-DI-BPM-191:Y", "SR-DI-BPM-192:Y", "SR-DI-BPM-193:Y", "SR-DI-BPM-194:Y", "SR-DI-BPM-195:Y", "SR-DI-BPM-196:Y", "SR-DI-BPM-197:Y", "SR-DI-BPM-201:Y", "SR-DI-BPM-202:Y", "SR-DI-BPM-203:Y", "SR-DI-BPM-204:Y", "SR-DI-BPM-205:Y", "SR-DI-BPM-206:Y", "SR-DI-BPM-207:Y", "SR-DI-BPM-208:Y", "SR-DI-BPM-210:Y", "SR-DI-BPM-211:Y", "SR-DI-BPM-212:Y", "SR-DI-BPM-213:Y", "SR-DI-BPM-214:Y", "SR-DI-BPM-215:Y", "SR-DI-BPM-216:Y", "SR-DI-BPM-217:Y", "SR-DI-BPM-221:Y", "SR-DI-BPM-222:Y", "SR-DI-BPM-223:Y", "SR-DI-BPM-224:Y", "SR-DI-BPM-225:Y", "SR-DI-BPM-226:Y", "SR-DI-BPM-227:Y", "SR-DI-BPM-231:Y", "SR-DI-BPM-232:Y", "SR-DI-BPM-233:Y", "SR-DI-BPM-234:Y", "SR-DI-BPM-235:Y", "SR-DI-BPM-236:Y", "SR-DI-BPM-237:Y", "SR-DI-BPM-241:Y", "SR-DI-BPM-242:Y", "SR-DI-BPM-243:Y", "SR-DI-BPM-244:Y", "SR-DI-BPM-245:Y", "SR-DI-BPM-246:Y", "SR-DI-BPM-247:Y"]  # sorted BPMY_174
    w320 = string[] ["SR-DI-BPM-011:X", "SR-DI-BPM-012:X", "SR-DI-BPM-013:X", "SR-DI-BPM-014:X", "SR-DI-BPM-015:X", "SR-DI-BPM-016:X", "SR-DI-BPM-017:X", "SR-DI-BPM-021:X", "SR-DI-BPM-022:X", "SR-DI-BPM-023:X", "SR-DI-BPM-024:X", "SR-DI-BPM-025:X", "SR-DI-BPM-026:X", "SR-DI-BPM-027:X", "SR-DI-BPM-031:X", "SR-DI-BPM-032:X", "SR-DI-BPM-033:X", "SR-DI-BPM-034:X", "SR-DI-BPM-035:X", "SR-DI-BPM-036:X", "SR-DI-BPM-037:X", "SR-DI-BPM-041:X", "SR-DI-BPM-042:X", "SR-DI-BPM-043:X", "SR-DI-BPM-044:X", "SR-DI-BPM-045:X", "SR-DI-BPM-046:X", "SR-DI-BPM-047:X", "SR-DI-BPM-048:X", "SR-DI-BPM-050:X", "SR-DI-BPM-051:X", "SR-DI-BPM-052:X", "SR-DI-BPM-053:X", "SR-DI-BPM-054:X", "SR-DI-BPM-055:X", "SR-DI-BPM-056:X", "SR-DI-BPM-057:X", "SR-DI-BPM-061:X", "SR-DI-BPM-062:X", "SR-DI-BPM-063:X", "SR-DI-BPM-064:X", "SR-DI-BPM-065:X", "SR-DI-BPM-066:X", "SR-DI-BPM-067:X", "SR-DI-BPM-071:X", "SR-DI-BPM-072:X", "SR-DI-BPM-073:X", "SR-DI-BPM-074:X", "SR-DI-BPM-075:X", "SR-DI-BPM-076:X", "SR-DI-BPM-077:X", "SR-DI-BPM-081:X", "SR-DI-BPM-082:X", "SR-DI-BPM-083:X", "SR-DI-BPM-084:X", "SR-DI-BPM-085:X", "SR-DI-BPM-086:X", "SR-DI-BPM-087:X", "SR-DI-BPM-091:X", "SR-DI-BPM-092:X", "SR-DI-BPM-093:X", "SR-DI-BPM-094:X", "SR-DI-BPM-095:X", "SR-DI-BPM-096:X", "SR-DI-BPM-097:X", "SR-DI-BPM-101:X", "SR-DI-BPM-102:X", "SR-DI-BPM-103:X", "SR-DI-BPM-104:X", "SR-DI-BPM-105:X", "SR-DI-BPM-106:X", "SR-DI-BPM-107:X", "SR-DI-BPM-111:X", "SR-DI-BPM-112:X", "SR-DI-BPM-113:X", "SR-DI-BPM-114:X", "SR-DI-BPM-115:X", "SR-DI-BPM-116:X", "SR-DI-BPM-117:X", "SR-DI-BPM-121:X", "SR-DI-BPM-122:X", "SR-DI-BPM-123:X", "SR-DI-BPM-124:X", "SR-DI-BPM-125:X", "SR-DI-BPM-126:X", "SR-DI-BPM-127:X", "SR-DI-BPM-128:X", "SR-DI-BPM-130:X", "SR-DI-BPM-131:X", "SR-DI-BPM-132:X", "SR-DI-BPM-133:X", "SR-DI-BPM-134:X", "SR-DI-BPM-135:X", "SR-DI-BPM-136:X", "SR-DI-BPM-137:X", "SR-DI-BPM-141:X", "SR-DI-BPM-142:X", "SR-DI-BPM-143:X", "SR-DI-BPM-144:X", "SR-DI-BPM-145:X", "SR-DI-BPM-146:X", "SR-DI-BPM-147:X", "SR-DI-BPM-151:X", "SR-DI-BPM-152:X", "SR-DI-BPM-153:X", "SR-DI-BPM-154:X", "SR-DI-BPM-155:X", "SR-DI-BPM-156:X", "SR-DI-BPM-157:X", "SR-DI-BPM-161:X", "SR-DI-BPM-162:X", "SR-DI-BPM-163:X", "SR-DI-BPM-164:X", "SR-DI-BPM-165:X", "SR-DI-BPM-166:X", "SR-DI-BPM-167:X", "SR-DI-BPM-171:X", "SR-DI-BPM-172:X", "SR-DI-BPM-173:X", "SR-DI-BPM-174:X", "SR-DI-BPM-175:X", "SR-DI-BPM-176:X", "SR-DI-BPM-177:X", "SR-DI-BPM-181:X", "SR-DI-BPM-182:X", "SR-DI-BPM-183:X", "SR-DI-BPM-184:X", "SR-DI-BPM-185:X", "SR-DI-BPM-186:X", "SR-DI-BPM-187:X", "SR-DI-BPM-191:X", "SR-DI-BPM-192:X", "SR-DI-BPM-193:X", "SR-DI-BPM-194:X", "SR-DI-BPM-195:X", "SR-DI-BPM-196:X", "SR-DI-BPM-197:X", "SR-DI-BPM-201:X", "SR-DI-BPM-202:X", "SR-DI-BPM-203:X", "SR-DI-BPM-204:X", "SR-DI-BPM-205:X", "SR-DI-BPM-206:X", "SR-DI-BPM-207:X", "SR-DI-BPM-208:X", "SR-DI-BPM-210:X", "SR-DI-BPM-211:X", "SR-DI-BPM-212:X", "SR-DI-BPM-213:X", "SR-DI-BPM-214:X", "SR-DI-BPM-215:X", "SR-DI-BPM-216:X", "SR-DI-BPM-217:X", "SR-DI-BPM-221:X", "SR-DI-BPM-222:X", "SR-DI-BPM-223:X", "SR-DI-BPM-224:X", "SR-DI-BPM-225:X", "SR-DI-BPM-226:X", "SR-DI-BPM-227:X", "SR-DI-BPM-231:X", "SR-DI-BPM-232:X", "SR-DI-BPM-233:X", "SR-DI-BPM-234:X", "SR-DI-BPM-235:X", "SR-DI-BPM-236:X", "SR-DI-BPM-237:X", "SR-DI-BPM-241:X", "SR-DI-BPM-242:X", "SR-DI-BPM-243:X", "SR-DI-BPM-244:X", "SR-DI-BPM-245:X", "SR-DI-BPM-246:X", "SR-DI-BPM-247:X"]  # sorted BPMX_174
    w379 = string[] ["BL-05A:HutchA_Enable", "BL-09A:HutchA_Enable", "BL-21A:HutchA_Enable", "BL-23A:HutchA_Enable", "BL-25A:HutchA_Enable", "BL-41A:HutchA_Enable", "BL-45A:HutchA_Enable"]  # Hutch enable
    w398 = string[] ["CPCI03-adl7452-0:doBank0Ch5", "CPCI05-adl7452-0:doBank0Ch5", "CPCI11-adl7452-0:doBank0Ch5", "CPCI12-adl7452-0:doBank0Ch5", "CPCI13-adl7452-0:doBank0Ch5", "CPCI21-adl7452-0:doBank0Ch5", "CPCI23-adl7452-0:doBank0Ch5"]  # FE enable
    (unwired) 1 ("index")
    w475 = 578.303 ("y")
    w480 = 1.202 ("y")
    # "SR-DI-RF-FB:getStatus"
    # "V1.4.2 改成直接用最大最小值當作scale的最大最小值"
    # "D:\\LOG運轉紀錄\\2016"
    # "45"
    # "41"
    # "25"
    # "23"
    # "21"
    # "09"
    # "05"
    # "0為"
    # "05\n09\n21\n23\n25\n41\n45"
    # "gapMotorOff"
    n36 = event shown="[3] \"Trip Evt B\": Value Change" {
      selector: _ -> [_ _ _ _ _ _ _ _ _ _]
      dyn-events: _ -> [_ _ _ _ _ _ _ _ _ _]
      timeout: 233 -> [_ _ _ _ _ _ _ _ _ _]
      tunnel: [_ w514 _ _ _ _ _ _ _ _] -> w74
      tunnel: [w499 w513 w520 w536 w675 w812 w824 w850 w887 w892] -> w73
      tunnel: w72 -> [w499 w513 w520 _ _ w812 w824 w850 w887 w892]
      tunnel: "last ? Hrs" -> [_ _ _ w537 w676 _ _ _ _ _]
      tunnel: w68 -> [_ w500 _ _ _ _ w823 _ w877 _]
      event Timeout {
        n37 = event-data() -> ()  [unwired: 1 in, 3 out]
      }
      event "stop": Value Change {
        n38 = event-data() -> ("NewVal"=w514:bool)  [unwired: 1 in, 3 out]
        n39 = Get Date/Time In Seconds() -> (seconds since 1Jan1904=w507:timestamp)
        n40 = To Double Precision Float(number=w507) -> (double precision float=w506:dbl)
        n41 = Subtract(x=w506, y=43200.0) -> (x-y=w503:dbl)
        n42 = call "Main_Daily_path.vi"() -> ("Directory path"=w508:path)  [unwired: 10 in, 1 out]
        n43 = Greater?(x=w503, y=w500) -> (0:w504:bool)
        n44 = Select(t=w503, s=w504, f=w500) -> (s? t:f=w502:dbl)
        n45 = call "B09_Save_new_lattice_files.vi"("For Test"=FALSE, "Directory Path"=w508) -> ()  [unwired: 10 in]
        n46 = call <vilib>:"Application Directory.vi"() -> ("Application Directory"=w501:path)
        n47 = local read "Diff list"() -> (w511:string[][])
        n48 = call "B07_Save_changed_PVs.vi"("For Test"=FALSE, "想要限制的筆數"=1000, "Directory Path"=w501, "紀錄起始時間  門檻"=w502, "diff_Value 2"=w511) -> ()  [unwired: 5 in, 2 out]
      }
      event "Open Button": Value Change {
        n49 = event-data() -> ()  [unwired: 1 in, 6 out]
        n50 = call <vilib>:"Beep.vi"("use system alert? (T)"=FALSE, "duration (msec)"=u32 40, "frequency (Hz)"=u32 1700) -> ()  [unwired: 9 in]
        n51 = call "Main_Daily_path.vi"() -> ("Directory path(STR)"=w519:string, "Directory path"=w518:path)  [unwired: 10 in]
        n52 = call <vilib>:"Check if File or Folder Exists.vi"("path"=w518) -> ("error out"=w524:errorcluster, "file or folder exists?"=w522:bool, "dup path"=w523:path)  [unwired: 8 in]
        n53 = case shown="False" w522 {
          tunnel: w523 -> [w531 w533]
          tunnel: w524 -> [w530 w532]
          tunnel: [w529 w533] -> _
          tunnel: [w528 w532] -> w521
          frame False {
            n54 = Create Folder(path (use dialog)=w531, error in=w530) -> (created path=w529:path, error out=w528:errorcluster)  [unwired: 1 in, 1 out]
          }
          frame True {
          }
        }
        n55 = Concatenate Strings("explorer ", w519) -> (w526:string)
        n56 = call <vilib>:"System Exec.vi"("wait until completion? (T)"=FALSE, "error in (no error)"=w521, "command line"=w526) -> ()  [unwired: 5 in, 4 out]
      }
      event "Trip Evt B": Value Change {
        n57 = event-data() -> ()  [unwired: 1 in, 1 out]
        n58 = flat-sequence {
          tunnel: w537 -> [w542]
          tunnel: [w542] -> w534
          tunnel: [w558] -> w535
          tunnel: w534 -> [w561]
          tunnel: [w672] -> w536
          tunnel: w535 -> [w672]
          frame #0 {
            n59 = property on="result" class="Str"("Visible"=FALSE) -> ()  [unwired: 2 in, 2 out]
            n60 = call <vilib>:"Beep.vi"("use system alert? (T)"=FALSE, "duration (msec)"=u32 40, "frequency (Hz)"=u32 1700) -> ()  [unwired: 9 in]
          }
          frame #1 {
            n61 = Get Date/Time In Seconds() -> (seconds since 1Jan1904=w565:timestamp)
            n62 = Multiply(x=3600.0 ("y"), y=w561) -> (x*y=w574:dbl)
            n63 = call "TimeToString.vi"("Time Stamp Control"=w565) -> ("result string"=w572:string)
            n64 = Subtract(x=w565, y=w574) -> (x-y=w566:timestamp)
            n65 = call "TimeToString.vi"("Time Stamp Control"=w566) -> ("result string"=w573:string)
            n66 = call <vilib>:"Application Directory.vi"() -> ("Application Directory"=w571:path)
            n67 = Build Path(base path=w571, name or relative path="DSN\\172-18-0-32.dsn") -> (appended path=w569:path)
            n68 = Concatenate Strings("SELECT  float_val , smpl_time\nFROM sample \nwhere  channel_id = 104 and smpl_time between '" ("result string"), w573, "' ::timestamp and '" ("result string"), w572, "' ::timestamp" ("result string")) -> (w586:string)
            n69 = call-poly <vilib>:"DB Tools Open Connection.vi"("connection information"=w569) -> ("error out"=w576:errorcluster, "connection reference"=w577:T2)  [unwired: 7 in]
            n70 = call-poly <vilib>:"DB Tools Execute Query.vi"("error in (no error)"=w576, "SQL query"=w586, "connection reference"=w577) -> ("error out"=w579:errorcluster, "recordset reference"=w578:T3)  [unwired: 5 in]
            n71 = call-poly <vilib>:"DB Tools Fetch Recordset Data.vi"("error in (no error)"=w579, "recordset reference"=w578) -> ("error out"=w562:errorcluster, "recordset data"=w545:variant[][], "recordset reference out"=w580:T3)  [unwired: 3 in]
            n72 = call-poly <vilib>:"DB Tools Free Object.vi"("error in (no error)"=w562, "recordset reference"=w580) -> ("error out"=w582:errorcluster, "connection reference"=w581:T2)  [unwired: 8 in]
            n73 = Transpose 2D Array(2D array=w545) -> (transposed array=w549:variant[][])
            n74 = call <vilib>:"DB Tools Close Connection.vi"("error in (no error)"=w582, "connection reference"=w581) -> ("error out"=→"error out 4":errorcluster)  [unwired: 5 in]
            n75 = Index Array(array=w549, index (row) #1=1 ("index (row)"), index (row) #2=0 ("index (row)")) -> (element #1=w551:variant[], element #2=w552:variant[])  [unwired: 2 in]
            n76 = xnode "Database Variant To Data"("database variant"=w551, "type"=timestamp[] []) -> ("data"=w544:timestamp[])  [unwired: 1 in, 1 out]
            n77 = Variant To Data(type=dbl[] [], Variant=w552) -> (data=w543:dbl[])  [unwired: 1 in, 1 out]
            n78 = control-ref of="BeamCurrent History"() -> (w560:refnum<vi>)
            n79 = for {
              tunnel: w543 -> [w665] mode=indexing
              tunnel: w544 -> [w664] mode=indexing
              shift-right: [w665] -> _
              shift-left: 0.0 -> [w666]
              tunnel: [w664] -> w588 mode=indexing if=w663
              tunnel: [w662] -> _ mode=indexing
              n80 = Subtract(x=w665, y=w666) -> (x-y=w662:dbl)
              n81 = Less Or Equal?(x=w662, y=-100.0) -> (x <= y?=w663:bool)
            }
            n82 = To Double Precision Float(number=w544) -> (double precision float=w559:dbl[])
            n83 = To Double Precision Float(number=w565) -> (double precision float=w567:dbl)
            n84 = Array Max & Min(array=w543) -> (max value=w564:dbl, min value=w563:dbl)  [unwired: 2 out]
            n85 = To Double Precision Float(number=w566) -> (double precision float=w568:dbl)
            n86 = property on="Property Node" class="XYGraph (strict)"(reference=w560, "XScale.Maximum"=w567, "XScale.Minimum"=w568, "YScale.Maximum"=w564, "YScale.Minimum"=w563) -> ()  [unwired: 1 in, 2 out]
            n87 = Bundle(w559, w543) -> (w558:cluster{dbl[], dbl[]})  [unwired: 1 in]
            n88 = Array Size(array=w588) -> (size(s)=w555:i32)
            n89 = for {
              tunnel: w588 -> [w659] mode=indexing
              tunnel: [w655] -> w589 mode=indexing
              i -> [w658]
              n90 = Increment(x=w658) -> (x+1=w657:i32)
              n91 = Format Date/Time String(time format string (%c)="%Y/%m/%d %H:%M", seconds (now)=w659) -> (date/time string=w656:string)  [unwired: 1 in]
              n92 = Number To Decimal String(number=w657) -> (decimal integer string=w654:string)  [unwired: 1 in]
              n93 = Concatenate Strings(w654, "." ("string")) -> (w652:string)
              n94 = Build Array(w652, w656) -> (w655:string[])
            }
            n95 = Number To Decimal String(number=w555) -> (decimal integer string=w595:string)  [unwired: 1 in]
            n96 = Build Array (concatenate)(string[] ["No.", "Event Time"], w589) -> (w593:string[][])
            n97 = Array To Spreadsheet String(delimiter (Tab)="", array=w593, 3:"%s" ("format string")) -> (spreadsheet string=w597:string)
            n98 = Concatenate Strings("Beam Trip Events \nTatal Counts: ", w595, "\n" ("string"), w597, "\n(Threshold:100mA)") -> (w554:string)
            n99 = case shown="0" w555 {
              tunnel: ["Beam Trip Events \nTotal Counts: 0" w651] -> w553
              tunnel: w554 -> [_ w651]
              frame 0 {
              }
              frame 1, Default {
              }
            }
            "result" <- w553
          }
          frame #2 {
            n100 = local write "Trip Evt B"(FALSE ("Trip Evt B")) -> ()
            n101 = property on="result" class="Str"("Visible"=TRUE) -> ()  [unwired: 2 in, 2 out]
            n102 = call <vilib>:"Beep.vi"("use system alert? (T)"=FALSE, "duration (msec)"=u32 40, "frequency (Hz)"=u32 2000) -> ()  [unwired: 9 in]
          }
        }
      }
      event "Refresh B": Value Change {
        n103 = event-data() -> ()  [unwired: 1 in, 6 out]
        n104 = flat-sequence {
          tunnel: w676 -> [w681]
          tunnel: [w681] -> w673
          tunnel: [w697] -> w674
          tunnel: w673 -> [w700]
          tunnel: [w811] -> w675
          tunnel: w674 -> [w811]
          frame #0 {
            n105 = property on="result" class="Str"("Visible"=FALSE) -> ()  [unwired: 2 in, 2 out]
            n106 = call <vilib>:"Beep.vi"("use system alert? (T)"=FALSE, "duration (msec)"=u32 40, "frequency (Hz)"=u32 1700) -> ()  [unwired: 9 in]
          }
          frame #1 {
            n107 = Get Date/Time In Seconds() -> (seconds since 1Jan1904=w704:timestamp)
            n108 = Multiply(x=3600.0 ("y"), y=w700) -> (x*y=w713:dbl)
            n109 = call "TimeToString.vi"("Time Stamp Control"=w704) -> ("result string"=w711:string)
            n110 = Subtract(x=w704, y=w713) -> (x-y=w705:timestamp)
            n111 = call "TimeToString.vi"("Time Stamp Control"=w705) -> ("result string"=w712:string)
            n112 = call <vilib>:"Application Directory.vi"() -> ("Application Directory"=w710:path)
            n113 = Build Path(base path=w710, name or relative path="DSN\\172-18-0-32.dsn") -> (appended path=w708:path)
            n114 = Concatenate Strings("SELECT  float_val , smpl_time\nFROM sample \nwhere  channel_id = 104 and smpl_time between '" ("result string"), w712, "' ::timestamp and '" ("result string"), w711, "' ::timestamp" ("result string")) -> (w725:string)
            n115 = call-poly <vilib>:"DB Tools Open Connection.vi"("connection information"=w708) -> ("error out"=w715:errorcluster, "connection reference"=w716:T2)  [unwired: 7 in]
            n116 = call-poly <vilib>:"DB Tools Execute Query.vi"("error in (no error)"=w715, "SQL query"=w725, "connection reference"=w716) -> ("error out"=w718:errorcluster, "recordset reference"=w717:T3)  [unwired: 5 in]
            n117 = call-poly <vilib>:"DB Tools Fetch Recordset Data.vi"("error in (no error)"=w718, "recordset reference"=w717) -> ("error out"=w701:errorcluster, "recordset data"=w684:variant[][], "recordset reference out"=w719:T3)  [unwired: 3 in]
            n118 = call-poly <vilib>:"DB Tools Free Object.vi"("error in (no error)"=w701, "recordset reference"=w719) -> ("error out"=w721:errorcluster, "connection reference"=w720:T2)  [unwired: 8 in]
            n119 = Transpose 2D Array(2D array=w684) -> (transposed array=w688:variant[][])
            n120 = call <vilib>:"DB Tools Close Connection.vi"("error in (no error)"=w721, "connection reference"=w720) -> ("error out"=→"error out 5":errorcluster)  [unwired: 5 in]
            n121 = Index Array(array=w688, index (row) #1=1 ("index (row)"), index (row) #2=0 ("index (row)")) -> (element #1=w690:variant[], element #2=w691:variant[])  [unwired: 2 in]
            n122 = xnode "Database Variant To Data"("database variant"=w690, "type"=timestamp[] []) -> ("data"=w683:timestamp[])  [unwired: 1 in, 1 out]
            n123 = Variant To Data(type=dbl[] [], Variant=w691) -> (data=w682:dbl[])  [unwired: 1 in, 1 out]
            n124 = control-ref of="BeamCurrent History"() -> (w699:refnum<vi>)
            n125 = for {
              tunnel: w682 -> [w804] mode=indexing
              tunnel: w683 -> [w803] mode=indexing
              shift-right: [w804] -> _
              shift-left: 0.0 -> [w805]
              tunnel: [w803] -> w727 mode=indexing if=w802
              tunnel: [w801] -> _ mode=indexing
              n126 = Subtract(x=w804, y=w805) -> (x-y=w801:dbl)
              n127 = Less Or Equal?(x=w801, y=-100.0) -> (x <= y?=w802:bool)
            }
            n128 = To Double Precision Float(number=w683) -> (double precision float=w698:dbl[])
            n129 = To Double Precision Float(number=w704) -> (double precision float=w706:dbl)
            n130 = Array Max & Min(array=w682) -> (max value=w703:dbl, min value=w702:dbl)  [unwired: 2 out]
            n131 = To Double Precision Float(number=w705) -> (double precision float=w707:dbl)
            n132 = property on="Property Node" class="XYGraph (strict)"(reference=w699, "XScale.Maximum"=w706, "XScale.Minimum"=w707, "YScale.Maximum"=w703, "YScale.Minimum"=w702) -> ()  [unwired: 1 in, 2 out]
            n133 = Bundle(w698, w682) -> (w697:cluster{dbl[], dbl[]})  [unwired: 1 in]
            n134 = Array Size(array=w727) -> (size(s)=w694:i32)
            n135 = for {
              tunnel: w727 -> [w798] mode=indexing
              tunnel: [w794] -> w728 mode=indexing
              i -> [w797]
              n136 = Increment(x=w797) -> (x+1=w796:i32)
              n137 = Format Date/Time String(time format string (%c)="%Y/%m/%d %H:%M", seconds (now)=w798) -> (date/time string=w795:string)  [unwired: 1 in]
              n138 = Number To Decimal String(number=w796) -> (decimal integer string=w793:string)  [unwired: 1 in]
              n139 = Concatenate Strings(w793, "." ("string")) -> (w791:string)
              n140 = Build Array(w791, w795) -> (w794:string[])
            }
            n141 = Number To Decimal String(number=w694) -> (decimal integer string=w734:string)  [unwired: 1 in]
            n142 = Build Array (concatenate)(string[] ["No.", "Event Time"], w728) -> (w732:string[][])
            n143 = Array To Spreadsheet String(delimiter (Tab)="", array=w732, 3:"%s" ("format string")) -> (spreadsheet string=w736:string)
            n144 = Concatenate Strings("Beam Trip Events \nTatal Counts: ", w734, "\n" ("string"), w736, "\n(Threshold:100mA)") -> (w693:string)
            n145 = case shown="0" w694 {
              tunnel: ["Beam Trip Events \nTotal Counts: 0" w790] -> w692
              tunnel: w693 -> [_ w790]
              frame 0 {
              }
              frame 1, Default {
              }
            }
            n146 = local write "result"(w692) -> ()
          }
          frame #2 {
            n147 = local write "Refresh B"(FALSE ("Trip Evt B")) -> ()
            n148 = property on="result" class="Str"("Visible"=TRUE) -> ()  [unwired: 2 in, 2 out]
            n149 = call <vilib>:"Beep.vi"("use system alert? (T)"=FALSE, "duration (msec)"=u32 40, "frequency (Hz)"=u32 2000) -> ()  [unwired: 9 in]
          }
        }
      }
      event "Save Lattice Button": Value Change {
        n150 = event-data() -> ()  [unwired: 1 in, 2 out]
        n151 = flat-sequence {
          frame #0 {
            n152 = call <vilib>:"Beep.vi"("use system alert? (T)"=FALSE, "duration (msec)"=u32 40, "frequency (Hz)"=u32 1700) -> ()  [unwired: 9 in]
          }
          frame #1 {
            n153 = call "Main_Daily_path.vi"() -> ("Directory path"=w816:path)  [unwired: 10 in, 1 out]
            n154 = call "B09_Save_new_lattice_files.vi"("For Test"=FALSE, "Directory Path"=w816) -> ()  [unwired: 10 in]
          }
          frame #2 {
            n155 = call <vilib>:"Beep.vi"("use system alert? (T)"=FALSE, "duration (msec)"=u32 40, "frequency (Hz)"=u32 2000) -> ()  [unwired: 9 in]
          }
        }
      }
      event "View Diff Button": Value Change {
        n156 = event-data() -> ()  [unwired: 1 in, 1 out]
        n157 = flat-sequence {
          tunnel: w823 -> [w829]
          tunnel: [w835] -> w821
          tunnel: [w840] -> w822
          tunnel: w821 -> [w840]
          tunnel: w822 -> [w842]
          frame #0 {
            # "12小時為43200sec"
            # "Save file"
            n158 = Get Date/Time In Seconds() -> (seconds since 1Jan1904=w834:timestamp)
            n159 = To Double Precision Float(number=w834) -> (double precision float=w833:dbl)
            n160 = call <vilib>:"Beep.vi"("use system alert? (T)"=FALSE, "duration (msec)"=u32 40, "frequency (Hz)"=u32 1700) -> ()  [unwired: 9 in]
            n161 = Subtract(x=w833, y=43200.0) -> (x-y=w830:dbl)
            n162 = Greater?(x=w830, y=w829) -> (0:w831:bool)
            n163 = Select(t=w830, s=w831, f=w829) -> (s? t:f=w828:dbl)
            n164 = local read "Diff list"() -> (w839:string[][])
            n165 = call "Main_Daily_path.vi"() -> ("Directory path"=w838:path)  [unwired: 10 in, 1 out]
            n166 = call "B07_Save_changed_PVs.vi"("For Test"=FALSE, "想要限制的筆數"=1000, "Directory Path"=w838, "紀錄起始時間  門檻"=w828, "diff_Value 2"=w839) -> ("saved file path"=w835:path)  [unwired: 5 in, 1 out]
          }
          frame #1 {
            # "Wait"
            n167 = Wait (ms)(milliseconds to wait=u32 300) -> ()  [unwired: 1 out]
          }
          frame #2 {
            # "Show"
            n168 = Path To String(path=w842) -> (string=w844:string)
            n169 = Concatenate Strings("explorer ", w844) -> (w843:string)
            n170 = call <vilib>:"System Exec.vi"("command line"=w843) -> ()  [unwired: 7 in, 4 out]
          }
          frame #3 {
            n171 = local write "View Diff Button"(FALSE ("View Diff Button")) -> ()
            n172 = call <vilib>:"Beep.vi"("use system alert? (T)"=FALSE, "duration (msec)"=u32 40, "frequency (Hz)"=u32 2000) -> ()  [unwired: 9 in]
          }
        }
      }
      event "Show Check list Button": Value Change {
        n173 = event-data() -> ()  [unwired: 1 in, 1 out]
        n174 = flat-sequence {
          frame #0 {
            n175 = call <vilib>:"Beep.vi"("use system alert? (T)"=FALSE, "duration (msec)"=u32 40, "frequency (Hz)"=u32 1700) -> ()  [unwired: 9 in]
          }
          frame #1 {
            n176 = local read "PV list"() -> (w854:string[])
            n177 = Array Size(array=w854) -> (size(s)=w855:i32)
            n178 = Array To Spreadsheet String(delimiter (Tab)="</BR>\n\r", array=w854, 3:"%s" ("format string")) -> (spreadsheet string=w866:string)
            n179 = Number To Decimal String(number=w855) -> (decimal integer string=w865:string)  [unwired: 1 in]
            n180 = call <vilib>:"Application Directory.vi"() -> ("Application Directory"=w856:path)
            n181 = Concatenate Strings("Tatal Checked PVs: ", w865, "</BR>\n\r" ("string"), w866) -> (w867:string)
            n182 = Build Path(base path=w856, name or relative path="Checked PV list.html") -> (appended path=w868:path)
            n183 = Write to Text File(file (use dialog)=w868, text=w867) -> ()  [unwired: 2 in, 3 out]
            n184 = flat-sequence {
              tunnel: w868 -> [w870]
              tunnel: [w870] -> w869
              frame #0 {
                n185 = Wait (ms)(milliseconds to wait=u32 500) -> ()  [unwired: 1 out]
              }
            }
            n186 = Path To String(path=w869) -> (string=w859:string)
            n187 = Concatenate Strings("explorer ", w859) -> (w858:string)
            n188 = call <vilib>:"System Exec.vi"("command line"=w858) -> ()  [unwired: 7 in, 4 out]
          }
          frame #2 {
            n189 = call <vilib>:"Beep.vi"("use system alert? (T)"=FALSE, "duration (msec)"=u32 40, "frequency (Hz)"=u32 2000) -> ()  [unwired: 9 in]
          }
        }
      }
      event Panel Close {
        n190 = event-data() -> ()  [unwired: 1 in, 2 out]
        n191 = Get Date/Time In Seconds() -> (seconds since 1Jan1904=w882:timestamp)
        n192 = To Double Precision Float(number=w882) -> (double precision float=w881:dbl)
        n193 = Subtract(x=w881, y=43200.0) -> (x-y=w878:dbl)
        n194 = call "Main_Daily_path.vi"() -> ("Directory path"=w883:path)  [unwired: 10 in, 1 out]
        n195 = Greater?(x=w878, y=w877) -> (0:w879:bool)
        n196 = Select(t=w878, s=w879, f=w877) -> (s? t:f=w876:dbl)
        n197 = call "B09_Save_new_lattice_files.vi"("For Test"=FALSE, "Directory Path"=w883) -> ()  [unwired: 10 in]
        n198 = call <vilib>:"Application Directory.vi"() -> ("Application Directory"=w875:path)
        n199 = local read "Diff list"() -> (w886:string[][])
        n200 = call "B07_Save_changed_PVs.vi"("For Test"=FALSE, "想要限制的筆數"=1000, "Directory Path"=w875, "紀錄起始時間  門檻"=w876, "diff_Value 2"=w886) -> ()  [unwired: 5 in, 2 out]
      }
      event "Save Button": Value Change {
        n201 = event-data() -> ()  [unwired: 1 in, 1 out]
        n202 = call <vilib>:"Beep.vi"("use system alert? (T)"=FALSE, "duration (msec)"=u32 40, "frequency (Hz)"=u32 1700) -> ()  [unwired: 9 in]
        n203 = Get Date/Time In Seconds() -> (seconds since 1Jan1904=w895:timestamp)
        n204 = Format Date/Time String(time format string (%c)="%Y", seconds (now)=w895, UTC format=FALSE) -> (date/time string=w914:string)
        n205 = Format Date/Time String(time format string (%c)="%d", seconds (now)=w895, UTC format=FALSE) -> (date/time string=w923:string)
        n206 = call "to_be_2_string.vi"("string 2"=w923) -> ("substring 2"=w924:string)  [unwired: 10 in]
        n207 = Format Date/Time String(time format string (%c)="%m", seconds (now)=w895, UTC format=FALSE) -> (date/time string=w918:string)
        n208 = Format Date/Time String(time format string (%c)="%Y%m%d%H%M%S", seconds (now)=w895) -> (date/time string=w902:string)  [unwired: 1 in]
        n209 = Concatenate Strings("D" ("磁碟位置"), ":\\LOG運轉紀錄\\", w914, "\\", w918, "\\", w924) -> (w907:string)
        n210 = String To Path(string=w907) -> (path=w910:path)
        n211 = call <vilib>:"Check if File or Folder Exists.vi"("path"=w910) -> ("error out"=w908:errorcluster, "file or folder exists?"=w922:bool, "dup path"=w909:path)  [unwired: 8 in]
        n212 = invoke on="Cluster" class="Clust (strict)" method="Get Image"() -> ("image data"=w893:T4)  [unwired: 6 in, 5 out]
        n213 = case shown="False" w922 {
          tunnel: w909 -> [w928 w930]
          tunnel: w908 -> [w927 w929]
          tunnel: [w926 w930] -> w894
          tunnel: [w925 w929] -> _
          frame False {
            n214 = Create Folder(path (use dialog)=w928, error in=w927) -> (created path=w926:path, error out=w925:errorcluster)  [unwired: 1 in, 1 out]
          }
          frame True {
          }
        }
        n215 = Path To String(path=w894) -> (string=w906:string)
        n216 = Concatenate Strings(w906, "\\" ("string"), w902) -> (w896:string)
        n217 = Concatenate Strings(w896, ".jpg" ("file format")) -> (w897:string)
        n218 = String To Path(string=w897) -> (path=w901:path)
        n219 = call <vilib>:"Write JPEG File.vi"("quality (80)"=100, "image data"=w893, "path to JPEG file"=w901) -> ("error out"=→"error out 3":errorcluster)  [unwired: 7 in, 1 out]
      }
    }
    n220 = call-poly <userlib>:"CaLabGet.vi"("PV Names"=string[] ["FE-DI-XBPM-051:signals:sa.X", "FE-DI-XBPM-051:signals:sa.Y", "FE-DI-XBPM-091:SA:SA_X_MONITOR", "FE-DI-XBPM-091:SA:SA_Y_MONITOR", "FE-DI-XBPM-211:SA:SA_X_MONITOR", "FE-DI-XBPM-211:SA:SA_Y_MONITOR", "FE-DI-XBPM-231:SA:SA_X_MONITOR", "FE-DI-XBPM-231:SA:SA_Y_MONITOR", "FE-DI-XBPM-251:SA:SA_X_MONITOR", "FE-DI-XBPM-251:SA:SA_Y_MONITOR", "FE-DI-XBPM-411:SA:SA_X_MONITOR", "FE-DI-XBPM-411:SA:SA_Y_MONITOR", "FE-DI-XBPM-451:SA:SA_X_MONITOR", "FE-DI-XBPM-451:SA:SA_Y_MONITOR", "FE-DI-XBPM-052:signals:sa.X", "FE-DI-XBPM-052:signals:sa.Y", "FE-DI-XBPM-092:SA:SA_X_MONITOR", "FE-DI-XBPM-092:SA:SA_Y_MONITOR", "FE-DI-XBPM-212:SA:SA_X_MONITOR", "FE-DI-XBPM-212:SA:SA_Y_MONITOR", "FE-DI-XBPM-232:SA:SA_X_MONITOR", "FE-DI-XBPM-232:SA:SA_Y_MONITOR", "FE-DI-XBPM-252:SA:SA_X_MONITOR", "FE-DI-XBPM-252:SA:SA_Y_MONITOR", "FE-DI-XBPM-412:SA:SA_X_MONITOR", "FE-DI-XBPM-412:SA:SA_Y_MONITOR", "FE-DI-XBPM-452:SA:SA_X_MONITOR", "FE-DI-XBPM-452:SA:SA_Y_MONITOR"] ("appended array")) -> ("1rst Value (number)"=w346:dbl[])  [unwired: 8 in, 6 out]
    n221 = Multiply(x=w346, y=0.001) -> (x*y=w345:dbl[])
    "Value Array (number) 7" <- w345
    n222 = disable-structure shown="Disabled" {
      frame Disabled {
        n223 = To Long Integer() -> (32bit integer=w975:i32)  [unwired: 1 in]
        n224 = case shown="1" w975 {
          tunnel: ["Decay" "Top-Up"] -> _
          frame 0, Default {
          }
          frame 1 {
          }
        }
      }
      frame Enabled {
      }
    }
    n225 = Index Array(array=w345, index #1=0 ("index"), index #2=1 ("index"), index #3=2 ("index"), index #4=3 ("index"), index #5=4 ("index"), index #6=5 ("index"), index #7=6 ("index"), index #8=7 ("index"), index #9=8 ("index"), index #10=9 ("index"), index #11=10 ("index"), index #12=11 ("index"), index #13=12 ("index"), index #14=13 ("index"), index #15=14 ("index"), index #16=15 ("index"), index #17=16 ("index"), index #18=17 ("index"), index #19=18 ("index"), index #20=19 ("index"), index #21=20 ("index"), index #22=21 ("index"), index #23=22 ("index"), index #24=23 ("index"), index #25=24 ("index"), index #26=25 ("index"), index #27=26 ("index"), index #28=27 ("index")) -> (element #1=w262:dbl, element #2=w255:dbl, element #3=w261:dbl, element #4=w254:dbl, element #5=w260:dbl, element #6=w253:dbl, element #7=w259:dbl, element #8=w252:dbl, element #9=w258:dbl, element #10=w251:dbl, element #11=w257:dbl, element #12=w250:dbl, element #13=w256:dbl, element #14=w249:dbl, element #15=w154:dbl, element #16=w153:dbl, element #17=w152:dbl, element #18=w151:dbl, element #19=w142:dbl, element #20=w141:dbl, element #21=w136:dbl, element #22=w135:dbl, element #23=w134:dbl, element #24=w133:dbl, element #25=w102:dbl, element #26=w101:dbl, element #27=w100:dbl, element #28=w99:dbl)
    n226 = call-poly <userlib>:"CaLabGet.vi"("PV Names"=string[] ["LI-ES-CPS-01:PULSEMODE", "LI-ES-BPS-01:SETU:GRID", "LI-ES-BPS-01:SETU:MBM", "LI-ES-BPS-01:SETU:SBM", "LI-RF-HVP-31:SET:U", "CPCITM-TI-EVRTG:Pulse6DelaySet", "CPCITM-TI-EVRTG:Pulse7DelaySet", "CPCITM-TI-EVRTG:Pulse6WidthSet", "CPCITM-TI-EVRTG:Pulse7WidthSet", "CPCITM-TI-EVRTG:GTX6CtrlGTXPHSet", "CPCITM-TI-EVRTG:GTX7CtrlGTXPHSet", "CPCITM-TI-EVRTG:GTX6DlySet", "CPCITM-TI-EVRTG:GTX7DlySet"]) -> ("1rst Value (string)"=w408:string[], "1rst Value (number)"=w459:dbl[])  [unwired: 8 in, 5 out]
    "Value Array (number) 3" <- w459
    n227 = call-poly <userlib>:"CaLabGet.vi"("PV Names"=string[] ["BR-PS-INJ-SE:setHV", "BR-PS-INJ-KI:setHV", "BR-PS-EXT-K1:setHV", "BR-PS-EXT-K2:setHV", "BR-PS-EXT-SE1:setHV", "BR-PS-EXT-SE2:setHV", "SR-PS-INJ-SE1:setHV", "SR-PS-INJ-SE2:setHV", "SR-PS-INJ-K1:setHV", "SR-PS-INJ-K2:setHV", "SR-PS-INJ-K3:setHV", "SR-PS-INJ-K4:setHV"]) -> ("1rst Value (number)"=w461:dbl[])  [unwired: 8 in, 6 out]
    n228 = call-poly <userlib>:"CaLabGet.vi"("PV Names"=string[] ["SR-RF-MSG:setFreq", "SR-RF2-LLRF:local", "SR-RF2-LLRF:getOperationMode", "SR-RF2-LLRF:getGapVoltage", "SR-RF2-LLRF:setGapVoltage", "SR-RF2-LLRF:setStationPhase", "SR-RF3-LLRF:local", "SR-RF3-LLRF:getOperationMode", "SR-RF3-LLRF:getGapVoltage", "SR-RF3-LLRF:setGapVoltage", "SR-RF3-LLRF:setStationPhase"]) -> ("1rst Value (number)"=w434:dbl[])  [unwired: 8 in, 6 out]
    n229 = call-poly <userlib>:"CaLabGet.vi"("PV Names"=string[] ["SR-DI-FP:CurrentBuffer"]) -> ("Value Array (number)"=w416:dbl[][])  [unwired: 8 in, 6 out]
    n230 = call-poly <userlib>:"CaLabGet.vi"("PV Names"=string[] ["TI-INJ-PROC:TopupHiLowStart", "SR-DI-DCCT:BeamCurrent", "SR-DI-DCCT:BeamLifetime", "SR-DI-XPC-40:SigmaX", "SR-DI-XPC-40:SigmaY", "SR-DI-TUNE:nux", "SR-DI-TUNE:nuy", "IGPF:TPSX:SRAM:VEC:PEAKFREQ2", "IGPF:TPSY:SRAM:VEC:PEAKFREQ2", "TI-INJ-PROC:setBucketAddressStart", "TI-INJ-PROC:setBucketAddressLast", "TI-INJ-PROC:setBucketAddressStep"]) -> ("1rst Value (number)"=w495:dbl[])  [unwired: 8 in, 6 out]
    n231 = call-poly <userlib>:"CaLabGet.vi"("PV Names"=string[] ["LI:restoreFilename", "LTB:restoreFilename", "BR:restoreFilename", "BTS:restoreFilename", "SR:restoreFilename"]) -> ("1rst Value (string)"=w418:string[])  [unwired: 8 in, 6 out]
    n232 = Index Array(array=w408, index=0) -> (element=w406:string)
    n233 = Index Array(array=w459, index #1=0 ("index"), index #2=1 ("index"), index #3=2 ("index"), index #4=3 ("index"), index #5=4 ("index"), index #6=5 ("index"), index #7=6 ("index"), index #8=7 ("index"), index #9=8 ("index"), index #10=9 ("index"), index #11=10 ("index"), index #12=11 ("index"), index #13=12 ("index")) -> (element #2=w295:dbl, element #3=w410:dbl, element #4=w409:dbl, element #5=w293:dbl, element #8=w405:dbl, element #9=w404:dbl, element #10=w403:dbl, element #11=w402:dbl, element #12=w401:dbl, element #13=w400:dbl)  [unwired: 3 out]
    "MBM volt.(S)" <- w410
    "SBM volt.(S)" <- w409
    n234 = Index Array(array=w461, index #1=0 ("index"), index #2=1 ("index"), index #3=2 ("index"), index #4=3 ("index"), index #5=4 ("index"), index #6=5 ("index"), index #7=6 ("index"), index #8=7 ("index"), index #9=8 ("index"), index #10=9 ("index"), index #11=10 ("index"), index #12=11 ("index")) -> (element #1=w308:dbl, element #2=w307:dbl, element #3=w306:dbl, element #4=w305:dbl, element #5=w304:dbl, element #6=w303:dbl, element #7=w302:dbl, element #8=w301:dbl, element #9=w300:dbl, element #10=w299:dbl, element #11=w298:dbl, element #12=w297:dbl)
    n235 = Index Array(array=w434, index #1=0 ("index"), index #2=1 ("index"), index #3=2 ("index"), index #4=3 ("index"), index #5=4 ("index"), index #6=5 ("index"), index #7=6 ("index"), index #8=7 ("index"), index #9=8 ("index"), index #10=9 ("index"), index #11=10 ("index")) -> (element #1=w287:dbl, element #2=w431:dbl, element #3=w429:dbl, element #5=w210:dbl, element #6=w211:dbl, element #7=w426:dbl, element #8=w425:dbl, element #10=w283:dbl, element #11=w284:dbl)  [unwired: 2 out]
    n236 = Index Array(array=w416, index (row)=0 ("index")) -> (element=w277:dbl[])  [unwired: 1 in]
    n237 = Index Array(array=w495, index #1=0 ("index"), index #2=1 ("index"), index #3=2 ("index"), index #4=3 ("index"), index #5=4 ("index"), index #6=5 ("index"), index #7=6 ("index"), index #8=7 ("index"), index #9=8 ("index"), index #10=9 ("index"), index #11=10 ("index"), index #12=11 ("index")) -> (element #1=w493:dbl, element #2=w317:dbl, element #3=w316:dbl, element #4=w481:dbl, element #5=w479:dbl, element #6=w478:dbl, element #7=w477:dbl, element #8=w476:dbl, element #9=w474:dbl, element #10=w311:dbl, element #11=w310:dbl, element #12=w309:dbl)
    n238 = call-poly <userlib>:"CaLabGet.vi"("PV Names"=w184) -> ("1rst Value (number)"=w186:dbl[])  [unwired: 8 in, 6 out]
    n239 = Index Array(array=w418, index #1=0 ("index"), index #2=1 ("index"), index #3=2 ("index"), index #4=3 ("index"), index #5=4 ("index")) -> (element #1=w279:string, element #2=w278:string, element #3=w282:string, element #4=w281:string, element #5=w280:string)
    n240 = call-poly <userlib>:"CaLabGet.vi"("PV Names"=w379) -> ("1rst Value (string)"=w387:string[])  [unwired: 8 in, 6 out]
    n241 = To Byte Integer(number=w186) -> (8bit integer=w185:i8[])
    n242 = for {
      tunnel: w185 -> [w934] mode=indexing
      tunnel: [w931] -> w162 mode=indexing
      n243 = Number To Boolean Array(number=w934) -> (Boolean array=w933:bool[])
      n244 = Index Array(array=w933, index=0) -> (element=w931:bool)
    }
    n245 = for {
      tunnel: w387 -> [w944] mode=indexing
      tunnel: [w943] -> w388 mode=indexing
      n246 = case shown="\"Enable\"" w944 {
        tunnel: [FALSE TRUE] -> w943
        frame "Disable", Default {
        }
        frame "Enable" {
        }
      }
    }
    n247 = call-poly <userlib>:"CaLabGet.vi"("PV Names"=w398) -> ("1rst Value (string)"=w390:string[])  [unwired: 8 in, 6 out]
    n248 = call-poly <userlib>:"CaLabGet.vi"("PV Names"=string[] ["SR-ID-IU22-05:getGap", "SR-ID-IU22A-09:getGap", "SR-ID-IU22B-09:getGap", "SR-ID-IUT22-21:getGap", "SR-ID-IU22-23:getGap", "SR-ID-IU22A-25:getGap", "SR-ID-IU22B-25:getGap", "SR-ID-EPU48A-41:getGap", "SR-ID-EPU48A-41:getPhase", "SR-ID-EPU48B-41:getGap", "SR-ID-EPU48B-41:getPhase", "SR-ID-EPU46-45:getGap", "SR-ID-EPU46-45:getPhase", "SR-ID-IUT22-21:getGapTaper", "SR-ID-EPU48PS-41:getGap"]) -> ("1rst Value (number)"=w378:dbl[])  [unwired: 8 in, 6 out]
    "Value Array (number) 6" <- w378
    n249 = for {
      tunnel: w390 -> [w948] mode=indexing
      tunnel: [w947] -> w389 mode=indexing
      n250 = case shown="\"enable\"" w948 {
        tunnel: [FALSE TRUE] -> w947
        frame "disable", Default {
        }
        frame "enable" {
        }
      }
    }
    n251 = call-poly <userlib>:"CaLabGet.vi"("PV Names"=string[] ["SR-ID-IU22-05:gapMotorOff", "SR-ID-IU22A-09:gapMotorOff", "SR-ID-IU22B-09:gapMotorOff", "SR-ID-IUT22-21:gapMotorOff", "SR-ID-IU22-23:gapMotorOff", "SR-ID-IU22A-25:gapMotorOff", "SR-ID-IU22B-25:gapMotorOff", "SR-ID-EPU48A-41:gapMotorOff", "SR-ID-EPU48B-41:gapMotorOff", "SR-ID-EPU46-45:gapMotorOff", "SR-ID-EPU48A-41:phaseMotorOff", "SR-ID-EPU48B-41:phaseMotorOff", "SR-ID-EPU46-45:phaseMotorOff"]) -> ("1rst Value (string)"=w330:string[])  [unwired: 8 in, 6 out]
    n252 = To Long Integer(number=w429) -> (32bit integer=w430:i32)
    n253 = To Long Integer(number=w431) -> (32bit integer=w432:i32)
    n254 = To Long Integer(number=w425) -> (32bit integer=w428:i32)
    n255 = To Long Integer(number=w426) -> (32bit integer=w427:i32)
    n256 = Index Array(array=w378, index #1=0 ("index"), index #2=1 ("index"), index #3=2 ("index"), index #4=3 ("index"), index #5=4 ("index"), index #6=5 ("index"), index #7=6 ("index"), index #8=7 ("index"), index #9=8 ("index"), index #10=9 ("index"), index #11=10 ("index"), index #12=11 ("index"), index #13=12 ("index"), index #14=13 ("index"), index #15=14 ("index")) -> (element #1=w276:dbl, element #2=w275:dbl, element #3=w274:dbl, element #4=w273:dbl, element #5=w272:dbl, element #6=w271:dbl, element #7=w270:dbl, element #8=w269:dbl, element #9=w268:dbl, element #10=w267:dbl, element #11=w266:dbl, element #12=w265:dbl, element #13=w264:dbl, element #14=w209:dbl, element #15=w263:dbl)
    n257 = for {
      tunnel: w330 -> [w940] mode=indexing
      tunnel: [w939] -> w329 mode=indexing
      n258 = case shown="\"1\", Default" w940 {
        tunnel: [FALSE TRUE] -> w939
        frame "1", Default {
        }
        frame "0" {
        }
      }
    }
    n259 = Index Array(array=w162, index #1=0 ("index"), index #2=1 ("index"), index #3=2 ("index"), index #4=3 ("index"), index #5=4 ("index"), index #6=5 ("index"), index #7=6 ("index"), index #8=7 ("index"), index #9=8 ("index"), index #10=9 ("index"), index #11=10 ("index"), index #12=11 ("index"), index #13=12 ("index"), index #14=13 ("index"), index #15=14 ("index"), index #16=15 ("index"), index #17=16 ("index"), index #18=17 ("index"), index #19=18 ("index"), index #20=19 ("index"), index #21=20 ("index")) -> (element #1=w159:bool, element #2=w158:bool, element #3=w157:bool, element #4=w146:bool, element #5=w145:bool, element #6=w144:bool, element #7=w139:bool, element #8=w138:bool, element #9=w137:bool, element #10=w128:bool, element #11=w127:bool, element #12=w126:bool, element #13=w121:bool, element #14=w120:bool, element #15=w119:bool, element #16=w118:bool, element #17=w117:bool, element #18=w116:bool, element #19=w115:bool, element #20=w114:bool, element #21=w113:bool)
    n260 = case shown="1" w432 {
      tunnel: [FALSE TRUE] -> w289
      frame 0, Default {
      }
      frame 1 {
      }
    }
    n261 = case shown="1" w427 {
      tunnel: [FALSE TRUE] -> w286
      frame 0, Default {
      }
      frame 1 {
      }
    }
    n262 = case shown="0" w430 {
      tunnel: [TRUE FALSE] -> w288
      frame 0 {
      }
      frame 1, Default {
      }
    }
    n263 = case shown="0" w428 {
      tunnel: [TRUE FALSE] -> w285
      frame 0 {
      }
      frame 1, Default {
      }
    }
    n264 = To Long Integer(number=w493) -> (32bit integer=w496:i32)
    n265 = Negate(x=w209) -> (-x=w208:dbl)
    n266 = case shown="1" w496 {
      tunnel: ["Decay" "Top-Up"] -> w318
      frame 0, Default {
      }
      frame 1 {
      }
    }
    n267 = Index Array(array=w388, index #1=0 ("index"), index #2=1 ("index"), index #3=2 ("index"), index #4=3 ("index"), index #5=4 ("index"), index #6=5 ("index"), index #7=6 ("index")) -> (element #1=w160:bool, element #2=w156:bool, element #3=w140:bool, element #4=w123:bool, element #5=w122:bool, element #6=w104:bool, element #7=w103:bool)
    n268 = case shown="\"MBM\", Default" w406 {
      tunnel: ["MBM" "SBM"] -> w296
      tunnel: w410 -> [w954 _]
      tunnel: [w954 w959] -> w294
      tunnel: w409 -> [_ w959]
      tunnel: w405 -> [_ w958]
      tunnel: w404 -> [w953 _]
      tunnel: [w953 w958] -> w292
      tunnel: w403 -> [_ w957]
      tunnel: w402 -> [w952 _]
      tunnel: [w952 w957] -> w291
      tunnel: w401 -> [_ w956]
      tunnel: w400 -> [w951 _]
      tunnel: [w951 w956] -> w290
      frame "MBM", Default {
      }
      frame "SBM" {
      }
    }
    n269 = Multiply(x=w481, y=w480) -> (x*y=w315:dbl)
    n270 = Divide(x=w476, y=w475) -> (x/y=w313:dbl)
    n271 = Multiply(x=w479, y=w480) -> (x*y=w314:dbl)
    n272 = Divide(x=w474, y=w475) -> (x/y=w312:dbl)
    n273 = Index Array(array=w389, index #1=0 ("index"), index #2=1 ("index"), index #3=2 ("index"), index #4=3 ("index"), index #5=4 ("index"), index #6=5 ("index"), index #7=6 ("index")) -> (element #1=w161:bool, element #2=w155:bool, element #3=w143:bool, element #4=w125:bool, element #5=w124:bool, element #6=w106:bool, element #7=w105:bool)
    n274 = call "FE_PAB_OpenState.vi"("FE"=w161, "XBPMX 2"=w154, "XBPMY 2"=w153, "Hutch"=w160, "PAB"=w159, "MGV"=w158, "FCV"=w157) -> ("XBPMX 2"=w150:string, "XBPMY 2"=w149:string)  [unwired: 7 in]
    n275 = call "FE_PAB_OpenState.vi"("FE"=w155, "XBPMX 2"=w152, "XBPMY 2"=w151, "Hutch"=w156, "PAB"=w146, "MGV"=w145, "FCV"=w144) -> ("XBPMX 2"=w148:string, "XBPMY 2"=w147:string)  [unwired: 7 in]
    n276 = call-poly <userlib>:"CaLabGet.vi"("PV Name"="TI-INJ-PROC:getTrig-SR-KICKER") -> ("1rst Value (string)"=w413:string)  [unwired: 8 in, 6 out]
    n277 = Index Array(array=w329, index #1=0 ("index"), index #2=1 ("index"), index #3=2 ("index"), index #4=3 ("index"), index #5=4 ("index"), index #6=5 ("index"), index #7=6 ("index"), index #8=7 ("index"), index #9=8 ("index"), index #10=9 ("index"), index #11=10 ("index"), index #12=11 ("index"), index #13=12 ("index")) -> (element #1=w248:bool, element #2=w247:bool, element #3=w246:bool, element #4=w245:bool, element #5=w244:bool, element #6=w243:bool, element #7=w242:bool, element #8=w241:bool, element #9=w240:bool, element #10=w239:bool, element #11=w238:bool, element #12=w237:bool, element #13=w236:bool)
    n278 = call-poly <userlib>:"CaLabGet.vi"("PV Names"=w320) -> ("1rst Value (number)"=w322:dbl[])  [unwired: 8 in, 6 out]
    n279 = call-poly <userlib>:"CaLabGet.vi"("PV Names"=w321) -> ("1rst Value (number)"=w324:dbl[])  [unwired: 8 in, 6 out]
    n280 = call "FE_PAB_OpenState.vi"("FE"=w143, "XBPMX 2"=w142, "XBPMY 2"=w141, "Hutch"=w140, "PAB"=w139, "MGV"=w138, "FCV"=w137) -> ("XBPMX 2"=w132:string, "XBPMY 2"=w131:string)  [unwired: 7 in]
    n281 = call-poly <userlib>:"CaLabGet.vi"("PV Names"=string[] ["SR-DI-FOFB-H:getStatus", "SR-DI-FOFB-V:getStatus", "IGPF:TPSX:FBCTRL", "IGPF:TPSY:FBCTRL", "TPS-SR-022:bpm3:ilk:enabled", "SR-DI-ANGLE-ILK:StatusX", "SR-DI-ANGLE-ILK:StatusY", "SR-DI-RF-FB:getStatus"]) -> ("1rst Value (string)"=w224:string[], "1rst Value (number)"=w225:dbl[])  [unwired: 8 in, 5 out]
    n282 = call "FE_PAB_OpenState.vi"("FE"=w125, "XBPMX 2"=w136, "XBPMY 2"=w135, "Hutch"=w123, "PAB"=w128, "MGV"=w127, "FCV"=w126) -> ("XBPMX 2"=w130:string, "XBPMY 2"=w129:string)  [unwired: 7 in]
    n283 = Multiply(x=w322, y=w323) -> (x*y=w202:dbl[])
    n284 = To Byte Integer(number=w225) -> (8bit integer=w221:i8[])
    n285 = Multiply(x=w324, y=w323) -> (x*y=w203:dbl[])
    n286 = for {
      tunnel: w221 -> [w936] mode=indexing
      tunnel: [w935] -> w231 mode=indexing
      n287 = case shown="1" w936 {
        tunnel: [TRUE FALSE] -> w935
        frame 1 {
        }
        frame 0, Default {
        }
      }
    }
    n288 = Array Max & Min(array=w202) -> ()  [unwired: 4 out]
    n289 = Array Max & Min(array=w203) -> ()  [unwired: 4 out]
    n290 = call "FE_PAB_OpenState.vi"("FE"=w124, "XBPMX 2"=w134, "XBPMY 2"=w133, "Hutch"=w122, "PAB"=w121, "MGV"=w120, "FCV"=w119) -> ("XBPMX 2"=w112:string, "XBPMY 2"=w111:string)  [unwired: 7 in]
    n291 = Index Array(array=w224, index #1=0 ("index"), index #2=1 ("index"), index #3=7 ("index")) -> (element #1=w219:string, element #2=w218:string, element #3=w69:string)
    n292 = call "FE_PAB_OpenState.vi"("FE"=w106, "XBPMX 2"=w102, "XBPMY 2"=w101, "Hutch"=w104, "PAB"=w118, "MGV"=w117, "FCV"=w116) -> ("XBPMX 2"=w110:string, "XBPMY 2"=w109:string)  [unwired: 7 in]
    n293 = call "FE_PAB_OpenState.vi"("FE"=w105, "XBPMX 2"=w100, "XBPMY 2"=w99, "Hutch"=w103, "PAB"=w115, "MGV"=w114, "FCV"=w113) -> ("XBPMX 2"=w108:string, "XBPMY 2"=w107:string)  [unwired: 7 in]
    n294 = Bundle("Array of X axis  平均分配至各段"=w67, w202) -> (w64:cluster{"Array of X axis  平均分配至各段":dbl[], dbl[]})  [unwired: 1 in]
    n295 = Bundle("Array of X axis  平均分配至各段"=w67, w203) -> (w63:cluster{"Array of X axis  平均分配至各段":dbl[], dbl[]})  [unwired: 1 in]
    n296 = Index Array(array=w231, index #1=2 ("index"), index #2=3 ("index"), index #3=4 ("index"), index #4=5 ("index"), index #5=6 ("index")) -> (element #1=w217:bool, element #2=w216:bool, element #3=w215:bool)  [unwired: 2 out]
    n297 = Equal?(x="1" ("1rst Value (string)"), y=w413) -> (x = y?=w411:bool)
    "x = y?" <- w411
    n298 = case shown="True" TRUE {
      tunnel: w74 -> [_ w498]
      frame False {
      }
      frame True {
        n299 = Quit LabVIEW(quit? (T)=w498) -> ()
      }
    }
    n300 = case shown="False" w411 {
      tunnel: w478 -> [_ w964]
      tunnel: w477 -> [_ w963]
      tunnel: [w962 w964] -> w207
      tunnel: [w961 w963] -> w206
      tunnel: w205 -> [w962 _]
      tunnel: w204 -> [w961 _]
      frame False {
      }
      frame True {
        n301 = local read "NOW date"() -> (→"date kickeron":string)
        n302 = local read "NOW time"() -> (→"time kickeron":string)
      }
    }
    n303 = Wait Until Next ms Multiple(millisecond multiple=u32 1000) -> ()  [unwired: 1 out]
    n304 = local read "date kickeron"() -> (w213:string)
    n305 = local read "time kickeron"() -> (w212:string)
    n306 = Get Date/Time In Seconds() -> (seconds since 1Jan1904=w326:timestamp)
    n307 = call-poly <userlib>:"CaLabGet.vi"("PV Names"=w98) -> ("1rst Value (string)"=w87:string[])  [unwired: 8 in, 6 out]
    n308 = Format Date/Time String(time format string (%c)="%Y/%m/%d", seconds (now)=w326) -> (date/time string=→"NOW date":string)  [unwired: 1 in]
    n309 = Format Date/Time String(time format string (%c)="%Y/%m/%d", seconds (now)=w326) -> (date/time string=w235:string)  [unwired: 1 in]
    n310 = Format Date/Time String(time format string (%c)="%H:%M:%S", seconds (now)=w326) -> (date/time string=w234:string)  [unwired: 1 in]
    "NOW time" <- w234
    n311 = Index Array(array=w87, index #1=0 ("index"), index #2=1 ("index"), index #3=2 ("index"), index #4=3 ("index"), index #5=4 ("index"), index #6=5 ("index"), index #7=6 ("index"), index #8=7 ("index"), index #9=8 ("index"), index #10=9 ("index")) -> (element #1=w86:string, element #2=w85:string, element #3=w84:string, element #4=w83:string, element #5=w82:string, element #6=w81:string, element #7=w80:string, element #8=w79:string, element #9=w78:string, element #10=w77:string)
    n312 = Bundle By Name(cluster=T1 {"SR Fill Pattern"=array[864 elements], "Beam Current(mA"=321.397805, "Beam Lifetime(min)"=353.6260562320138, "Beamsize X(um)"=63.067730523299595, "Beamsize Y(um)"=38.02823648772029, "Tune X(from BPM)"=0.1487279843444227, "Tune Y(from BPM)"=0.2309197651663405, "Mode"="Top-Up", "NuX(from BBF) "=0.1502078828062249, "NuY(from BBF)"=0.22496346361412184, "IU22-23gap(R)"=7.0, "IU22-05gap(R)"=7.399, "IU22-05M"=TRUE, "IU22A-09gap(R)"=8.05, "IU22A-09M"=TRUE, "IU22B-09gap(R)"=40.001, "IU22B-09M"=FALSE, "IUT22-21gap(R)"=7.0, "IUT22-21M"=TRUE, "IU22-23M"=TRUE, "IU22A-25gap(R)"=7.0, "IU22A-25M"=TRUE, "IU22B-25gap(R)"=40.0, "IU22B-25M"=FALSE, "EPU48A-41gap(R)"=65.0006, "EPU48A-41gM"=FALSE, "EPU48B-41gap(R)"=27.44995, "EPU48B-41gM"=TRUE, "EPU46-45gap(R)"=44.99850000000001, "EPU46-45gM"=FALSE, "EPU48A-41phase(R)"=0.00055, "EPU48B-41phase(R)"=0.0, "EPU46-45phase(R)"=5e-05, "Grid volt.(V)(S)"=33.0, "Gun mode"="MBM", "Mod.3 HV(kV)(S)"=35.37999999999996, "SR"="SR_DMB_2017_1024_0300LOCO.data", "BR"="Booster_2017_1023_0900.data", "Linac"="Linac_2017_0413_1015.data", "LTB"="LTB_JT_2017_0828_1050.data", "BTS"="BTS_2017_1023_0900.data", "RF2 remote"=TRUE, "RF2 OP mode"=TRUE, "RF2 phase.(S)"=-42.0, "RF Freq.(s)"=499655372.0590207, "RF2 gap volt.(S)"=1600.0, "RF3 remote"=TRUE, "RF3 OP mode"=TRUE, "RF3 phase.(S)"=1.1999999999999995, "RF3 gap volt.(S)"=1600.0, "BBF V"=TRUE, "BBF H"=TRUE, "BR ext. kicker1(kV)"=17.666, "BR ext. kicker2(kV)"=17.666, "BR ext. sep.1(V)"=322.14, "BR ext. sep.2(V)"=441.1, "BR inj. sep.(V)"=104.95, "BR inj. kicker(kV)"=13.449999999999969, "SR kicker4(kV)"=7.945, "SR kicker3(kV)"=8.02, "SR kicker2(kV)"=8.142, "SR kicker1(kV)"=8.1, "SR inj. sep.2(V)"=397.2, "SR inj. sep.1(V)"=398.04, "Bucket Start"=100.0, "Bucket Last"=450.0, "Bucket Step"=10.0, "Orbit ILK(P)"=TRUE, "IU22-05 Hutch Enable"=TRUE, "IU22A-09M Hutch Enable"=TRUE, "IUT22-21M Hutch Enable"=TRUE, "IU22-23M Hutch Enable"=TRUE, "IU22A-25M Hutch Enable"=TRUE, "EPU48A-41M Hutch Enable"=TRUE, "EPU46-45M Hutch Enable"=FALSE, "EPU46-45 FE Enable"=TRUE, "EPU48A-41 FE Enable"=TRUE, "IU22A-25 FE Enable"=TRUE, "IU22-23 FE Enable"=TRUE, "IUT22-21 FE Enable"=TRUE, "IU22A-09 FE Enable"=TRUE, "IU22-05 FE Enable"=TRUE, "EPU48A-41pM"=FALSE, "EPU48B-41pM"=TRUE, "EPU46-45pM"=FALSE, "Gun volt.(V)(S)"=23.5, "Width count"=75.0, "2ns step"=2.0, "10ps delay"=150.0, "phase shifter"=130.0015, "Taper"=1.0899999999999999, "05XBPMX 1"=18.217, "09XBPMX 1"=-35.273, "21XBPMX 1"=-37.205, "23XBPMX 1"=-39.666000000000004, "25XBPMX 1"=-41.598, "41XBPMX 1"=-514.719, "45XBPMX 1"=-13.727, "05XBPMY 1"=52.193, "09XBPMY 1"=27.633, "21XBPMY 1"=-4.559, "23XBPMY 1"=19.132, "25XBPMY 1"=-4.634, "41XBPMY 1"=310.067, "45XBPMY 1"=1.909, "FOFB H"="On", "FOFB V"="On", "time string"="15:09:56", "date"="2017/10/28", "date (last kicker ON)"="2017/10/28", "time string (last kicker ON)"="15:09:26", "Radio Buttons 2"=enum."absolute", "09XBPMX 2"="24.03", "09XBPMY 2"="-18.69", "05XBPMY 2"="-460.42", "05XBPMX 2"="-403.04", "21XBPMY 2"="-134.80", "21XBPMX 2"="-32.13", "23XBPMY 2"="233.63", "23XBPMX 2"="10.79", "25XBPMY 2"="5173.11", "25XBPMX 2"="2153.87", "41XBPMY 2"=" closed", "41XBPMX 2"=" PAB ", "45XBPMX 2"=" Hutch ", "45XBPMY 2"=" closed", "05 mode"="Follow", "09A mode"="Follow", "09B mode"="Follow", "21 mode"="Follow", "23 mode"="Follow", "25A mode"="Follow", "25B mode"="Follow", "41A mode"="Follow", "41B mode"="Follow", "46 mode"="Follow", "BeamCurrent History"={"BPM NO.  1_172"=array[4318 elements], array[4318 elements]}, "SR Beam Current in            hours"=12.0, "RF FB"="On", "BPMX Graph 2"={"Array of X axis  平均分配至各段"=[1.0, 1.1666666666666667, 1.3333333333333333, 1.5, 1.6666666666666665, 1.8333333333333333, 2.0, 2.142857142857143, 2.2857142857142856, 2.4285714285714284, 2.571428571428571, 2.7142857142857144, 2.857142857142857, 3.0, 3.142857142857143, 3.2857142857142856, 3.4285714285714284, 3.571428571428571, 3.7142857142857144, 3.857142857142857, 4.0, 4.125, 4.25, 4.375, 4.5, 4.625, 4.75, 4.875, 5.0, 5.125, 5.25, 5.375, 5.5, 5.625, 5.75, 5.875, 6.0, 6.142857142857143, 6.285714285714286, 6.428571428571429, 6.571428571428571, 6.714285714285714, 6.857142857142857, 7.0, 7.142857142857143, 7.285714285714286, 7.428571428571429, 7.571428571428571, 7.714285714285714, 7.857142857142857, 8.0, 8.142857142857142, 8.285714285714286, 8.428571428571429, 8.571428571428571, 8.714285714285714, 8.857142857142858, 9.0, 9.142857142857142, 9.285714285714286, 9.428571428571429, 9.571428571428571, 9.714285714285714, 9.857142857142858, 10.0, 10.142857142857142, 10.285714285714286, 10.428571428571429, 10.571428571428571, 10.714285714285714, 10.857142857142858, 11.0, 11.142857142857142, 11.285714285714286, 11.428571428571429, 11.571428571428571, 11.714285714285714, 11.857142857142858, 12.0, 12.125, 12.25, 12.375, 12.5, 12.625, 12.75, 12.875, 13.0, 13.125, 13.25, 13.375, 13.5, 13.625, 13.75, 13.875, 14.0, 14.142857142857142, 14.285714285714286, 14.428571428571429, 14.571428571428571, 14.714285714285714, 14.857142857142858, 15.0, 15.142857142857142, 15.285714285714286, 15.428571428571429, 15.571428571428571, 15.714285714285714, 15.857142857142858, 16.0, 16.142857142857142, 16.285714285714285, 16.428571428571427, 16.571428571428573, 16.714285714285715, 16.857142857142858, 17.0, 17.142857142857142, 17.285714285714285, 17.428571428571427, 17.571428571428573, 17.714285714285715, 17.857142857142858, 18.0, 18.142857142857142, 18.285714285714285, 18.428571428571427, 18.571428571428573, 18.714285714285715, 18.857142857142858, 19.0, 19.142857142857142, 19.285714285714285, 19.428571428571427, 19.571428571428573, 19.714285714285715, 19.857142857142858, 20.0, 20.125, 20.25, 20.375, 20.5, 20.625, 20.75, 20.875, 21.0, 21.125, 21.25, 21.375, 21.5, 21.625, 21.75, 21.875, 22.0, 22.142857142857142, 22.285714285714285, 22.428571428571427, 22.571428571428573, 22.714285714285715, 22.857142857142858, 23.0, 23.142857142857142, 23.285714285714285, 23.428571428571427, 23.571428571428573, 23.714285714285715, 23.857142857142858, 24.0, 24.166666666666668, 24.333333333333332, 24.5, 24.666666666666668, 24.833333333333332], [-104.227, -27.392, -81.018, 31.28, 6.132000000000001, -135.87, 99.482, -88.327, -46.663000000000004, -164.852, 6.208, -84.886, 1.943, -8.764, 8.325, -133.845, -96.541, 25.052, 5.134, -100.18900000000001, 144.734, -9.466000000000001, 21.308, -54.732, 53.756, 191.299, 158.747, 222.874, -123.647, -26.238, 534.69, 573.208, -224.824, -6.72, 120.822, -75.292, 85.152, 50.89, -59.291000000000004, -202.874, -20.561, 130.56300000000002, -112.505, 76.172, 14.976, -35.12, -105.438, -16.586000000000002, 69.038, -141.012, 107.333, 144.232, -54.824, -193.089, 129.575, 58.372, -162.483, 153.757, 28.289, 9.403, -83.349, 84.846, 23.046, -31.029, 89.548, -47.595, 54.976, -68.162, 110.83800000000001, -118.546, -371.735, -19.905, -329.171, -248.937, -146.731, 118.799, -25.663, -98.276, 55.484, -122.214, 51.079, -55.6, 88.252, -0.417, -608.077, -139.565, -304.883, -214.90200000000002, 93.242, 44.795, -65.068, 37.347, -3.416, -169.766, 216.592, 50.29, -92.114, -131.881, -12.643, 66.816, -188.424, 148.784, -5.175, -71.23, -177.479, 41.446, -12.38, -184.66400000000002, 194.874, 52.247, -75.578, -80.254, -36.615, 105.784, -104.456, 110.113, 49.676, -67.27, -157.036, 29.876, 22.181, -105.571, 47.881, 11.346, -75.185, -79.621, 34.539, -24.888, -158.69, 177.365, 200.818, -165.714, -60.410000000000004, 20.396, -15.233, -111.031, 107.666, 26.375, 69.638, -40.93, 82.21300000000001, 54.462, 253.235, 378.57, -116.893, -304.883, 131.02700000000002, 2.457, -158.189, 94.82900000000001, 63.029, -82.897, 99.34400000000001, 65.763, -37.109, -102.32900000000001, 42.021, 66.714, -163.54, 160.316, -7.206, -51.043, -140.245, 34.113, 54.116, -147.479, 128.90800000000002, 58.346000000000004, -47.1, -184.366, 57.122, 67.505, -53.948, -2.9250000000000003]}, "BPMY Graph 2"={"Array of X axis  平均分配至各段"=[1.0, 1.1666666666666667, 1.3333333333333333, 1.5, 1.6666666666666665, 1.8333333333333333, 2.0, 2.142857142857143, 2.2857142857142856, 2.4285714285714284, 2.571428571428571, 2.7142857142857144, 2.857142857142857, 3.0, 3.142857142857143, 3.2857142857142856, 3.4285714285714284, 3.571428571428571, 3.7142857142857144, 3.857142857142857, 4.0, 4.125, 4.25, 4.375, 4.5, 4.625, 4.75, 4.875, 5.0, 5.125, 5.25, 5.375, 5.5, 5.625, 5.75, 5.875, 6.0, 6.142857142857143, 6.285714285714286, 6.428571428571429, 6.571428571428571, 6.714285714285714, 6.857142857142857, 7.0, 7.142857142857143, 7.285714285714286, 7.428571428571429, 7.571428571428571, 7.714285714285714, 7.857142857142857, 8.0, 8.142857142857142, 8.285714285714286, 8.428571428571429, 8.571428571428571, 8.714285714285714, 8.857142857142858, 9.0, 9.142857142857142, 9.285714285714286, 9.428571428571429, 9.571428571428571, 9.714285714285714, 9.857142857142858, 10.0, 10.142857142857142, 10.285714285714286, 10.428571428571429, 10.571428571428571, 10.714285714285714, 10.857142857142858, 11.0, 11.142857142857142, 11.285714285714286, 11.428571428571429, 11.571428571428571, 11.714285714285714, 11.857142857142858, 12.0, 12.125, 12.25, 12.375, 12.5, 12.625, 12.75, 12.875, 13.0, 13.125, 13.25, 13.375, 13.5, 13.625, 13.75, 13.875, 14.0, 14.142857142857142, 14.285714285714286, 14.428571428571429, 14.571428571428571, 14.714285714285714, 14.857142857142858, 15.0, 15.142857142857142, 15.285714285714286, 15.428571428571429, 15.571428571428571, 15.714285714285714, 15.857142857142858, 16.0, 16.142857142857142, 16.285714285714285, 16.428571428571427, 16.571428571428573, 16.714285714285715, 16.857142857142858, 17.0, 17.142857142857142, 17.285714285714285, 17.428571428571427, 17.571428571428573, 17.714285714285715, 17.857142857142858, 18.0, 18.142857142857142, 18.285714285714285, 18.428571428571427, 18.571428571428573, 18.714285714285715, 18.857142857142858, 19.0, 19.142857142857142, 19.285714285714285, 19.428571428571427, 19.571428571428573, 19.714285714285715, 19.857142857142858, 20.0, 20.125, 20.25, 20.375, 20.5, 20.625, 20.75, 20.875, 21.0, 21.125, 21.25, 21.375, 21.5, 21.625, 21.75, 21.875, 22.0, 22.142857142857142, 22.285714285714285, 22.428571428571427, 22.571428571428573, 22.714285714285715, 22.857142857142858, 23.0, 23.142857142857142, 23.285714285714285, 23.428571428571427, 23.571428571428573, 23.714285714285715, 23.857142857142858, 24.0, 24.166666666666668, 24.333333333333332, 24.5, 24.666666666666668, 24.833333333333332], [-144.036, -13.790000000000001, -13.737, 122.754, -66.398, 31.577, 2.231, -24.664, 28.261, 0.28400000000000003, -36.56, -28.349, 48.835, 9.362, -3.45, 70.141, -21.434, 14.82, -7.15, 5.503, -3.1510000000000002, 19.615000000000002, -37.542, 37.142, -77.187, -13.869, 77.778, 28.214000000000002, -209.435, -44.263, 92.675, 173.606, -70.128, -22.579, 17.791, -6.63, 25.718, -41.878, 53.799, 9.335, -26.023, 18.444, 63.755, -8.517, 5.2540000000000004, -5.954, 9.551, -5.4510000000000005, -29.493000000000002, 36.647, -52.591, 51.495000000000005, -48.731, 1.0150000000000001, -23.6, -3.77, -9.625, -5.4670000000000005, -68.671, 95.393, -62.251000000000005, 56.047000000000004, -59.108000000000004, 68.081, -49.556000000000004, 29.952, -8.473, 3.225, -5.556, -80.529, 58.230000000000004, 15.281, -158.66400000000002, -40.713, 5.2170000000000005, 3.318, 41.133, -54.32, 4.988, 18.864, 11.423, -20.661, 21.778, -17.285, 27.321, 0.708, -6.828, -137.514, 116.626, -6.855, 17.827, -3.508, 11.786, 6.365, 0.353, -0.934, -8.204, -5.18, 14.941, -29.801000000000002, 30.563000000000002, -9.965, -49.22, 82.158, -27.42, 22.347, -6.756, -9.127, 9.927, -14.251, 14.278, -7.242, 12.457, -44.276, 50.209, -36.062, -9.121, 45.864000000000004, 14.941, -27.25, 10.852, -10.11, -33.233000000000004, 2.839, -9.967, -6.089, -53.326, -28.101, 2.907, -37.004, -2.206, 8.992, 13.58, -25.542, -16.332, 7.6370000000000005, -0.069, -29.122, 32.791000000000004, -20.453, 30.197, -45.615, 36.533, 74.47, 68.377, -22.557000000000002, -31.576, 134.472, -45.46, -0.8290000000000001, -40.115, 24.439, 20.487000000000002, -31.29, 19.527, -11.775, 16.457, -38.495, 9.553, 0.089, -0.045, -4.825, 11.782, 25.691, -10.461, -18.152, -12.304, 95.417, -138.734, 30.436, 96.265, -48.722, 40.836, 0.248]}} ("Cluster"), "Tune X(from BPM)"=w207, "Tune Y(from BPM)"=w206, "date (last kicker ON)"=w213, "time string (last kicker ON)"=w212, "date"=w235, "time string"=w234, "Mode"=w318, "Beam Current(mA"=w317, "Beam Lifetime(min)"=w316, "Beamsize X(um)"=w315, "Beamsize Y(um)"=w314, "NuX(from BBF)"=w313, "NuY(from BBF)"=w312, "Bucket Start"=w311, "Bucket Last"=w310, "Bucket Step"=w309, "BR inj. sep.(V)"=w308, "BR inj. kicker(kV)"=w307, "BR ext. kicker1(kV)"=w306, "BR ext. kicker2(kV)"=w305, "BR ext. sep.1(V)"=w304, "BR ext. sep.2(V)"=w303, "SR inj. sep.1(V)"=w302, "SR inj. sep.2(V)"=w301, "SR kicker1(kV)"=w300, "SR kicker2(kV)"=w299, "SR kicker3(kV)"=w298, "SR kicker4(kV)"=w297, "Gun mode"=w296, "Grid volt.(V)(S)"=w295, "Gun volt.(V)(S)"=w294, "Mod.3 HV(kV)(S)"=w293, "Width count"=w292, "2ns step"=w291, "10ps delay"=w290, "RF2 remote"=w289, "RF2 OP mode"=w288, "RF2 phase.(S)"=w211, "RF Freq.(s)"=w287, "RF2 gap volt.(S)"=w210, "RF3 remote"=w286, "RF3 OP mode"=w285, "RF3 phase.(S)"=w284, "RF3 gap volt.(S)"=w283, "BR"=w282, "BTS"=w281, "Linac"=w279, "LTB"=w278, "SR"=w280, "SR Fill Pattern"=w277, "IU22-05 Hutch Enable"=w160, "IU22A-09M Hutch Enable"=w156, "IUT22-21M Hutch Enable"=w140, "IU22-23M Hutch Enable"=w123, "IU22A-25M Hutch Enable"=w122, "EPU48A-41M Hutch Enable"=w104, "EPU46-45M Hutch Enable"=w103, "EPU46-45 FE Enable"=w105, "EPU48A-41 FE Enable"=w106, "IU22A-25 FE Enable"=w124, "IU22-23 FE Enable"=w125, "IUT22-21 FE Enable"=w143, "IU22A-09 FE Enable"=w155, "IU22-05 FE Enable"=w161, "IU22-05gap(R)"=w276, "IU22A-09gap(R)"=w275, "IU22B-09gap(R)"=w274, "IUT22-21gap(R)"=w273, "IU22-23gap(R)"=w272, "IU22A-25gap(R)"=w271, "IU22B-25gap(R)"=w270, "EPU48A-41gap(R)"=w269, "EPU48A-41phase(R)"=w268, "EPU48B-41gap(R)"=w267, "EPU48B-41phase(R)"=w266, "EPU46-45gap(R)"=w265, "EPU46-45phase(R)"=w264, "Taper"=w208, "phase shifter"=w263, "05XBPMX 1"=w262, "09XBPMX 1"=w261, "21XBPMX 1"=w260, "23XBPMX 1"=w259, "25XBPMX 1"=w258, "41XBPMX 1"=w257, "45XBPMX 1"=w256, "05XBPMY 1"=w255, "09XBPMY 1"=w254, "21XBPMY 1"=w253, "23XBPMY 1"=w252, "25XBPMY 1"=w251, "41XBPMY 1"=w250, "45XBPMY 1"=w249, "IU22-05M"=w248, "IU22A-09M"=w247, "IU22B-09M"=w246, "IUT22-21M"=w245, "IU22-23M"=w244, "IU22A-25M"=w243, "IU22B-25M"=w242, "EPU48A-41gM"=w241, "EPU48B-41gM"=w240, "EPU46-45gM"=w239, "EPU48A-41pM"=w238, "EPU48B-41pM"=w237, "EPU46-45pM"=w236, "BPMX Graph 2"=w64, "BPMY Graph 2"=w63, "Radio Buttons 2"=enum32{"absolute", "different with"}."absolute", "FOFB H"=w219, "FOFB V"=w218, "BBF H"=w217, "BBF V"=w216, "Orbit ILK(P)"=w215, "05XBPMX 2"=w150, "05XBPMY 2"=w149, "09XBPMX 2"=w148, "09XBPMY 2"=w147, "21XBPMX 2"=w132, "21XBPMY 2"=w131, "23XBPMX 2"=w130, "23XBPMY 2"=w129, "25XBPMX 2"=w112, "25XBPMY 2"=w111, "41XBPMX 2"=w110, "41XBPMY 2"=w109, "45XBPMX 2"=w108, "45XBPMY 2"=w107, "05 mode"=w86, "09A mode"=w85, "09B mode"=w84, "21 mode"=w83, "23 mode"=w82, "25A mode"=w81, "25B mode"=w80, "41A mode"=w79, "41B mode"=w78, "46 mode"=w77, "BeamCurrent History"=w73, "RF FB"=w69) -> (→"Cluster":T1)
  }
  n313 = while {
    tunnel: w5 -> [_]
    shift-right: [w996] -> _
    shift-left: string[] [] -> [w993]
    shift-right: [w985] -> _
    shift-left: string[][] [] -> [w988]
    tunnel: w15 -> [w983]
    i -> [w981]
    stop <- w982 stop-if-true
    n314 = flat-sequence {
      tunnel: [w1009] -> w997
      tunnel: [w1008] -> w994
      tunnel: w993 -> [w1008]
      tunnel: [w1007] -> w984
      tunnel: w983 -> [w1007]
      tunnel: [w1019] -> w998
      tunnel: w997 -> [w1019]
      tunnel: [w1017] -> w995
      tunnel: w994 -> [w1018]
      tunnel: [w1011] -> w992
      tunnel: w984 -> [w1010]
      tunnel: w998 -> [w1042]
      tunnel: [w1040] -> w996
      tunnel: w995 -> [w1040]
      tunnel: w992 -> [w1039]
      tunnel: [w1039] -> w987
      frame #0 {
        n315 = Tick Count (ms)() -> (millisecond timer value=w1009:u32)
      }
      frame #1 {
        n316 = Get Date/Time In Seconds() -> (seconds since 1Jan1904=w1014:timestamp)
        n317 = To Double Precision Float(number=w1014) -> (double precision float=w1013:dbl)
        n318 = Format Date/Time String(time format string (%c)="%Y/%m/%d %H:%M:%S", seconds (now)=w1014) -> (date/time string=w1015:string)  [unwired: 1 in]
        n319 = Number To Fractional String(number=w1013) -> (F-format string=w1012:string)  [unwired: 3 in]
        n320 = call-poly <userlib>:"CaLabGet.vi"("PV Names"=w1010) -> ("1rst Value (string)"=w1017:string[])  [unwired: 8 in, 6 out]
        n321 = for {
          tunnel: w1018 -> [w1021] mode=indexing
          tunnel: w1017 -> [w1020] mode=indexing
          tunnel: w1010 -> [w1029] mode=indexing
          tunnel: w1015 -> [w1028]
          tunnel: [w1027] -> w1011 mode=indexing if=w1025
          tunnel: w1012 -> [w1026]
          i -> [w1024]
          n322 = Greater Or Equal?(x=w1024, y=1) -> (x >= y?=w1022:bool)
          n323 = case shown="True" w1022 {
            tunnel: w1029 -> [_ w1038]
            tunnel: w1021 -> [_ w1037]
            tunnel: w1020 -> [_ w1036]
            tunnel: w1028 -> [_ w1035]
            tunnel: [string[] [] w1034] -> w1027
            tunnel: w1026 -> [_ w1033]
            tunnel: [FALSE w1032] -> w1025
            frame False {
            }
            frame True {
              n324 = Not Equal?(x=w1037, y=w1036) -> (x != y?=w1032:bool)
              n325 = Build Array(w1035, w1038, w1037, w1036, w1033) -> (w1034:string[])
            }
          }
        }
      }
      frame #2 {
        n326 = Tick Count (ms)() -> (millisecond timer value=w1043:u32)
        n327 = Subtract(x=w1043, y=w1042) -> (x-y=→"dT":u32)
      }
    }
    n328 = while {
      i -> [w1000]
      stop <- w1004 stop-if-true
      # "每60秒，表示法:\n100 600"
      # "每十秒，表示法:\n100 100"
      n329 = local read "stop"() -> (w1003:bool)
      n330 = Multiply(x="Check period", y=10) -> (x*y=w1001:i32)
      n331 = Greater Or Equal?(x=w1000, y=w1001) -> (x >= y?=w1005:bool)
      n332 = Wait Until Next ms Multiple(millisecond multiple=u32 99) -> ()  [unwired: 1 out]
      n333 = Or(x=w1005, y=w1003) -> (x .or. y?=w1004:bool)
    }
    n334 = Index Array(array=w987, index (row)=0) -> (element=w990:string[])  [unwired: 1 in]
    n335 = Array Size(array=w990) -> (size(s)=w980:i32)
    "EVENTs" <- w980
    n336 = Greater?(x=w980, y=0) -> (0:→"x > y?":bool)
    n337 = Build Array (concatenate)(w988, w987) -> (w985:string[][])
    "Diff list" <- w985
    n338 = local read "stop"() -> (w982:bool)
    "check loop" <- w981
  }
  n339 = local write "stop"(FALSE ("stop")) -> ()
